vi "VIP_Phase_4.vi"() -> ()   [LabVIEW 2024]
uses:
  <vilib>/DAQmx/read.llb/DAQmx Read (Digital 1D Bool 1Chan 1Samp).vi
  <vilib>/Utility/file.llb/Write To Spreadsheet File (DBL).vi
  <vilib>/DAQmx/create/channels.llb/DAQmx Create Channel (DI-Digital Input).vi
  <vilib>/DAQmx/miscellaneous.llb/DAQmx Fill In Error Info.vi
  <vilib>/ptbypt/NI_PtbyPt.lvlib
panel:
  out "fault # 4":dbl
  out "fault # 3":dbl
  out "fault # 2":dbl
  out "fault # 1":dbl
  in  "LED 4":tag="Dev1/port0/line23"
  in  "LED 3":tag="Dev1/port0/line22"
  in  "LED 2":tag="Dev1/port0/line21"
  out "LED 4 (i)":dbl
  out "LED 3 (i)":dbl
  out "LED 2 (i)":dbl
  in  "LED 1":tag="Dev1/port0/line20"
  out "LED 1(i)":dbl
  out "4.2":bool
  out "mouse 4.2":cluster{"Y":dbl[], "Y":dbl[]}[](graph)
  out "mouse 4.1":cluster{"Y":dbl[], "Y":dbl[]}[](graph)
  in  "fake 4.2":bool
  in  "fake 4.1":bool
  out "ratio 4.2R":cluster{"Y":dbl[], "Y":dbl[]}[](graph)=[{"Y"=[2.5380001068115234, 12.063000202178955, 24.592000007629395, 36.145999908447266, 48.69600009918213, 58.23899984359741, 67.79099988937378, 81.40899991989136, 91.96199989318848, 99.9980001449585], "Y"=[0.0, 0.0, 0.0, 0.0, 0.0, 0.0, 0.0, 0.0, 0.0, 0.0]}]
  out "ratio 4.1L":cluster{"Y":dbl[], "Y":dbl[]}[](graph)=[{"Y"=[2.5380001068115234, 12.063000202178955, 24.592000007629395, 36.145999908447266, 48.69600009918213, 58.23899984359741, 67.79099988937378, 81.40899991989136, 91.96199989318848, 99.9980001449585], "Y"=[0.0, 0.0, 0.0, 0.0, 0.0, 0.0, 0.0, 0.0, 0.0, 0.0]}]
  out "ratio 4.2R":dbl
  out "ratio 4.1L":dbl
  in  "water dur (ms) 4.2":dbl=11.5
  in  "water port 4.2":tag="Dev1/port2/line0"
  out "Mouse path 4":path=path "C:/Users/Administrator/Documents/LabVIEW Data/a-lick-20140707-145848"
  out "Mouse file 4":string="a-lick-20140707-145848"
  in  "Mouse ID 4":string="VIP_4"
  in  "water dur (ms) 4.1":dbl=9.0
  in  "water port 4.1":tag="Dev1/port1/line7"
  in  "free water 4.2":bool
  in  "free water 4.1":bool
  out "4.1":bool
  out "state 4.2":enum16{"waiting", "sound", "ITI"}(ring)=enum."ITI"
  out "state 4.1":enum16{"waiting", "sound", "ITI"}(ring)=enum."ITI"
  out "water # 4.1L":dbl
  out "water # 4.2R":dbl
  out "lick # 4.2R":dbl
  out "lick # 4.1L":dbl
  out "last water 4.2R":dbl
  out "last water 4.1L":dbl
  out "mistake # 4.2R":dbl
  out "mistake # 4.1L":dbl
  out "ratio 3.2R":cluster{"Y":dbl[], "Y":dbl[]}[](graph)=[{"Y"=[2.5380001068115234, 12.063000202178955, 24.592000007629395, 36.145999908447266, 48.69600009918213, 58.23899984359741, 67.79099988937378, 81.40899991989136, 91.96199989318848, 99.9980001449585], "Y"=[0.0, 0.0, 0.0, 0.0, 0.0, 0.0, 0.0, 0.0, 0.0, 0.0]}]
  out "ratio 3.1L":cluster{"Y":dbl[], "Y":dbl[]}[](graph)=[{"Y"=[2.5380001068115234, 12.063000202178955, 24.592000007629395, 36.145999908447266, 48.69600009918213, 58.23899984359741, 67.79099988937378, 81.40899991989136, 91.96199989318848, 99.9980001449585], "Y"=[0.0, 0.0, 0.0, 0.0, 0.0, 0.0, 0.0, 0.0, 0.0, 0.0]}]
  in  "free water 3.2":bool
  in  "free water 3.1":bool
  in  "water dur (ms) 3. 2":dbl=29.0
  in  "water dur (ms) 3.1":dbl=29.0
  out "mouse 3.2":cluster{"Y":dbl[], "Y":dbl[]}[](graph)
  out "mouse 3.1":cluster{"Y":dbl[], "Y":dbl[]}[](graph)
  in  "fake 3.2":bool
  in  "fake 3.1":bool
  out "last water 3.2R":dbl
  out "last water 3.1L":dbl
  out "mistake # 3.2R":dbl
  out "mistake # 3.1L":dbl
  out "water # 3.2R":dbl
  out "water # 3.1L":dbl
  out "lick # 3.2R":dbl
  out "lick # 3.1L":dbl
  out "ratio 3.2R":dbl
  out "ratio 3.1L":dbl
  in  "water port 3.2":tag="Dev1/port1/line6"
  out "3.2":bool
  out "state 3.2":enum16{"waiting", "sound", "ITI"}(ring)=enum."ITI"
  out "state 3.1":enum16{"waiting", "sound", "ITI"}(ring)=enum."ITI"
  out "3.1":bool
  out "Mouse path 3":path=path "C:/Users/Administrator/Documents/LabVIEW Data/a-lick-20140707-145848"
  out "Mouse file 3":string="a-lick-20140707-145848"
  in  "water port 3.1":tag="Dev1/port1/line5"
  in  "Mouse ID 3":string="VIP_3"
  out "ratio 2.2R":cluster{"Y":dbl[], "Y":dbl[]}[](graph)=[{"Y"=[2.5380001068115234, 12.063000202178955, 24.592000007629395, 36.145999908447266, 48.69600009918213, 58.23899984359741, 67.79099988937378, 81.40899991989136, 91.96199989318848, 99.9980001449585], "Y"=[0.0, 0.0, 0.0, 0.0, 0.0, 0.0, 0.0, 0.0, 0.0, 0.0]}]
  out "ratio 2.1L":cluster{"Y":dbl[], "Y":dbl[]}[](graph)=[{"Y"=[2.5380001068115234, 12.063000202178955, 24.592000007629395, 36.145999908447266, 48.69600009918213, 58.23899984359741, 67.79099988937378, 81.40899991989136, 91.96199989318848, 99.9980001449585], "Y"=[0.0, 0.0, 0.0, 0.0, 0.0, 0.0, 0.0, 0.0, 0.0, 0.0]}]
  out "ratio 1.2R":cluster{"Y":dbl[], "Y":dbl[]}[](graph)=[{"Y"=[2.5380001068115234, 12.063000202178955, 24.592000007629395, 36.145999908447266, 48.69600009918213, 58.23899984359741, 67.79099988937378, 81.40899991989136, 91.96199989318848, 99.9980001449585], "Y"=[0.0, 0.0, 0.0, 0.0, 0.0, 0.0, 0.0, 0.0, 0.0, 0.0]}]
  out "mouse 2.2":cluster{"Y":dbl[], "Y":dbl[]}[](graph)
  out "mouse 2.1":cluster{"Y":dbl[], "Y":dbl[]}[](graph)
  in  "free water 2.2":bool
  in  "free water 2.1":bool
  out "last water 2.2R":dbl
  out "last water 2.1L":dbl
  out "mistake # 2.2R":dbl
  out "mistake # 2.1L":dbl
  out "water # 2.2R":dbl
  out "water # 2.1L":dbl
  out "lick  #  2.2R":dbl
  out "lick  #  2.1L":dbl
  out "2.1":bool
  out "ratio 2.2R":dbl
  out "ratio 2.1L":dbl
  out "2.2":bool
  in  "fake 2.2":bool
  in  "fake 2.1":bool
  out "Mouse path 2":path=path "C:/Users/Administrator/Documents/LabVIEW Data/a-lick-20140707-145848"
  out "Mouse file 2":string="a-lick-20140707-145848"
  in  "Mouse ID 2":string="VIP_2"
  in  "water dur (ms) 2.2":dbl=27.5
  in  "water dur (ms) 2.1":dbl=36.5
  in  "water port 2.2":tag="Dev1/port1/line4"
  in  "water port 2.1":tag="Dev1/port1/line3"
  out "state 2.2":enum16{"waiting", "sound", "ITI"}(ring)=enum."ITI"
  out "state 2.1":enum16{"waiting", "sound", "ITI"}(ring)=enum."ITI"
  in  "sound port 2":tag="Dev1/ao1"
  out "time (s)":dbl=103.38100004196167
  out "mistake # 1.2R":dbl
  out "mistake # 1.1L":dbl
  in  "water dur (ms) 1.1":dbl=36.0
  in  "water port 1.1":tag="Dev1/port1/line1"
  in  "water dur (ms) 1.2":dbl=28.0
  in  "water port 1.2":tag="Dev1/port1/line2"
  out "1.1":bool
  out "1.2":bool
  out "state 1.2":enum16{"waiting", "sound", "ITI"}(ring)=enum."ITI"
  out "lick # 1.2R":dbl
  out "water # 1.2R":dbl
  in  "fake 1.2":bool
  in  "free water 1.2":bool
  out "mouse 1.2":cluster{"Y":dbl[], "Y":dbl[]}[](graph)
  out "ratio 1.2R":dbl
  out "last water 1.2R":dbl
  out "ratio 1.1L":dbl
  out "ratio 1.1L":cluster{"Y":dbl[], "Y":dbl[]}[](graph)=[{"Y"=[2.5380001068115234, 12.063000202178955, 24.592000007629395, 36.145999908447266, 48.69600009918213, 58.23899984359741, 67.79099988937378, 81.40899991989136, 91.96199989318848, 99.9980001449585], "Y"=[0.0, 0.0, 0.0, 0.0, 0.0, 0.0, 0.0, 0.0, 0.0, 0.0]}]
  in  "free water 1.1":bool
  out "Right Speaker":dbl=5.0
  out "Left Speaker":dbl=5.0
  in  "sound file 2":path=path "C:/Users/cvm-gritton-lab/Documents/Lab View Programs/Lab View Programs/LabVIEW VIs/Tones/New_Phase_2_Sounds/200k_target2.wav"
  in  "ITI max (ms)":dbl=7000.0
  in  "ITI min (ms)":dbl=5000.0
  in  "reaction dur (ms)":dbl=1750.0
  in  "sound dur (ms)":dbl=3000.0
  in  "sound file 1":path=path "C:/Users/cvm-gritton-lab/Documents/Lab View Programs/Lab View Programs/LabVIEW VIs/Tones/New_Phase_2_Sounds/200k_target1.wav"
  in  "sound port 1":tag="Dev1/ao0"
  out "trial state":T1(ring)=enum."ITI"
  out "trial #":dbl=10.0
  out "current sound":dbl=1.0
  out "next sound":dbl[](array[numeric])
  out "Mouse path 1":path=path "C:/Users/Administrator/Documents/LabVIEW Data/a-lick-20140707-145848"
  in  "fake 1.1":bool
  out "mouse 1.1":cluster{"Y":dbl[], "Y":dbl[]}[](graph)
  out "ITI (s)":dbl=6.5
  out "last water 1.1L":dbl
  out "state 1.1":enum16{"waiting", "sound", "ITI"}(ring)=enum."ITI"
  out "water # 1.1L":dbl
  out "lick # 1.1L":dbl
  out "Mouse file 1":string="a-lick-20140707-145848"
  out "data folder":path=path "C:/LabVIEW VIs/LabVIEW data"
  in  "Mouse ID 1":string="VIP_1"
  in  "lick port":tag="Dev1/port0/line0:7"
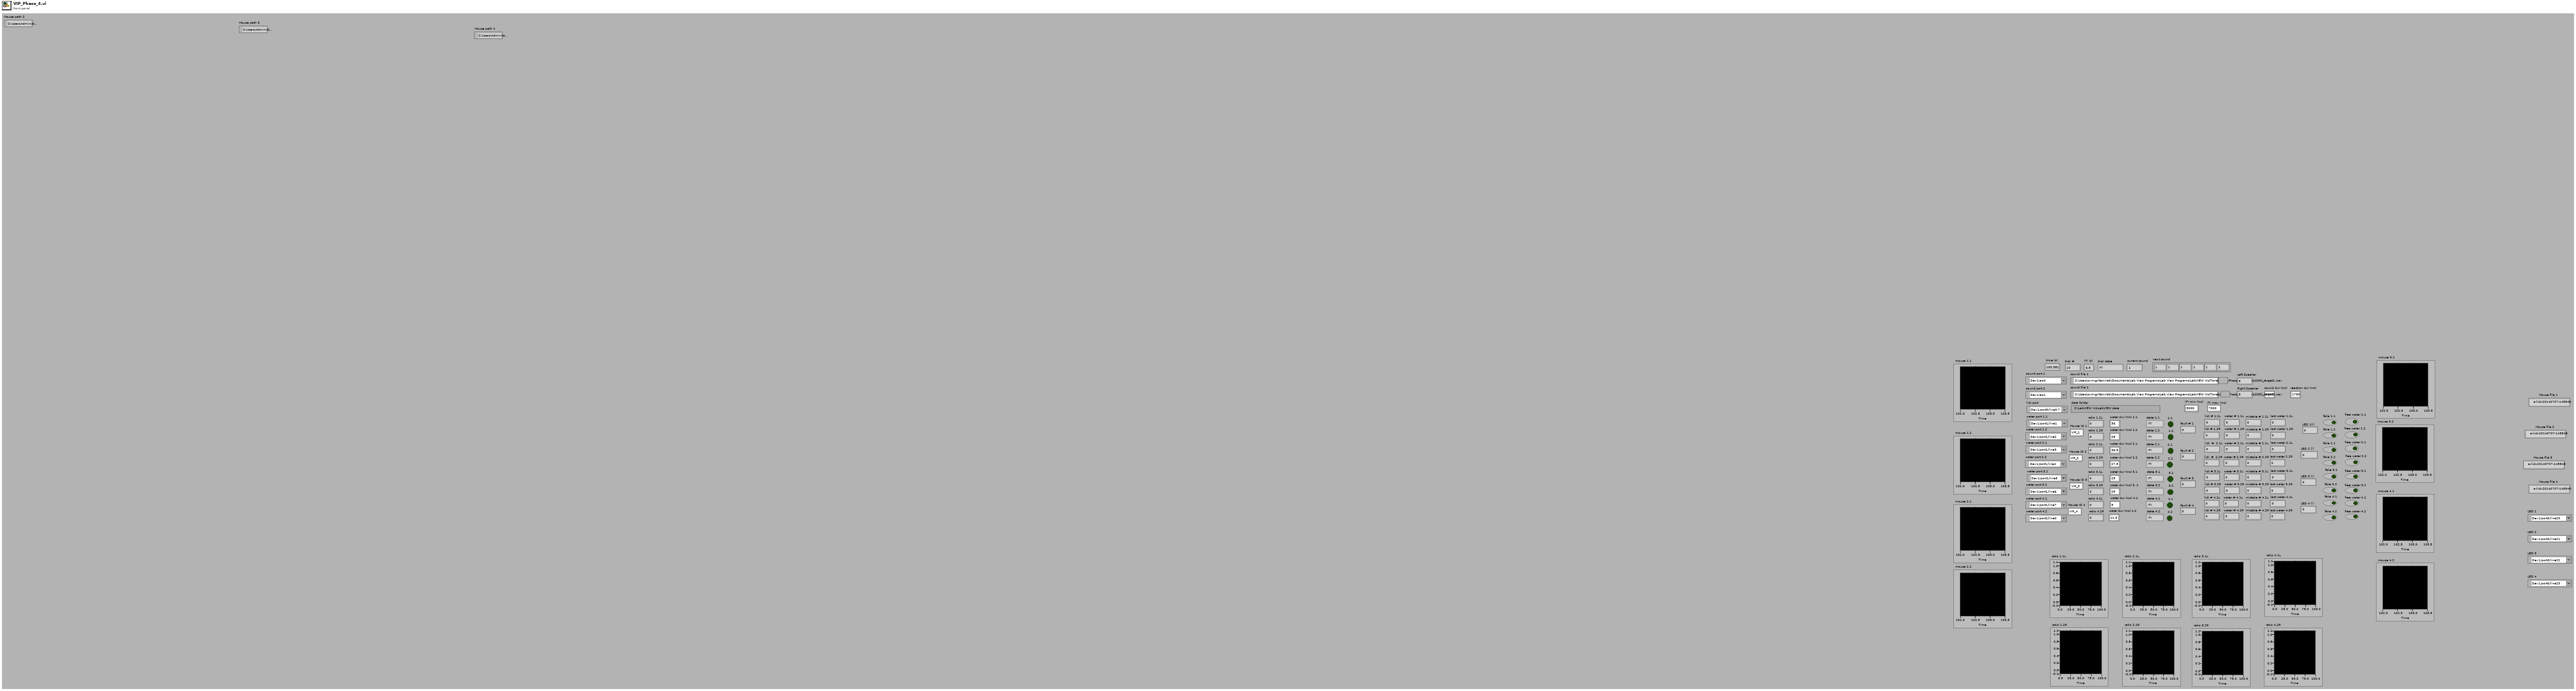
[diagram p1: front panel]
types:
  T1 = enum16{"prepare", "sound", "reaction window", "ITI", "free water", "graph", "data collection"}
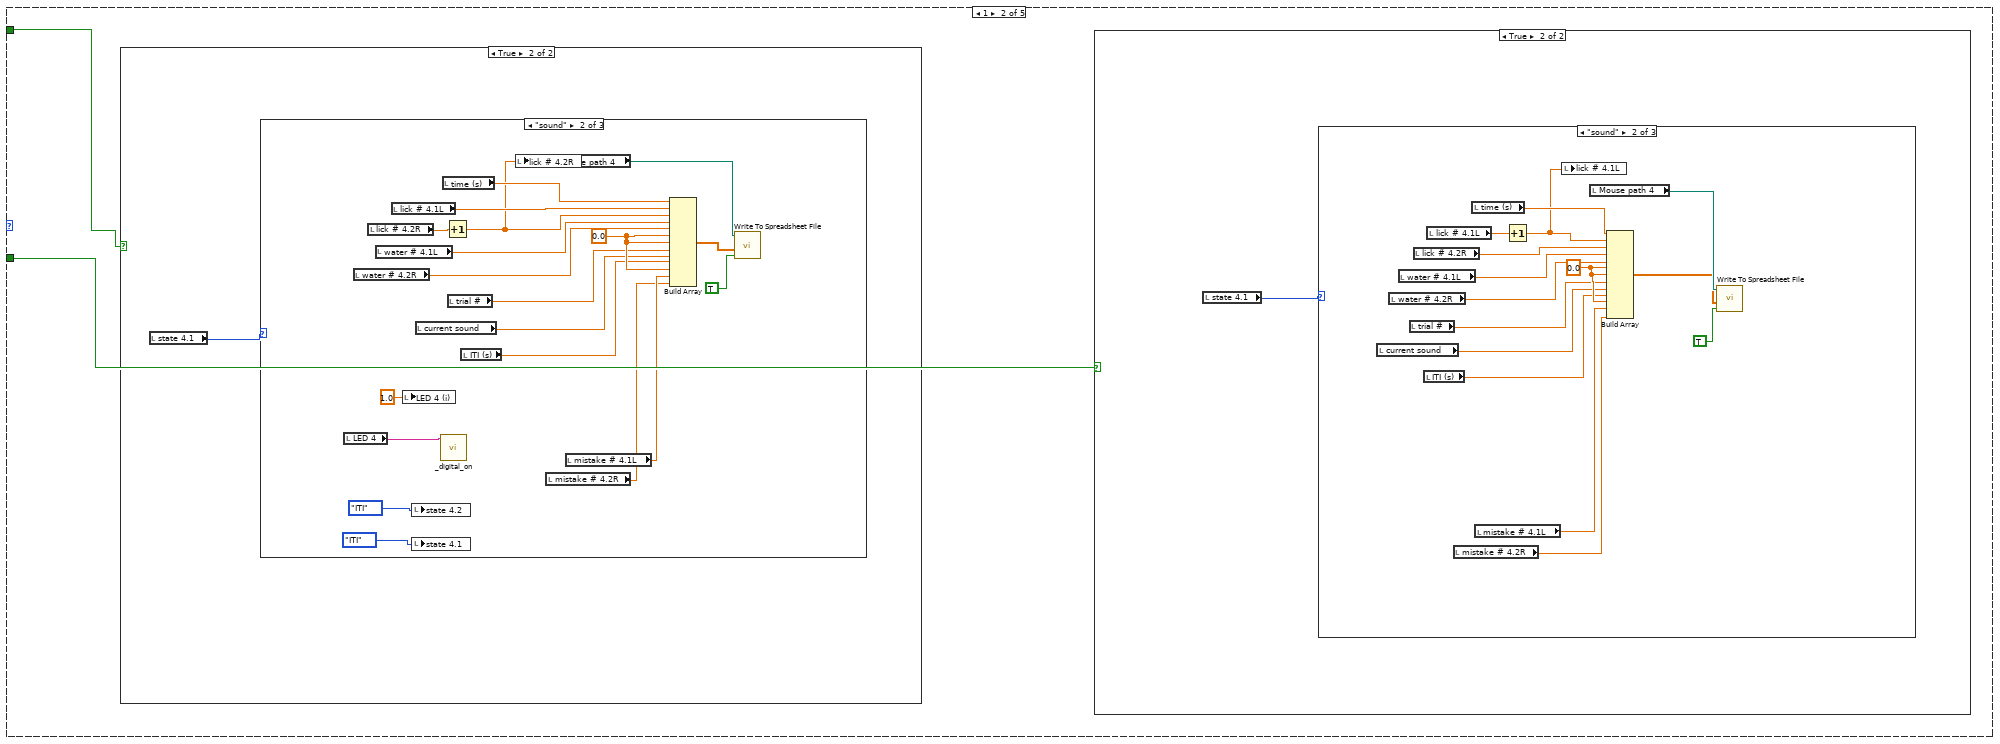
[diagram p3: hidden frame]
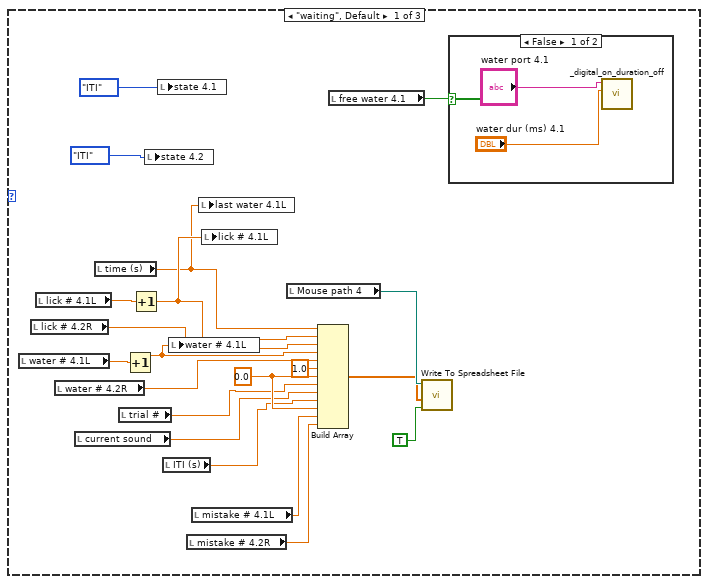
[diagram p5: hidden frame]
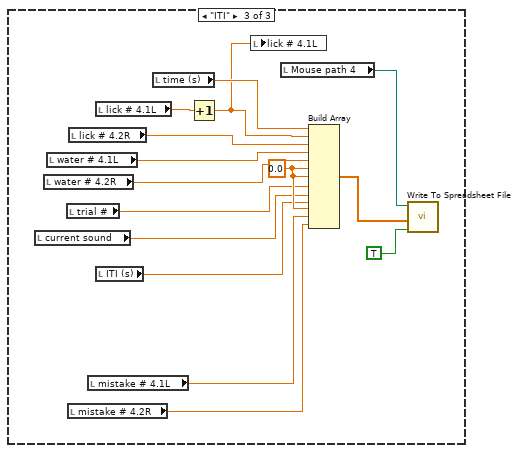
[diagram p7: hidden frame]
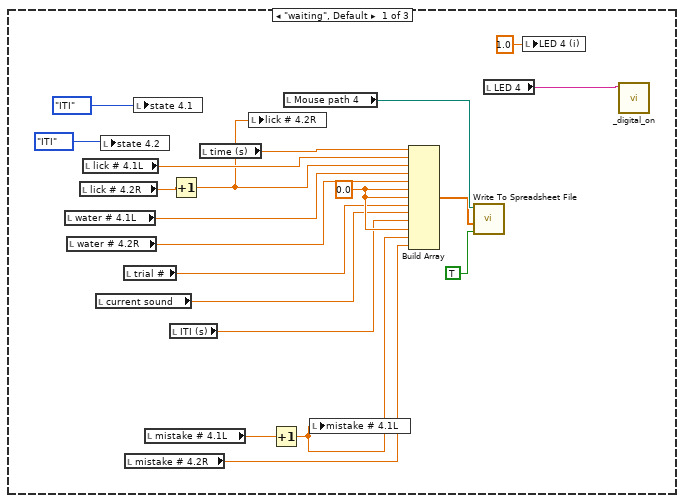
[diagram p9: hidden frame]
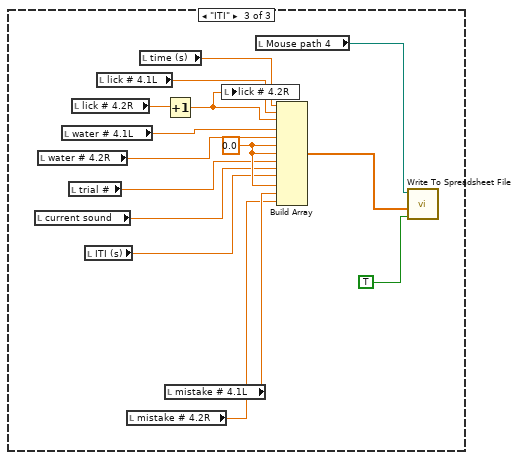
[diagram p10: hidden frame]
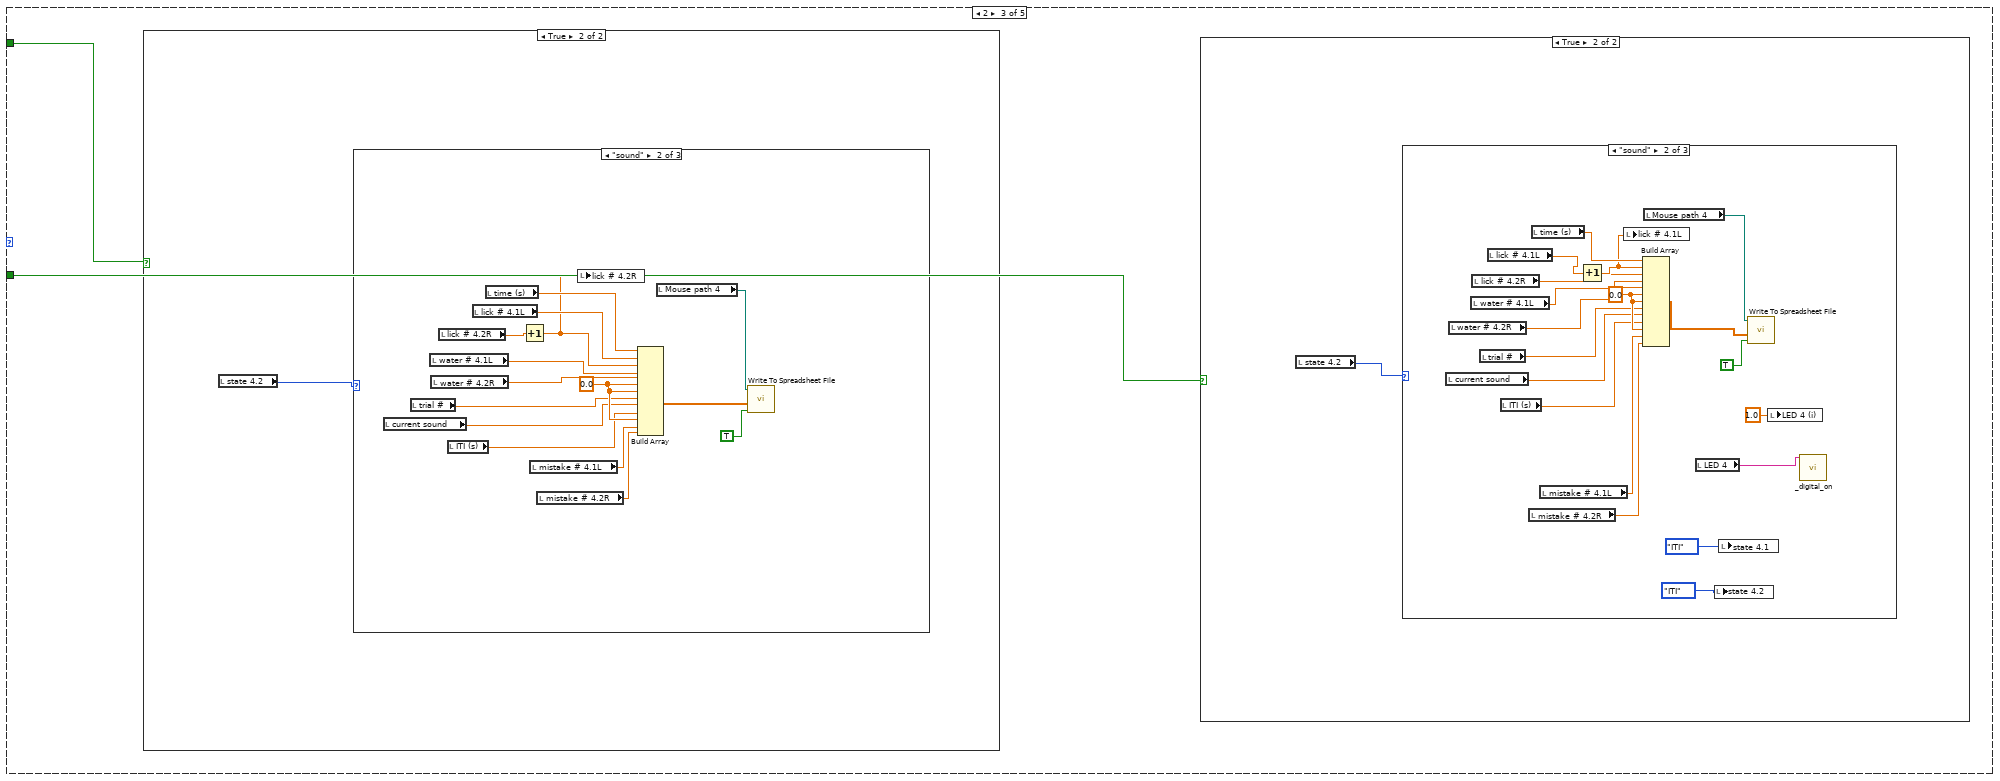
[diagram p11: hidden frame]
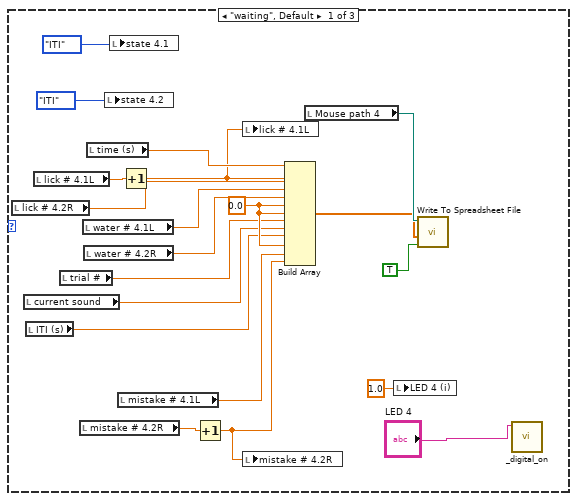
[diagram p13: hidden frame]
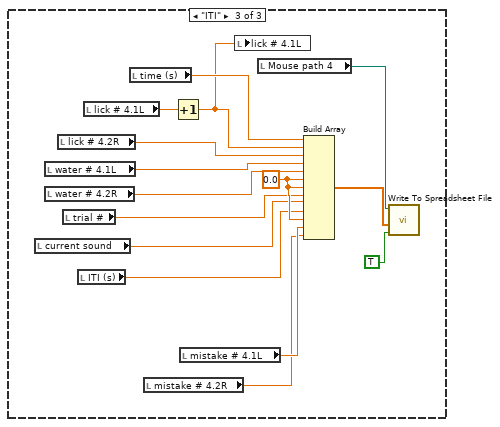
[diagram p14: hidden frame]
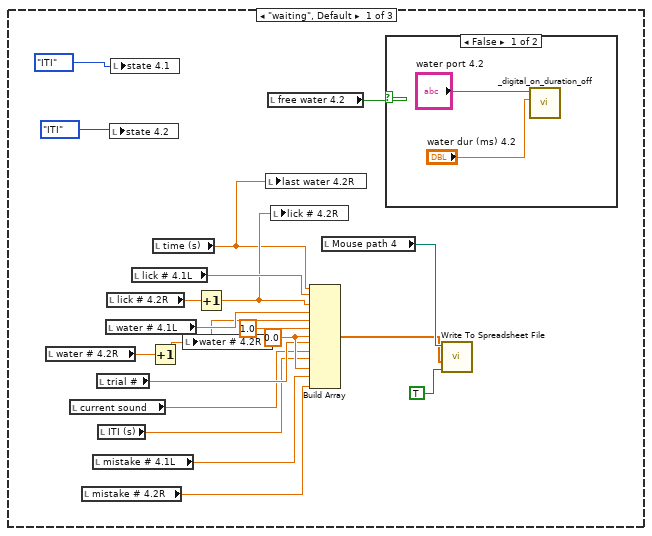
[diagram p16: hidden frame]
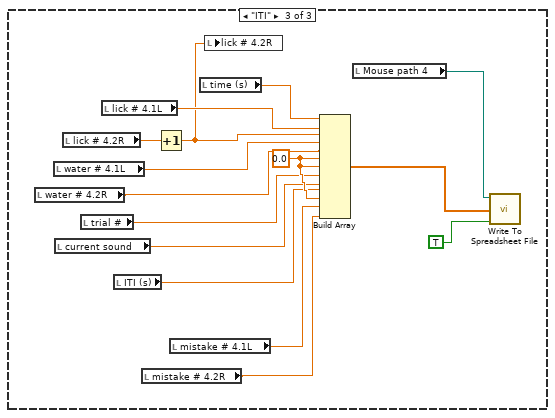
[diagram p18: hidden frame]
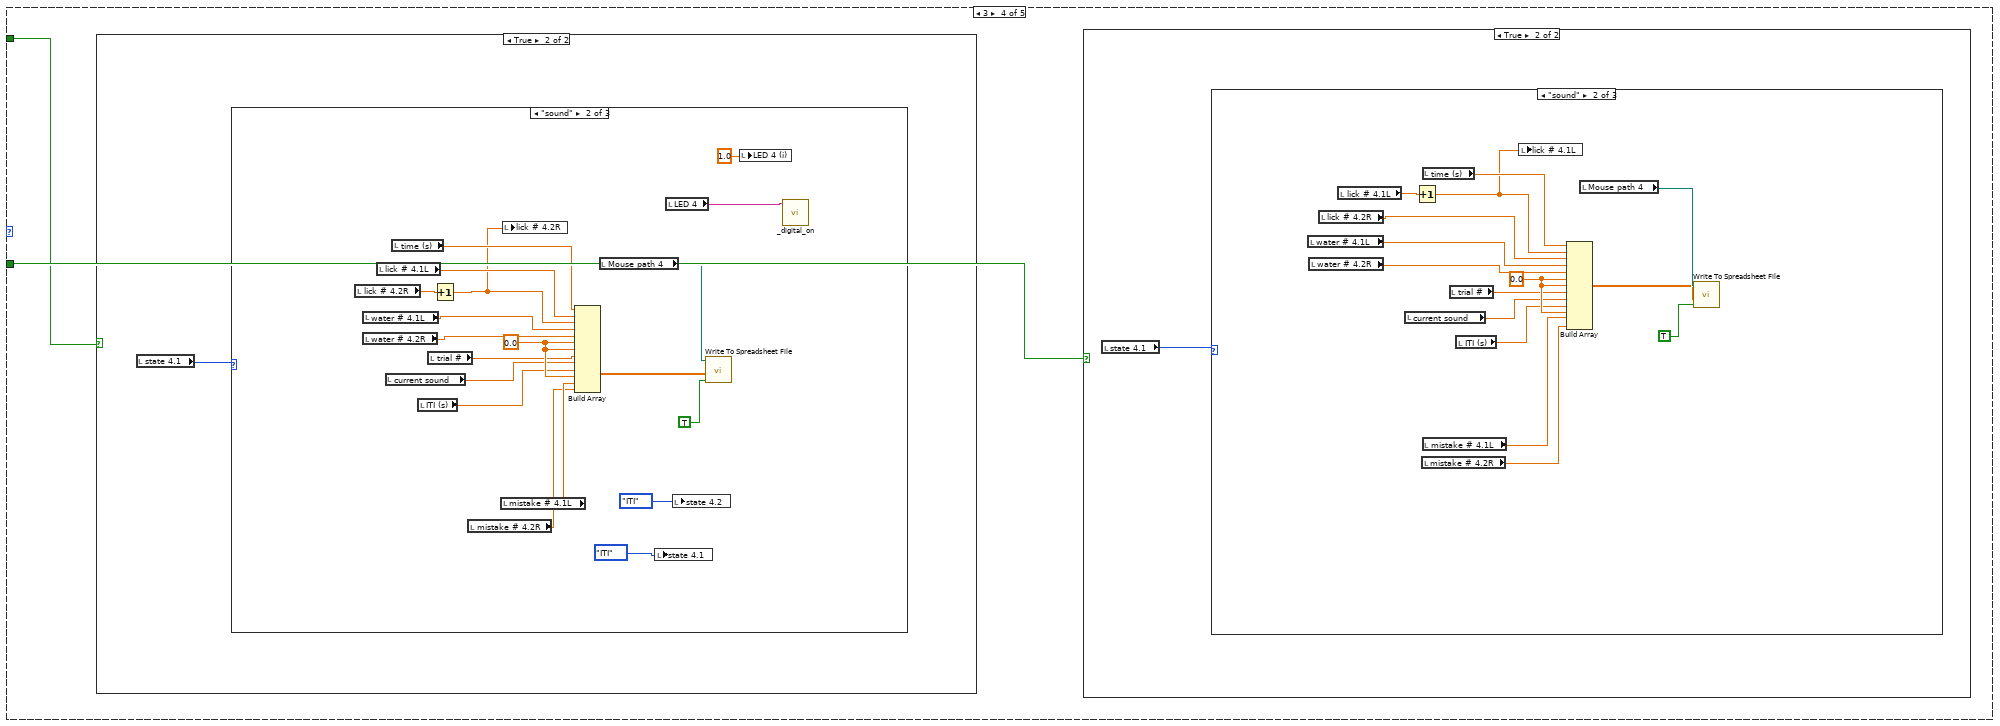
[diagram p19: hidden frame]
diagram:
  n1 = flat-sequence {
    frame #0 {
      w1 = 0.0 ("fault # 2")
      w2 = 0.0 ("LED 1 (R)")
      w12 = 0.0 ("mistake # 1.1L")
      w4 = 0
      w22 = 0
      w11 = 0
      w3 = 0
      w10 = enum16{"waiting", "sound", "ITI"}."sound"
      n2 = Get Date/Time In Seconds() -> (seconds since 1Jan1904=w24:timestamp)
      n3 = call <vilib>:"Dflt Data Dir.vi"() -> ("App:Default Data Directory"=w6:path)
      "data folder" <- w6
      n4 = Format Date/Time String(time format string (%c)="%m%d%Y-%H%M%S-", seconds (now)=w24) -> (date/time string=w9:string)  [unwired: 1 in]
      n5 = Concatenate Strings(w9, "Mouse ID 1") -> (w27:string)
      "Mouse file 1" <- w27
      n6 = Concatenate Strings(w9, "Mouse ID 4") -> (w7:string)
      "Mouse file 4" <- w7
      n7 = Concatenate Strings(w9, "Mouse ID 2") -> (w17:string)
      "Mouse file 2" <- w17
      n8 = Concatenate Strings(w9, "Mouse ID 3") -> (w14:string)
      "Mouse file 3" <- w14
      n9 = Build Path(base path=w6, name or relative path=w27) -> (appended path=→"Mouse path 1":path)
      n10 = Build Path(base path=w6, name or relative path=w17) -> (appended path=→"Mouse path 2":path)
      n11 = Build Path(base path=w6, name or relative path=w14) -> (appended path=→"Mouse path 3":path)
      n12 = Build Path(base path=w6, name or relative path=w7) -> (appended path=→"Mouse path 4":path)
      n13 = call "_array_shuffle.vi"("total number"=40, "input array"=i32[] [1, 2, 3, 4, 1, 2, 3, 4]) -> ("output array"=→"next sound":dbl[])  [unwired: 9 in]
      n14 = local write "time (s)"(w22) -> ()
      "water # 1.1L" <- w3
      "lick # 1.1L" <- w3
      "state 1.1" <- w10
      "last water 1.1L" <- w11
      "current sound" <- w22
      "trial #" <- w22
      "ITI (s)" <- w22
      "Left Speaker" <- w22
      "Right Speaker" <- w22
      "ratio 1.1L" <- w4
      "last water 1.2R" <- w11
      "ratio 1.2R" <- w4
      "water # 1.2R" <- w3
      "lick # 1.2R" <- w3
      "state 1.2" <- w10
      "mistake # 1.1L" <- w12
      "mistake # 1.2R" <- w12
      "state 2.1" <- w10
      "state 2.2" <- w10
      "ratio 2.1L" <- w4
      "ratio 2.2R" <- w4
      "lick  #  2.1L" <- w3
      "lick  #  2.2R" <- w3
      "water # 2.1L" <- w3
      "water # 2.2R" <- w3
      "mistake # 2.1L" <- w12
      "mistake # 2.2R" <- w12
      "last water 2.1L" <- w11
      "last water 2.2R" <- w11
      "state 3.1" <- w10
      "state 3.2" <- w10
      "ratio 3.1L" <- w4
      "ratio 3.2R" <- w4
      "lick # 3.1L" <- w3
      "lick # 3.2R" <- w3
      "water # 3.1L" <- w3
      "water # 3.2R" <- w3
      "mistake # 3.1L" <- w12
      "mistake # 3.2R" <- w12
      "last water 3.1L" <- w11
      "last water 3.2R" <- w11
      "mistake # 4.1L" <- w12
      "mistake # 4.2R" <- w12
      "last water 4.1L" <- w11
      "last water 4.2R" <- w11
      "lick # 4.1L" <- w3
      "lick # 4.2R" <- w3
      "water # 4.2R" <- w3
      "water # 4.1L" <- w3
      "state 4.1" <- w10
      "state 4.2" <- w10
      "ratio 4.1L" <- w4
      "ratio 4.2R" <- w4
      "LED 1(i)" <- w2
      "LED 2 (i)" <- w2
      "LED 3 (i)" <- w2
      "LED 4 (i)" <- w2
      "fault # 1" <- w1
      "fault # 2" <- w1
      "fault # 3" <- w1
      "fault # 4" <- w1
    }
    frame #1 {
      # "file format:\n1. time stamp\n2. lick #\n3. water #\n4. water triggered by lick?\n5. trial start?\n6. trial #\n7. trial sound\n8. trial ITI\n9. free water?"
      n15 = call-poly <vilib>:"DAQmx Create Virtual Channel.vi"("lines"="lick port") -> ("task out"=w29:refnum<k21>)  [unwired: 13 in, 1 out]
      n16 = call <vilib>:"DAQmx Start Task.vi"("task/channels in"=w29) -> ("task out"=w30:refnum<k21>)  [unwired: 13 in, 1 out]
      n17 = while {
        tunnel: w30 -> [w89]
        tunnel: [w88] -> w31
        shift-right: [w79] -> _
        shift-left: _ -> [w87]
        shift-right: [w84] -> _
        shift-left: _ -> [w85]
        stop <- FALSE stop-if-true
        n18 = call-poly <vilib>:"DAQmx Read.vi"("task/channels in"=w89) -> ("task out"=w88:refnum<k21>, "data"=w80:bool[])  [unwired: 12 in, 1 out]
        n19 = Build Array("fake 1.1", "fake 1.2", "fake 2.1", "fake 2.2", "fake 3.1", "fake 3.2", "fake 4.1", "fake 4.2") -> (w76:bool[])
        n20 = Or(x=w80, y=w76) -> (x .or. y?=w79:bool[])
        n21 = Index Array(array=w79) -> (element #1=w82:bool, element #2=w68:bool, element #3=w59:bool, element #4=w56:bool, element #5=w48:bool, element #6=w45:bool, element #7=w40:bool, element #8=w36:bool)  [unwired: 8 in]
        n22 = call "Collector1."("Signals"=w59) -> ("Collected Signals"=w60:dynamicdata)  [unwired: 9 in, 1 out]
        n23 = call "Collector1.2"("Signals"=w68) -> ("Collected Signals"=w67:dynamicdata)  [unwired: 9 in, 1 out]
        n24 = call "Collector1.7"("Signals"=w36) -> ("Collected Signals"=w38:dynamicdata)  [unwired: 9 in, 1 out]
        n25 = call "Collector1.3"("Signals"=w56) -> ("Collected Signals"=w57:dynamicdata)  [unwired: 9 in, 1 out]
        n26 = call "Collector1.6"("Signals"=w40) -> ("Collected Signals"=w41:dynamicdata)  [unwired: 9 in, 1 out]
        n27 = call "Collector1.1"("Signals"=w82) -> ("Collected Signals"=w69:dynamicdata)  [unwired: 9 in, 1 out]
        n28 = call "Collector1.5"("Signals"=w45) -> ("Collected Signals"=w46:dynamicdata)  [unwired: 9 in, 1 out]
        n29 = call "Collector1.4"("Signals"=w48) -> ("Collected Signals"=w49:dynamicdata)  [unwired: 9 in, 1 out]
        n30 = local read "time (s)"() -> (w83:dbl)
        n31 = call "Collector"("Signals"=w83) -> ("Collected Signals"=w35:dynamicdata)  [unwired: 9 in, 1 out]
        n32 = call "Build XY Graph1.1"("Y Input"=w69, "X Input"=w35) -> ("XY Graph"=→"mouse 1.1":cluster{"Y":dbl[], "Y":dbl[]}[])  [unwired: 3 in, 6 out]
        n33 = call "Build XY Graph1."("Y Input"=w60, "X Input"=w35) -> ("XY Graph"=→"mouse 2.1":cluster{"Y":dbl[], "Y":dbl[]}[])  [unwired: 3 in, 6 out]
        n34 = call "Build XY Graph1.2"("Y Input"=w67, "X Input"=w35) -> ("XY Graph"=→"mouse 1.2":cluster{"Y":dbl[], "Y":dbl[]}[])  [unwired: 3 in, 6 out]
        n35 = call "Build XY Graph1.7"("Y Input"=w38, "X Input"=w35) -> ("XY Graph"=→"mouse 4.2":cluster{"Y":dbl[], "Y":dbl[]}[])  [unwired: 3 in, 6 out]
        n36 = call "Build XY Graph1.3"("Y Input"=w57, "X Input"=w35) -> ("XY Graph"=→"mouse 2.2":cluster{"Y":dbl[], "Y":dbl[]}[])  [unwired: 3 in, 6 out]
        n37 = call "Build XY Graph1.6"("Y Input"=w41, "X Input"=w35) -> ("XY Graph"=→"mouse 4.1":cluster{"Y":dbl[], "Y":dbl[]}[])  [unwired: 3 in, 6 out]
        n38 = call "Build XY Graph1.5"("Y Input"=w46, "X Input"=w35) -> ("XY Graph"=→"mouse 3.2":cluster{"Y":dbl[], "Y":dbl[]}[])  [unwired: 3 in, 6 out]
        n39 = call "Build XY Graph1.4"("Y Input"=w49, "X Input"=w35) -> ("XY Graph"=→"mouse 3.1":cluster{"Y":dbl[], "Y":dbl[]}[])  [unwired: 3 in, 6 out]
        n40 = Greater?(x=w79, y=w87) -> (0:w86:bool[])
        n41 = Index Array(array=w86) -> (element #1=w74:bool, element #2=w73:bool, element #3=w62:bool, element #4=w63:bool, element #5=w54:bool, element #6=w53:bool, element #7=w33:bool, element #8=w34:bool)  [unwired: 8 in]
        "1.2" <- w73
        "1.1" <- w74
        "2.2" <- w63
        "2.1" <- w62
        "3.1" <- w54
        "3.2" <- w53
        "4.1" <- w33
        "4.2" <- w34
        n42 = local read "current sound"() -> (w72:dbl)
        n43 = local read "current sound"() -> (w66:dbl)
        n44 = local read "current sound"() -> (w44:dbl)
        n45 = local read "current sound"() -> (w55:dbl)
        n46 = case shown="4" w55 {
          tunnel: w54 -> [_ w531 w642 w752 w862]
          tunnel: w53 -> [_ w530 w641 w751 w861]
          frame 0, Default {
          }
          frame 1 {
            n47 = case shown="True" w531 {
              frame False {
              }
              frame True {
                n48 = local read "state 3.1"() -> (w588:enum16{"waiting", "sound", "ITI"})
                n49 = case shown="\"waiting\", Default" w588 {
                  frame "waiting", Default {
                    w597 = 0.0 ("element")
                    n50 = local write "state 3.2"(enum16{"waiting", "sound", "ITI"}."ITI") -> ()
                    n51 = local read "free water 3.1"() -> (w608:bool)
                    n52 = local write "state 3.1"(enum16{"waiting", "sound", "ITI"}."ITI") -> ()
                    n53 = local read "water # 3.1L"() -> (w600:dbl)
                    n54 = local read "lick # 3.2R"() -> (w601:dbl)
                    n55 = local read "lick # 3.1L"() -> (w603:dbl)
                    n56 = local read "water # 3.2R"() -> (w598:dbl)
                    n57 = local read "current sound"() -> (w590:dbl)
                    n58 = case shown="False" w608 {
                      frame False {
                        n59 = call "_digital_on_duration_off.vi"("duration (ms)"="water dur (ms) 3.1", "digital port"="water port 3.1") -> ()  [unwired: 10 in]
                      }
                      frame True {
                      }
                    }
                    n60 = local read "mistake # 3.2R"() -> (w595:dbl)
                    n61 = local read "mistake # 3.1L"() -> (w596:dbl)
                    n62 = local read "ITI (s)"() -> (w589:dbl)
                    n63 = local read "trial #"() -> (w591:dbl)
                    n64 = Increment(x=w600) -> (x+1=w599:dbl)
                    n65 = Increment(x=w603) -> (x+1=w602:dbl)
                    n66 = local read "time (s)"() -> (w604:dbl)
                    n67 = local write "water # 3.1L"(w599) -> ()
                    n68 = local write "lick # 3.1L"(w602) -> ()
                    n69 = local write "last water 3.1L"(w604) -> ()
                    n70 = local read "Mouse path 3"() -> (w607:path)
                    n71 = Build Array(w604, w602, w601, w599, w598, 1.0 ("element"), w597, w591, w590, w589, w597, w596, w595) -> (w605:dbl[])
                    n72 = call-poly <vilib>:"Write To Spreadsheet File.vi"("append to file? (new file:F)"=TRUE, "1D data"=w605, "file path (dialog if empty)"=w607) -> ()  [unwired: 5 in, 1 out]
                  }
                  frame "sound" {
                    w616 = 0.0 ("element")
                    n73 = local read "current sound"() -> (w612:dbl)
                    n74 = local read "trial #"() -> (w613:dbl)
                    n75 = local read "water # 3.2R"() -> (w617:dbl)
                    n76 = local read "water # 3.1L"() -> (w618:dbl)
                    n77 = local read "mistake # 3.2R"() -> (w614:dbl)
                    n78 = local read "lick # 3.2R"() -> (w619:dbl)
                    n79 = local read "lick # 3.1L"() -> (w621:dbl)
                    n80 = local read "ITI (s)"() -> (w611:dbl)
                    n81 = local read "mistake # 3.1L"() -> (w615:dbl)
                    n82 = local read "time (s)"() -> (w622:dbl)
                    n83 = Increment(x=w621) -> (x+1=w620:dbl)
                    n84 = local write "lick # 3.1L"(w620) -> ()
                    n85 = local read "Mouse path 3"() -> (w625:path)
                    n86 = Build Array(w622, w620, w619, w618, w617, w616, w616, w613, w612, w611, w616, w615, w614) -> (w623:dbl[])
                    n87 = call-poly <vilib>:"Write To Spreadsheet File.vi"("append to file? (new file:F)"=TRUE, "1D data"=w623, "file path (dialog if empty)"=w625) -> ()  [unwired: 5 in, 1 out]
                  }
                  frame "ITI" {
                    w631 = 0.0 ("element")
                    n88 = local read "water # 3.2R"() -> (w632:dbl)
                    n89 = local read "current sound"() -> (w627:dbl)
                    n90 = local read "lick # 3.2R"() -> (w634:dbl)
                    n91 = local read "lick # 3.1L"() -> (w636:dbl)
                    n92 = local read "water # 3.1L"() -> (w633:dbl)
                    n93 = local read "trial #"() -> (w628:dbl)
                    n94 = local read "ITI (s)"() -> (w626:dbl)
                    n95 = local read "time (s)"() -> (w637:dbl)
                    n96 = Increment(x=w636) -> (x+1=w635:dbl)
                    n97 = local read "mistake # 3.1L"() -> (w630:dbl)
                    n98 = local read "mistake # 3.2R"() -> (w629:dbl)
                    n99 = local write "lick # 3.1L"(w635) -> ()
                    n100 = local read "Mouse path 3"() -> (w640:path)
                    n101 = Build Array(w637, w635, w634, w633, w632, w631, w631, w628, w627, w626, w631, w630, w629) -> (w638:dbl[])
                    n102 = call-poly <vilib>:"Write To Spreadsheet File.vi"("append to file? (new file:F)"=TRUE, "1D data"=w638, "file path (dialog if empty)"=w640) -> ()  [unwired: 5 in, 1 out]
                  }
                }
              }
            }
            n103 = case shown="True" w530 {
              frame False {
              }
              frame True {
                n104 = local read "state 3.1"() -> (w532:enum16{"waiting", "sound", "ITI"})
                n105 = case shown="\"sound\"" w532 {
                  frame "waiting", Default {
                    w542 = 0.0 ("element")
                    n106 = local read "mistake # 3.1L"() -> (w541:dbl)
                    n107 = local write "state 3.2"(enum16{"waiting", "sound", "ITI"}."ITI") -> ()
                    n108 = local write "state 3.1"(enum16{"waiting", "sound", "ITI"}."ITI") -> ()
                    n109 = Increment(x=w541) -> (x+1=w540:dbl)
                    n110 = local read "water # 3.2R"() -> (w543:dbl)
                    n111 = local read "water # 3.1L"() -> (w544:dbl)
                    n112 = local read "lick # 3.2R"() -> (w546:dbl)
                    n113 = local read "current sound"() -> (w535:dbl)
                    n114 = local read "mistake # 3.2R"() -> (w539:dbl)
                    n115 = local write "mistake # 3.1L"(w540) -> ()
                    n116 = local read "lick # 3.1L"() -> (w547:dbl)
                    n117 = local read "ITI (s)"() -> (w534:dbl)
                    n118 = local read "trial #"() -> (w536:dbl)
                    n119 = local read "time (s)"() -> (w548:dbl)
                    n120 = Increment(x=w546) -> (x+1=w545:dbl)
                    n121 = local write "lick # 3.2R"(w545) -> ()
                    n122 = Build Array(w548, w547, w545, w544, w543, w542, w542, w536, w535, w534, w542, w540, w539) -> (w549:dbl[])
                    n123 = local read "Mouse path 3"() -> (w551:path)
                    n124 = call "_digital_on.vi"("digital port"="LED 3") -> ()  [unwired: 11 in]
                    n125 = call-poly <vilib>:"Write To Spreadsheet File.vi"("append to file? (new file:F)"=TRUE, "1D data"=w549, "file path (dialog if empty)"=w551) -> ()  [unwired: 5 in, 1 out]
                    n126 = local write "LED 3 (i)"(1.0 ("LED 3 (i)")) -> ()
                    n127 = local write "state 3.2"(enum16{"waiting", "sound", "ITI"}."ITI") -> ()
                  }
                  frame "sound" {
                    w563 = 0.0 ("element")
                    n128 = local read "LED 3"() -> (w556:tag)
                    n129 = local write "LED 3 (i)"(1.0 ("LED 3 (i)")) -> ()
                    n130 = local read "water # 3.1L"() -> (w565:dbl)
                    n131 = local read "lick # 3.2R"() -> (w567:dbl)
                    n132 = local read "water # 3.2R"() -> (w564:dbl)
                    n133 = local read "lick # 3.1L"() -> (w568:dbl)
                    n134 = local read "current sound"() -> (w559:dbl)
                    n135 = local read "trial #"() -> (w560:dbl)
                    n136 = local read "time (s)"() -> (w569:dbl)
                    n137 = Increment(x=w567) -> (x+1=w566:dbl)
                    n138 = local read "ITI (s)"() -> (w558:dbl)
                    n139 = call "_digital_on.vi"("digital port"=w556) -> ()  [unwired: 11 in]
                    n140 = local read "mistake # 3.2R"() -> (w561:dbl)
                    n141 = local read "mistake # 3.1L"() -> (w562:dbl)
                    n142 = local write "lick # 3.2R"(w566) -> ()
                    n143 = local write "state 3.1"(enum16{"waiting", "sound", "ITI"}."ITI") -> ()
                    n144 = local write "state 3.2"(enum16{"waiting", "sound", "ITI"}."ITI") -> ()
                    n145 = local read "Mouse path 3"() -> (w571:path)
                    n146 = Build Array(w569, w568, w566, w565, w564, w563, w563, w560, w559, w558, w563, w562, w561) -> (w570:dbl[])
                    n147 = call-poly <vilib>:"Write To Spreadsheet File.vi"("append to file? (new file:F)"=TRUE, "1D data"=w570, "file path (dialog if empty)"=w571) -> ()  [unwired: 5 in, 1 out]
                  }
                  frame "ITI" {
                    w578 = 0.0 ("element")
                    n148 = local read "water # 3.2R"() -> (w579:dbl)
                    n149 = local read "water # 3.1L"() -> (w580:dbl)
                    n150 = local read "lick # 3.2R"() -> (w582:dbl)
                    n151 = local read "current sound"() -> (w574:dbl)
                    n152 = local read "lick # 3.1L"() -> (w583:dbl)
                    n153 = local read "trial #"() -> (w575:dbl)
                    n154 = Increment(x=w582) -> (x+1=w581:dbl)
                    n155 = local read "time (s)"() -> (w584:dbl)
                    n156 = local read "mistake # 3.2R"() -> (w576:dbl)
                    n157 = local read "ITI (s)"() -> (w573:dbl)
                    n158 = local read "mistake # 3.1L"() -> (w577:dbl)
                    n159 = local write "lick # 3.2R"(w581) -> ()
                    n160 = local read "Mouse path 3"() -> (w586:path)
                    n161 = Build Array(w584, w583, w581, w580, w579, w578, w578, w575, w574, w573, w578, w577, w576) -> (w585:dbl[])
                    n162 = call-poly <vilib>:"Write To Spreadsheet File.vi"("append to file? (new file:F)"=TRUE, "1D data"=w585, "file path (dialog if empty)"=w586) -> ()  [unwired: 5 in, 1 out]
                  }
                }
              }
            }
          }
          frame 2 {
            n163 = case shown="True" w642 {
              frame False {
              }
              frame True {
                n164 = local read "state 3.2"() -> (w696:enum16{"waiting", "sound", "ITI"})
                n165 = case shown="\"sound\"" w696 {
                  frame "waiting", Default {
                    w705 = 0.0 ("element")
                    n166 = local read "water # 3.2R"() -> (w706:dbl)
                    n167 = local read "water # 3.1L"() -> (w707:dbl)
                    n168 = local read "lick # 3.2R"() -> (w708:dbl)
                    n169 = local read "lick # 3.1L"() -> (w710:dbl)
                    n170 = local read "current sound"() -> (w698:dbl)
                    n171 = local write "state 3.2"(enum16{"waiting", "sound", "ITI"}."ITI") -> ()
                    n172 = local read "trial #"() -> (w699:dbl)
                    n173 = local read "ITI (s)"() -> (w697:dbl)
                    n174 = local read "mistake # 3.1L"() -> (w704:dbl)
                    n175 = local read "time (s)"() -> (w711:dbl)
                    n176 = local read "mistake # 3.2R"() -> (w703:dbl)
                    n177 = local write "state 3.1"(enum16{"waiting", "sound", "ITI"}."ITI") -> ()
                    n178 = Increment(x=w710) -> (x+1=w709:dbl)
                    n179 = local write "lick # 3.1L"(w709) -> ()
                    n180 = local read "Mouse path 3"() -> (w713:path)
                    n181 = Increment(x=w703) -> (x+1=w702:dbl)
                    n182 = local write "mistake # 3.2R"(w702) -> ()
                    n183 = Build Array(w711, w709, w708, w707, w706, w705, w705, w699, w698, w697, w705, w704, w702) -> (w712:dbl[])
                    n184 = local read "LED 3"() -> (w701:tag)
                    n185 = call-poly <vilib>:"Write To Spreadsheet File.vi"("append to file? (new file:F)"=TRUE, "1D data"=w712, "file path (dialog if empty)"=w713) -> ()  [unwired: 5 in, 1 out]
                    n186 = local write "LED 3 (i)"(1.0 ("LED 3 (i)")) -> ()
                    n187 = call "_digital_on.vi"("digital port"=w701) -> ()  [unwired: 11 in]
                  }
                  frame "sound" {
                    w726 = 0.0 ("element")
                    n188 = local read "current sound"() -> (w722:dbl)
                    n189 = local read "water # 3.2R"() -> (w727:dbl)
                    n190 = local read "water # 3.1L"() -> (w728:dbl)
                    n191 = local read "trial #"() -> (w723:dbl)
                    n192 = local read "lick # 3.2R"() -> (w729:dbl)
                    n193 = local read "lick # 3.1L"() -> (w731:dbl)
                    n194 = local read "ITI (s)"() -> (w721:dbl)
                    n195 = local read "mistake # 3.2R"() -> (w724:dbl)
                    n196 = local read "time (s)"() -> (w732:dbl)
                    n197 = local read "mistake # 3.1L"() -> (w725:dbl)
                    n198 = Increment(x=w731) -> (x+1=w730:dbl)
                    n199 = local write "lick # 3.1L"(w730) -> ()
                    n200 = local read "Mouse path 3"() -> (w734:path)
                    n201 = Build Array(w732, w730, w729, w728, w727, w726, w726, w723, w722, w721, w726, w725, w724) -> (w733:dbl[])
                    n202 = local read "LED 3"() -> (w719:tag)
                    n203 = call-poly <vilib>:"Write To Spreadsheet File.vi"("append to file? (new file:F)"=TRUE, "1D data"=w733, "file path (dialog if empty)"=w734) -> ()  [unwired: 5 in, 1 out]
                    n204 = local write "LED 3 (i)"(1.0 ("LED 3 (i)")) -> ()
                    n205 = local write "state 3.1"(enum16{"waiting", "sound", "ITI"}."ITI") -> ()
                    n206 = local write "state 3.2"(enum16{"waiting", "sound", "ITI"}."ITI") -> ()
                    n207 = call "_digital_on.vi"("digital port"=w719) -> ()  [unwired: 11 in]
                  }
                  frame "ITI" {
                    w741 = 0.0 ("element")
                    n208 = local read "current sound"() -> (w737:dbl)
                    n209 = local read "water # 3.2R"() -> (w742:dbl)
                    n210 = local read "water # 3.1L"() -> (w743:dbl)
                    n211 = local read "lick # 3.2R"() -> (w744:dbl)
                    n212 = local read "trial #"() -> (w738:dbl)
                    n213 = local read "lick # 3.1L"() -> (w746:dbl)
                    n214 = local read "ITI (s)"() -> (w736:dbl)
                    n215 = local read "mistake # 3.2R"() -> (w739:dbl)
                    n216 = local read "time (s)"() -> (w747:dbl)
                    n217 = local read "mistake # 3.1L"() -> (w740:dbl)
                    n218 = Increment(x=w746) -> (x+1=w745:dbl)
                    n219 = local write "lick # 3.1L"(w745) -> ()
                    n220 = local read "Mouse path 3"() -> (w749:path)
                    n221 = Build Array(w747, w745, w744, w743, w742, w741, w741, w738, w737, w736, w741, w740, w739) -> (w748:dbl[])
                    n222 = call-poly <vilib>:"Write To Spreadsheet File.vi"("append to file? (new file:F)"=TRUE, "1D data"=w748, "file path (dialog if empty)"=w749) -> ()  [unwired: 5 in, 1 out]
                  }
                }
              }
            }
            n223 = case shown="True" w641 {
              frame False {
              }
              frame True {
                n224 = local read "state 3.2"() -> (w643:enum16{"waiting", "sound", "ITI"})
                n225 = case shown="\"waiting\", Default" w643 {
                  frame "waiting", Default {
                    w651 = 0.0 ("element")
                    n226 = local read "water # 3.2R"() -> (w653:dbl)
                    n227 = local read "current sound"() -> (w645:dbl)
                    n228 = local read "lick # 3.2R"() -> (w656:dbl)
                    n229 = local read "water # 3.1L"() -> (w654:dbl)
                    n230 = local read "trial #"() -> (w646:dbl)
                    n231 = local read "mistake # 3.2R"() -> (w649:dbl)
                    n232 = local write "state 3.1"(enum16{"waiting", "sound", "ITI"}."ITI") -> ()
                    n233 = local write "state 3.2"(enum16{"waiting", "sound", "ITI"}."ITI") -> ()
                    n234 = local read "ITI (s)"() -> (w644:dbl)
                    n235 = local read "lick # 3.1L"() -> (w657:dbl)
                    n236 = local read "mistake # 3.1L"() -> (w650:dbl)
                    n237 = local read "time (s)"() -> (w648:dbl)
                    n238 = Increment(x=w653) -> (x+1=w652:dbl)
                    n239 = Increment(x=w656) -> (x+1=w655:dbl)
                    n240 = local read "free water 3.2"() -> (w663:bool)
                    n241 = local write "water # 3.2R"(w652) -> ()
                    n242 = local write "last water 3.2R"(w648) -> ()
                    n243 = local write "lick # 3.2R"(w655) -> ()
                    n244 = local read "Mouse path 3"() -> (w659:path)
                    n245 = Build Array(w648, w657, w655, w654, w652, 1.0 ("element"), w651, w646, w645, w644, w651, w650, w649) -> (w658:dbl[])
                    n246 = case shown="False" w663 {
                      frame False {
                        n247 = call "_digital_on_duration_off.vi"("duration (ms)"="water dur (ms) 3. 2", "digital port"="water port 3.2") -> ()  [unwired: 10 in]
                      }
                      frame True {
                      }
                    }
                    n248 = call-poly <vilib>:"Write To Spreadsheet File.vi"("append to file? (new file:F)"=TRUE, "1D data"=w658, "file path (dialog if empty)"=w659) -> ()  [unwired: 5 in, 1 out]
                  }
                  frame "sound" {
                    w671 = 0.0 ("element")
                    n249 = local read "lick # 3.2R"() -> (w675:dbl)
                    n250 = local read "water # 3.1L"() -> (w673:dbl)
                    n251 = local read "current sound"() -> (w667:dbl)
                    n252 = local read "trial #"() -> (w668:dbl)
                    n253 = local read "water # 3.2R"() -> (w672:dbl)
                    n254 = local read "lick # 3.1L"() -> (w676:dbl)
                    n255 = local read "ITI (s)"() -> (w666:dbl)
                    n256 = local read "mistake # 3.2R"() -> (w669:dbl)
                    n257 = Increment(x=w675) -> (x+1=w674:dbl)
                    n258 = local read "mistake # 3.1L"() -> (w670:dbl)
                    n259 = local read "time (s)"() -> (w677:dbl)
                    n260 = local write "lick # 3.2R"(w674) -> ()
                    n261 = local read "Mouse path 3"() -> (w680:path)
                    n262 = Build Array(w677, w676, w674, w673, w672, w671, w671, w668, w667, w666, w671, w670, w669) -> (w678:dbl[])
                    n263 = call-poly <vilib>:"Write To Spreadsheet File.vi"("append to file? (new file:F)"=TRUE, "1D data"=w678, "file path (dialog if empty)"=w680) -> ()  [unwired: 5 in, 1 out]
                  }
                  frame "ITI" {
                    w686 = 0.0 ("element")
                    n264 = local read "water # 3.2R"() -> (w687:dbl)
                    n265 = local read "lick # 3.2R"() -> (w690:dbl)
                    n266 = local read "current sound"() -> (w682:dbl)
                    n267 = local read "water # 3.1L"() -> (w688:dbl)
                    n268 = local read "lick # 3.1L"() -> (w691:dbl)
                    n269 = local read "trial #"() -> (w683:dbl)
                    n270 = local read "ITI (s)"() -> (w681:dbl)
                    n271 = local read "time (s)"() -> (w692:dbl)
                    n272 = Increment(x=w690) -> (x+1=w689:dbl)
                    n273 = local read "mistake # 3.2R"() -> (w684:dbl)
                    n274 = local read "mistake # 3.1L"() -> (w685:dbl)
                    n275 = local write "lick # 3.2R"(w689) -> ()
                    n276 = local read "Mouse path 3"() -> (w694:path)
                    n277 = Build Array(w692, w691, w689, w688, w687, w686, w686, w683, w682, w681, w686, w685, w684) -> (w693:dbl[])
                    n278 = call-poly <vilib>:"Write To Spreadsheet File.vi"("append to file? (new file:F)"=TRUE, "1D data"=w693, "file path (dialog if empty)"=w694) -> ()  [unwired: 5 in, 1 out]
                  }
                }
              }
            }
          }
          frame 3 {
            n279 = case shown="True" w752 {
              frame False {
              }
              frame True {
                n280 = local read "state 3.1"() -> (w808:enum16{"waiting", "sound", "ITI"})
                n281 = case shown="\"sound\"" w808 {
                  frame "waiting", Default {
                    w815 = 0.0 ("element")
                    n282 = local read "water # 3.2R"() -> (w817:dbl)
                    n283 = local read "water # 3.1L"() -> (w819:dbl)
                    n284 = local read "lick # 3.1L"() -> (w822:dbl)
                    n285 = local write "state 3.2"(enum16{"waiting", "sound", "ITI"}."ITI") -> ()
                    n286 = local read "lick # 3.2R"() -> (w820:dbl)
                    n287 = local write "state 3.1"(enum16{"waiting", "sound", "ITI"}."ITI") -> ()
                    n288 = local read "time (s)"() -> (w816:dbl)
                    n289 = local read "current sound"() -> (w811:dbl)
                    n290 = Increment(x=w822) -> (x+1=w821:dbl)
                    n291 = Increment(x=w819) -> (x+1=w818:dbl)
                    n292 = local read "trial #"() -> (w812:dbl)
                    n293 = local read "mistake # 3.2R"() -> (w813:dbl)
                    n294 = local read "free water 3.1"() -> (w826:bool)
                    n295 = local write "water # 3.1L"(w818) -> ()
                    n296 = local write "lick # 3.1L"(w821) -> ()
                    n297 = local write "last water 3.1L"(w816) -> ()
                    n298 = local read "mistake # 3.1L"() -> (w814:dbl)
                    n299 = local read "ITI (s)"() -> (w810:dbl)
                    n300 = local read "Mouse path 3"() -> (w825:path)
                    n301 = case shown="False" w826 {
                      frame False {
                        n302 = local read "water dur (ms) 3.1"() -> (w829:dbl)
                        n303 = local read "water port 3.1"() -> (w830:tag)
                        n304 = call "_digital_on_duration_off.vi"("duration (ms)"=w829, "digital port"=w830) -> ()  [unwired: 10 in]
                      }
                      frame True {
                      }
                    }
                    n305 = Build Array(w816, w821, w820, w818, w817, 1.0 ("element"), w815, w812, w811, w810, w815, w814, w813) -> (w823:dbl[])
                    n306 = call-poly <vilib>:"Write To Spreadsheet File.vi"("append to file? (new file:F)"=TRUE, "1D data"=w823, "file path (dialog if empty)"=w825) -> ()  [unwired: 5 in, 1 out]
                  }
                  frame "sound" {
                    w836 = 0.0 ("element")
                    n307 = local read "lick # 3.2R"() -> (w839:dbl)
                    n308 = local read "water # 3.2R"() -> (w837:dbl)
                    n309 = local read "water # 3.1L"() -> (w838:dbl)
                    n310 = local read "current sound"() -> (w832:dbl)
                    n311 = local read "lick # 3.1L"() -> (w841:dbl)
                    n312 = local read "trial #"() -> (w833:dbl)
                    n313 = local read "ITI (s)"() -> (w831:dbl)
                    n314 = Increment(x=w841) -> (x+1=w840:dbl)
                    n315 = local read "mistake # 3.2R"() -> (w834:dbl)
                    n316 = local read "time (s)"() -> (w842:dbl)
                    n317 = local read "mistake # 3.1L"() -> (w835:dbl)
                    n318 = local write "lick # 3.1L"(w840) -> ()
                    n319 = local read "Mouse path 3"() -> (w844:path)
                    n320 = Build Array(w842, w840, w839, w838, w837, w836, w836, w833, w832, w831, w836, w835, w834) -> (w843:dbl[])
                    n321 = call-poly <vilib>:"Write To Spreadsheet File.vi"("append to file? (new file:F)"=TRUE, "1D data"=w843, "file path (dialog if empty)"=w844) -> ()  [unwired: 5 in, 1 out]
                  }
                  frame "ITI" {
                    w851 = 0.0 ("element")
                    n322 = local read "water # 3.2R"() -> (w852:dbl)
                    n323 = local read "water # 3.1L"() -> (w853:dbl)
                    n324 = local read "lick # 3.2R"() -> (w854:dbl)
                    n325 = local read "lick # 3.1L"() -> (w856:dbl)
                    n326 = local read "current sound"() -> (w847:dbl)
                    n327 = local read "trial #"() -> (w848:dbl)
                    n328 = local read "ITI (s)"() -> (w846:dbl)
                    n329 = local read "time (s)"() -> (w857:dbl)
                    n330 = local read "mistake # 3.2R"() -> (w849:dbl)
                    n331 = local read "mistake # 3.1L"() -> (w850:dbl)
                    n332 = Increment(x=w856) -> (x+1=w855:dbl)
                    n333 = local write "lick # 3.1L"(w855) -> ()
                    n334 = local read "Mouse path 3"() -> (w859:path)
                    n335 = Build Array(w857, w855, w854, w853, w852, w851, w851, w848, w847, w846, w851, w850, w849) -> (w858:dbl[])
                    n336 = call-poly <vilib>:"Write To Spreadsheet File.vi"("append to file? (new file:F)"=TRUE, "1D data"=w858, "file path (dialog if empty)"=w859) -> ()  [unwired: 5 in, 1 out]
                  }
                }
              }
            }
            n337 = case shown="True" w751 {
              frame False {
              }
              frame True {
                n338 = local read "state 3.1"() -> (w753:enum16{"waiting", "sound", "ITI"})
                n339 = case shown="\"sound\"" w753 {
                  frame "waiting", Default {
                    w762 = 0.0 ("element")
                    n340 = local write "state 3.2"(enum16{"waiting", "sound", "ITI"}."ITI") -> ()
                    n341 = local write "state 3.1"(enum16{"waiting", "sound", "ITI"}."ITI") -> ()
                    n342 = local read "current sound"() -> (w755:dbl)
                    n343 = local read "trial #"() -> (w756:dbl)
                    n344 = local read "ITI (s)"() -> (w754:dbl)
                    n345 = local read "lick # 3.2R"() -> (w766:dbl)
                    n346 = local read "water # 3.2R"() -> (w763:dbl)
                    n347 = local read "water # 3.1L"() -> (w764:dbl)
                    n348 = local read "mistake # 3.1L"() -> (w761:dbl)
                    n349 = local read "mistake # 3.2R"() -> (w759:dbl)
                    n350 = local read "lick # 3.1L"() -> (w767:dbl)
                    n351 = local read "time (s)"() -> (w768:dbl)
                    n352 = Increment(x=w766) -> (x+1=w765:dbl)
                    n353 = Increment(x=w761) -> (x+1=w760:dbl)
                    n354 = local write "lick # 3.2R"(w765) -> ()
                    n355 = local write "mistake # 3.1L"(w760) -> ()
                    n356 = local read "Mouse path 3"() -> (w769:path)
                    n357 = Build Array(w768, w767, w765, w764, w763, w762, w762, w756, w755, w754, w762, w760, w759) -> (w770:dbl[])
                    n358 = call-poly <vilib>:"Write To Spreadsheet File.vi"("append to file? (new file:F)"=TRUE, "1D data"=w770, "file path (dialog if empty)"=w769) -> ()  [unwired: 5 in, 1 out]
                    n359 = local read "LED 3"() -> (w758:tag)
                    n360 = local write "LED 3 (i)"(1.0 ("LED 3 (i)")) -> ()
                    n361 = call "_digital_on.vi"("digital port"=w758) -> ()  [unwired: 11 in]
                  }
                  frame "sound" {
                    w783 = 0.0 ("element")
                    n362 = local read "current sound"() -> (w779:dbl)
                    n363 = local read "water # 3.2R"() -> (w784:dbl)
                    n364 = local read "trial #"() -> (w780:dbl)
                    n365 = local read "ITI (s)"() -> (w778:dbl)
                    n366 = local read "water # 3.1L"() -> (w785:dbl)
                    n367 = local read "lick # 3.2R"() -> (w787:dbl)
                    n368 = local read "mistake # 3.2R"() -> (w781:dbl)
                    n369 = local read "lick # 3.1L"() -> (w788:dbl)
                    n370 = local read "mistake # 3.1L"() -> (w782:dbl)
                    n371 = local read "time (s)"() -> (w789:dbl)
                    n372 = Increment(x=w787) -> (x+1=w786:dbl)
                    n373 = local read "Mouse path 3"() -> (w791:path)
                    n374 = local write "lick # 3.2R"(w786) -> ()
                    n375 = Build Array(w789, w788, w786, w785, w784, w783, w783, w780, w779, w778, w783, w782, w781) -> (w790:dbl[])
                    n376 = local read "LED 3"() -> (w776:tag)
                    n377 = call-poly <vilib>:"Write To Spreadsheet File.vi"("append to file? (new file:F)"=TRUE, "1D data"=w790, "file path (dialog if empty)"=w791) -> ()  [unwired: 5 in, 1 out]
                    n378 = call "_digital_on.vi"("digital port"=w776) -> ()  [unwired: 11 in]
                    n379 = local write "state 3.1"(enum16{"waiting", "sound", "ITI"}."ITI") -> ()
                    n380 = local write "state 3.2"(enum16{"waiting", "sound", "ITI"}."ITI") -> ()
                    n381 = local write "LED 3 (i)"(1.0 ("LED 3 (i)")) -> ()
                  }
                  frame "ITI" {
                    w798 = 0.0 ("element")
                    n382 = local read "current sound"() -> (w794:dbl)
                    n383 = local read "lick # 3.2R"() -> (w802:dbl)
                    n384 = local read "water # 3.2R"() -> (w799:dbl)
                    n385 = local read "water # 3.1L"() -> (w800:dbl)
                    n386 = local read "lick # 3.1L"() -> (w803:dbl)
                    n387 = local read "trial #"() -> (w795:dbl)
                    n388 = local read "ITI (s)"() -> (w793:dbl)
                    n389 = local read "mistake # 3.1L"() -> (w797:dbl)
                    n390 = local read "mistake # 3.2R"() -> (w796:dbl)
                    n391 = Increment(x=w802) -> (x+1=w801:dbl)
                    n392 = local read "time (s)"() -> (w804:dbl)
                    n393 = local write "lick # 3.2R"(w801) -> ()
                    n394 = local read "Mouse path 3"() -> (w806:path)
                    n395 = Build Array(w804, w803, w801, w800, w799, w798, w798, w795, w794, w793, w798, w797, w796) -> (w805:dbl[])
                    n396 = call-poly <vilib>:"Write To Spreadsheet File.vi"("append to file? (new file:F)"=TRUE, "1D data"=w805, "file path (dialog if empty)"=w806) -> ()  [unwired: 5 in, 1 out]
                  }
                }
              }
            }
          }
          frame 4 {
            n397 = case shown="True" w862 {
              frame False {
              }
              frame True {
                n398 = local read "state 3.2"() -> (w916:enum16{"waiting", "sound", "ITI"})
                n399 = case shown="\"sound\"" w916 {
                  frame "waiting", Default {
                    w925 = 0.0 ("element")
                    n400 = local read "current sound"() -> (w918:dbl)
                    n401 = local read "mistake # 3.2R"() -> (w923:dbl)
                    n402 = local read "trial #"() -> (w919:dbl)
                    n403 = local read "mistake # 3.1L"() -> (w924:dbl)
                    n404 = local read "water # 3.2R"() -> (w926:dbl)
                    n405 = local read "water # 3.1L"() -> (w927:dbl)
                    n406 = local read "lick # 3.2R"() -> (w928:dbl)
                    n407 = local read "ITI (s)"() -> (w917:dbl)
                    n408 = local read "lick # 3.1L"() -> (w930:dbl)
                    n409 = local write "state 3.2"(enum16{"waiting", "sound", "ITI"}."ITI") -> ()
                    n410 = local read "LED 3"() -> (w920:tag)
                    n411 = local write "state 3.1"(enum16{"waiting", "sound", "ITI"}."ITI") -> ()
                    n412 = local write "LED 3 (i)"(1.0 ("LED 3 (i)")) -> ()
                    n413 = local read "time (s)"() -> (w931:dbl)
                    n414 = Increment(x=w923) -> (x+1=w922:dbl)
                    n415 = Increment(x=w930) -> (x+1=w929:dbl)
                    n416 = local write "mistake # 3.2R"(w922) -> ()
                    n417 = local write "lick # 3.1L"(w929) -> ()
                    n418 = local read "Mouse path 3"() -> (w933:path)
                    n419 = Build Array(w931, w929, w928, w927, w926, w925, w925, w919, w918, w917, w925, w924, w922) -> (w932:dbl[])
                    n420 = call "_digital_on.vi"("digital port"=w920) -> ()  [unwired: 11 in]
                    n421 = call-poly <vilib>:"Write To Spreadsheet File.vi"("append to file? (new file:F)"=TRUE, "1D data"=w932, "file path (dialog if empty)"=w933) -> ()  [unwired: 5 in, 1 out]
                  }
                  frame "sound" {
                    w946 = 0.0 ("element")
                    n422 = local read "current sound"() -> (w942:dbl)
                    n423 = local read "mistake # 3.2R"() -> (w944:dbl)
                    n424 = local read "water # 3.2R"() -> (w947:dbl)
                    n425 = local read "trial #"() -> (w943:dbl)
                    n426 = local read "mistake # 3.1L"() -> (w945:dbl)
                    n427 = local read "water # 3.1L"() -> (w948:dbl)
                    n428 = local read "ITI (s)"() -> (w941:dbl)
                    n429 = local read "lick # 3.2R"() -> (w949:dbl)
                    n430 = local read "lick # 3.1L"() -> (w951:dbl)
                    n431 = local read "time (s)"() -> (w952:dbl)
                    n432 = Increment(x=w951) -> (x+1=w950:dbl)
                    n433 = local read "Mouse path 3"() -> (w954:path)
                    n434 = local write "lick # 3.1L"(w950) -> ()
                    n435 = Build Array(w952, w950, w949, w948, w947, w946, w946, w943, w942, w941, w946, w945, w944) -> (w953:dbl[])
                    n436 = local read "LED 3"() -> (w939:tag)
                    n437 = local write "state 3.2"(enum16{"waiting", "sound", "ITI"}."ITI") -> ()
                    n438 = call-poly <vilib>:"Write To Spreadsheet File.vi"("append to file? (new file:F)"=TRUE, "1D data"=w953, "file path (dialog if empty)"=w954) -> ()  [unwired: 5 in, 1 out]
                    n439 = local write "state 3.1"(enum16{"waiting", "sound", "ITI"}."ITI") -> ()
                    n440 = call "_digital_on.vi"("digital port"=w939) -> ()  [unwired: 11 in]
                    n441 = local write "LED 3 (i)"(1.0 ("LED 4 (i)")) -> ()
                  }
                  frame "ITI" {
                    w961 = 0.0 ("element")
                    n442 = local read "water # 3.1L"() -> (w963:dbl)
                    n443 = local read "water # 3.2R"() -> (w962:dbl)
                    n444 = local read "current sound"() -> (w957:dbl)
                    n445 = local read "lick # 3.2R"() -> (w964:dbl)
                    n446 = local read "lick # 3.1L"() -> (w966:dbl)
                    n447 = local read "trial #"() -> (w958:dbl)
                    n448 = local read "ITI (s)"() -> (w956:dbl)
                    n449 = local read "mistake # 3.1L"() -> (w960:dbl)
                    n450 = local read "mistake # 3.2R"() -> (w959:dbl)
                    n451 = local read "time (s)"() -> (w967:dbl)
                    n452 = Increment(x=w966) -> (x+1=w965:dbl)
                    n453 = local write "lick # 3.1L"(w965) -> ()
                    n454 = Build Array(w967, w965, w964, w963, w962, w961, w961, w958, w957, w956, w961, w960, w959) -> (w968:dbl[])
                    n455 = local read "Mouse path 3"() -> (w969:path)
                    n456 = call-poly <vilib>:"Write To Spreadsheet File.vi"("append to file? (new file:F)"=TRUE, "1D data"=w968, "file path (dialog if empty)"=w969) -> ()  [unwired: 5 in, 1 out]
                  }
                }
              }
            }
            n457 = case shown="True" w861 {
              frame False {
              }
              frame True {
                n458 = local read "state 3.2"() -> (w863:enum16{"waiting", "sound", "ITI"})
                n459 = case shown="\"sound\"" w863 {
                  frame "waiting", Default {
                    w872 = 0.0 ("element")
                    n460 = local read "lick # 3.2R"() -> (w877:dbl)
                    n461 = local read "water # 3.2R"() -> (w874:dbl)
                    n462 = local read "water # 3.1L"() -> (w875:dbl)
                    n463 = local read "current sound"() -> (w865:dbl)
                    n464 = local read "lick # 3.1L"() -> (w878:dbl)
                    n465 = local read "trial #"() -> (w866:dbl)
                    n466 = local read "mistake # 3.1L"() -> (w871:dbl)
                    n467 = local read "mistake # 3.2R"() -> (w870:dbl)
                    n468 = local read "time (s)"() -> (w868:dbl)
                    n469 = local read "ITI (s)"() -> (w864:dbl)
                    n470 = Increment(x=w877) -> (x+1=w876:dbl)
                    n471 = Increment(x=w874) -> (x+1=w873:dbl)
                    n472 = local write "water # 3.2R"(w873) -> ()
                    n473 = local write "state 3.2"(enum16{"waiting", "sound", "ITI"}."ITI") -> ()
                    n474 = local write "state 3.1"(enum16{"waiting", "sound", "ITI"}."ITI") -> ()
                    n475 = local write "last water 3.2R"(w868) -> ()
                    n476 = local write "lick # 3.2R"(w876) -> ()
                    n477 = local read "Mouse path 3"() -> (w880:path)
                    n478 = local read "free water 3.2"() -> (w869:bool)
                    n479 = Build Array(w868, w878, w876, w875, w873, 1.0 ("element"), w872, w866, w865, w864, w872, w871, w870) -> (w879:dbl[])
                    n480 = call-poly <vilib>:"Write To Spreadsheet File.vi"("append to file? (new file:F)"=TRUE, "1D data"=w879, "file path (dialog if empty)"=w880) -> ()  [unwired: 5 in, 1 out]
                    n481 = case shown="False" w869 {
                      frame False {
                        n482 = local read "water dur (ms) 3. 2"() -> (w885:dbl)
                        n483 = local read "water port 3.2"() -> (w884:tag)
                        n484 = call "_digital_on_duration_off.vi"("duration (ms)"=w885, "digital port"=w884) -> ()  [unwired: 10 in]
                      }
                      frame True {
                      }
                    }
                  }
                  frame "sound" {
                    w891 = 0.0 ("element")
                    n485 = local read "water # 3.2R"() -> (w892:dbl)
                    n486 = local read "water # 3.1L"() -> (w893:dbl)
                    n487 = local read "lick # 3.2R"() -> (w895:dbl)
                    n488 = local read "current sound"() -> (w887:dbl)
                    n489 = local read "lick # 3.1L"() -> (w896:dbl)
                    n490 = local read "trial #"() -> (w888:dbl)
                    n491 = local read "ITI (s)"() -> (w886:dbl)
                    n492 = local read "mistake # 3.2R"() -> (w889:dbl)
                    n493 = local read "time (s)"() -> (w897:dbl)
                    n494 = local read "mistake # 3.1L"() -> (w890:dbl)
                    n495 = Increment(x=w895) -> (x+1=w894:dbl)
                    n496 = local write "lick # 3.2R"(w894) -> ()
                    n497 = local read "Mouse path 3"() -> (w899:path)
                    n498 = Build Array(w897, w896, w894, w893, w892, w891, w891, w888, w887, w886, w891, w890, w889) -> (w898:dbl[])
                    n499 = call-poly <vilib>:"Write To Spreadsheet File.vi"("append to file? (new file:F)"=TRUE, "1D data"=w898, "file path (dialog if empty)"=w899) -> ()  [unwired: 5 in, 1 out]
                  }
                  frame "ITI" {
                    w906 = 0.0 ("element")
                    n500 = local read "water # 3.2R"() -> (w907:dbl)
                    n501 = local read "lick # 3.2R"() -> (w910:dbl)
                    n502 = local read "water # 3.1L"() -> (w908:dbl)
                    n503 = local read "current sound"() -> (w902:dbl)
                    n504 = local read "trial #"() -> (w903:dbl)
                    n505 = local read "ITI (s)"() -> (w901:dbl)
                    n506 = local read "lick # 3.1L"() -> (w911:dbl)
                    n507 = local read "time (s)"() -> (w912:dbl)
                    n508 = local read "mistake # 3.2R"() -> (w904:dbl)
                    n509 = local read "mistake # 3.1L"() -> (w905:dbl)
                    n510 = Increment(x=w910) -> (x+1=w909:dbl)
                    n511 = local write "lick # 3.2R"(w909) -> ()
                    n512 = local read "Mouse path 3"() -> (w914:path)
                    n513 = Build Array(w912, w911, w909, w908, w907, w906, w906, w903, w902, w901, w906, w905, w904) -> (w913:dbl[])
                    n514 = call-poly <vilib>:"Write To Spreadsheet File.vi"("append to file? (new file:F)"=TRUE, "1D data"=w913, "file path (dialog if empty)"=w914) -> ()  [unwired: 5 in, 1 out]
                  }
                }
              }
            }
          }
        }
        n515 = case shown="1" w66 {
          tunnel: w62 -> [_ w972 w1082 w1192 w1302]
          tunnel: w63 -> [_ w971 w1081 w1191 w1301]
          frame 0, Default {
          }
          frame 1 {
            n516 = case shown="True" w972 {
              frame False {
              }
              frame True {
                n517 = local read "state 2.1"() -> (w1028:enum16{"waiting", "sound", "ITI"})
                n518 = case shown="\"waiting\", Default" w1028 {
                  frame "waiting", Default {
                    w1030 = 0.0 ("element")
                    n519 = local read "free water 2.1"() -> (w1034:bool)
                    n520 = case shown="False" w1034 {
                      frame False {
                        n521 = call "_digital_on_duration_off.vi"("duration (ms)"="water dur (ms) 2.1", "digital port"="water port 2.1") -> ()  [unwired: 10 in]
                      }
                      frame True {
                      }
                    }
                    n522 = local write "state 2.2"(enum16{"waiting", "sound", "ITI"}."ITI") -> ()
                    n523 = local write "state 2.1"(enum16{"waiting", "sound", "ITI"}."ITI") -> ()
                    n524 = local read "lick  #  2.1L"() -> (w1043:dbl)
                    n525 = local read "water # 2.2R"() -> (w1038:dbl)
                    n526 = local read "water # 2.1L"() -> (w1040:dbl)
                    n527 = local read "lick  #  2.2R"() -> (w1041:dbl)
                    n528 = local read "current sound"() -> (w1032:dbl)
                    n529 = Increment(x=w1043) -> (x+1=w1042:dbl)
                    n530 = local read "mistake # 2.2R"() -> (w1036:dbl)
                    n531 = local read "mistake # 2.1L"() -> (w1037:dbl)
                    n532 = Increment(x=w1040) -> (x+1=w1039:dbl)
                    n533 = local read "time (s)"() -> (w1035:dbl)
                    n534 = local read "trial #"() -> (w1033:dbl)
                    n535 = local read "ITI (s)"() -> (w1031:dbl)
                    n536 = local write "lick  #  2.1L"(w1042) -> ()
                    n537 = local write "water # 2.1L"(w1039) -> ()
                    n538 = local write "last water 2.1L"(w1035) -> ()
                    n539 = local read "Mouse path 2"() -> (w1046:path)
                    n540 = Build Array(w1035, w1042, w1041, w1039, w1038, 1.0 ("element"), w1030, w1033, w1032, w1031, w1030, w1037, w1036) -> (w1044:dbl[])
                    n541 = call-poly <vilib>:"Write To Spreadsheet File.vi"("append to file? (new file:F)"=TRUE, "1D data"=w1044, "file path (dialog if empty)"=w1046) -> ()  [unwired: 5 in, 1 out]
                  }
                  frame "sound" {
                    w1056 = 0.0 ("element")
                    n542 = local read "water # 2.2R"() -> (w1057:dbl)
                    n543 = local read "water # 2.1L"() -> (w1058:dbl)
                    n544 = local read "lick  #  2.2R"() -> (w1059:dbl)
                    n545 = local read "lick  #  2.1L"() -> (w1061:dbl)
                    n546 = local read "current sound"() -> (w1052:dbl)
                    n547 = local read "trial #"() -> (w1053:dbl)
                    n548 = local read "ITI (s)"() -> (w1051:dbl)
                    n549 = local read "mistake # 2.2R"() -> (w1054:dbl)
                    n550 = local read "mistake # 2.1L"() -> (w1055:dbl)
                    n551 = local read "time (s)"() -> (w1062:dbl)
                    n552 = Increment(x=w1061) -> (x+1=w1060:dbl)
                    n553 = local write "lick  #  2.1L"(w1060) -> ()
                    n554 = local read "Mouse path 2"() -> (w1065:path)
                    n555 = Build Array(w1062, w1060, w1059, w1058, w1057, w1056, w1056, w1053, w1052, w1051, w1056, w1055, w1054) -> (w1063:dbl[])
                    n556 = call-poly <vilib>:"Write To Spreadsheet File.vi"("append to file? (new file:F)"=TRUE, "1D data"=w1063, "file path (dialog if empty)"=w1065) -> ()  [unwired: 5 in, 1 out]
                  }
                  frame "ITI" {
                    w1071 = 0.0 ("element")
                    n557 = local read "water # 2.2R"() -> (w1072:dbl)
                    n558 = local read "water # 2.1L"() -> (w1073:dbl)
                    n559 = local read "lick  #  2.2R"() -> (w1074:dbl)
                    n560 = local read "current sound"() -> (w1067:dbl)
                    n561 = local read "lick  #  2.1L"() -> (w1076:dbl)
                    n562 = local read "trial #"() -> (w1068:dbl)
                    n563 = local read "time (s)"() -> (w1077:dbl)
                    n564 = local read "ITI (s)"() -> (w1066:dbl)
                    n565 = Increment(x=w1076) -> (x+1=w1075:dbl)
                    n566 = local read "mistake # 2.2R"() -> (w1069:dbl)
                    n567 = local read "mistake # 2.1L"() -> (w1070:dbl)
                    n568 = local write "lick  #  2.1L"(w1075) -> ()
                    n569 = local read "Mouse path 2"() -> (w1079:path)
                    n570 = Build Array(w1077, w1075, w1074, w1073, w1072, w1071, w1071, w1068, w1067, w1066, w1071, w1070, w1069) -> (w1078:dbl[])
                    n571 = call-poly <vilib>:"Write To Spreadsheet File.vi"("append to file? (new file:F)"=TRUE, "1D data"=w1078, "file path (dialog if empty)"=w1079) -> ()  [unwired: 5 in, 1 out]
                  }
                }
              }
            }
            n572 = case shown="True" w971 {
              frame False {
              }
              frame True {
                n573 = local read "state 2.1"() -> (w973:enum16{"waiting", "sound", "ITI"})
                n574 = case shown="\"sound\"" w973 {
                  frame "waiting", Default {
                    w982 = 0.0 ("element")
                    n575 = local write "LED 2 (i)"(1.0 ("LED 2 (i)")) -> ()
                    n576 = local read "water # 2.2R"() -> (w983:dbl)
                    n577 = local read "lick  #  2.2R"() -> (w987:dbl)
                    n578 = local read "water # 2.1L"() -> (w984:dbl)
                    n579 = local read "mistake # 2.1L"() -> (w981:dbl)
                    n580 = local read "lick  #  2.1L"() -> (w986:dbl)
                    n581 = local read "mistake # 2.2R"() -> (w979:dbl)
                    n582 = local read "current sound"() -> (w975:dbl)
                    n583 = local read "trial #"() -> (w976:dbl)
                    n584 = local write "state 2.2"(enum16{"waiting", "sound", "ITI"}."ITI") -> ()
                    n585 = local read "time (s)"() -> (w988:dbl)
                    n586 = Increment(x=w987) -> (x+1=w985:dbl)
                    n587 = local read "ITI (s)"() -> (w974:dbl)
                    n588 = Increment(x=w981) -> (x+1=w980:dbl)
                    n589 = local write "state 2.1"(enum16{"waiting", "sound", "ITI"}."ITI") -> ()
                    n590 = local write "lick  #  2.2R"(w985) -> ()
                    n591 = local write "mistake # 2.1L"(w980) -> ()
                    n592 = local read "Mouse path 2"() -> (w991:path)
                    n593 = Build Array(w988, w986, w985, w984, w983, w982, w982, w976, w975, w974, w982, w980, w979) -> (w990:dbl[])
                    n594 = call-poly <vilib>:"Write To Spreadsheet File.vi"("append to file? (new file:F)"=TRUE, "1D data"=w990, "file path (dialog if empty)"=w991) -> ()  [unwired: 5 in, 1 out]
                    n595 = call "_digital_on.vi"("digital port"="LED 2") -> ()  [unwired: 11 in]
                  }
                  frame "ITI" {
                    w999 = 0.0 ("element")
                    n596 = local read "water # 2.2R"() -> (w1000:dbl)
                    n597 = local read "lick  #  2.2R"() -> (w1003:dbl)
                    n598 = local read "water # 2.1L"() -> (w1001:dbl)
                    n599 = local read "current sound"() -> (w995:dbl)
                    n600 = local read "lick  #  2.1L"() -> (w1004:dbl)
                    n601 = Increment(x=w1003) -> (x+1=w1002:dbl)
                    n602 = local read "trial #"() -> (w996:dbl)
                    n603 = local read "time (s)"() -> (w1005:dbl)
                    n604 = local read "ITI (s)"() -> (w994:dbl)
                    n605 = local read "mistake # 2.2R"() -> (w997:dbl)
                    n606 = local write "lick  #  2.2R"(w1002) -> ()
                    n607 = local read "mistake # 2.1L"() -> (w998:dbl)
                    n608 = local read "Mouse path 2"() -> (w1007:path)
                    n609 = Build Array(w1005, w1004, w1002, w1001, w1000, w999, w999, w996, w995, w994, w999, w998, w997) -> (w1006:dbl[])
                    n610 = call-poly <vilib>:"Write To Spreadsheet File.vi"("append to file? (new file:F)"=TRUE, "1D data"=w1006, "file path (dialog if empty)"=w1007) -> ()  [unwired: 5 in, 1 out]
                  }
                  frame "sound" {
                    w1018 = 0.0 ("element")
                    n611 = local read "LED 2"() -> (w1011:tag)
                    n612 = local read "water # 2.2R"() -> (w1019:dbl)
                    n613 = local write "LED 2 (i)"(1.0 ("LED 2 (i)")) -> ()
                    n614 = local read "water # 2.1L"() -> (w1020:dbl)
                    n615 = local read "lick  #  2.2R"() -> (w1022:dbl)
                    n616 = local read "lick  #  2.1L"() -> (w1023:dbl)
                    n617 = local read "current sound"() -> (w1014:dbl)
                    n618 = call "_digital_on.vi"("digital port"=w1011) -> ()  [unwired: 11 in]
                    n619 = local read "trial #"() -> (w1015:dbl)
                    n620 = Increment(x=w1022) -> (x+1=w1021:dbl)
                    n621 = local read "ITI (s)"() -> (w1013:dbl)
                    n622 = local read "time (s)"() -> (w1024:dbl)
                    n623 = local write "lick  #  2.2R"(w1021) -> ()
                    n624 = local read "mistake # 2.2R"() -> (w1016:dbl)
                    n625 = local read "mistake # 2.1L"() -> (w1017:dbl)
                    n626 = local write "state 2.1"(enum16{"waiting", "sound", "ITI"}."ITI") -> ()
                    n627 = local write "state 2.2"(enum16{"waiting", "sound", "ITI"}."ITI") -> ()
                    n628 = local read "Mouse path 2"() -> (w1026:path)
                    n629 = Build Array(w1024, w1023, w1021, w1020, w1019, w1018, w1018, w1015, w1014, w1013, w1018, w1017, w1016) -> (w1025:dbl[])
                    n630 = call-poly <vilib>:"Write To Spreadsheet File.vi"("append to file? (new file:F)"=TRUE, "1D data"=w1025, "file path (dialog if empty)"=w1026) -> ()  [unwired: 5 in, 1 out]
                  }
                }
              }
            }
          }
          frame 2 {
            n631 = case shown="True" w1082 {
              frame False {
              }
              frame True {
                n632 = local read "state 2.2"() -> (w1136:enum16{"waiting", "sound", "ITI"})
                n633 = case shown="\"sound\"" w1136 {
                  frame "waiting", Default {
                    w1145 = 0.0 ("element")
                    n634 = local read "LED 2"() -> (w1140:tag)
                    n635 = local write "state 2.2"(enum16{"waiting", "sound", "ITI"}."ITI") -> ()
                    n636 = local write "state 2.1"(enum16{"waiting", "sound", "ITI"}."ITI") -> ()
                    n637 = local read "current sound"() -> (w1138:dbl)
                    n638 = local read "water # 2.2R"() -> (w1146:dbl)
                    n639 = local read "water # 2.1L"() -> (w1147:dbl)
                    n640 = local read "trial #"() -> (w1139:dbl)
                    n641 = local read "lick  #  2.2R"() -> (w1148:dbl)
                    n642 = local read "lick  #  2.1L"() -> (w1150:dbl)
                    n643 = local read "mistake # 2.2R"() -> (w1143:dbl)
                    n644 = call "_digital_on.vi"("digital port"=w1140) -> ()  [unwired: 11 in]
                    n645 = local read "ITI (s)"() -> (w1137:dbl)
                    n646 = local read "mistake # 2.1L"() -> (w1144:dbl)
                    n647 = local read "time (s)"() -> (w1151:dbl)
                    n648 = Increment(x=w1150) -> (x+1=w1149:dbl)
                    n649 = Increment(x=w1143) -> (x+1=w1142:dbl)
                    n650 = local write "lick  #  2.1L"(w1149) -> ()
                    n651 = local read "Mouse path 2"() -> (w1153:path)
                    n652 = local write "mistake # 2.2R"(w1142) -> ()
                    n653 = Build Array(w1151, w1149, w1148, w1147, w1146, w1145, w1145, w1139, w1138, w1137, w1145, w1144, w1142) -> (w1152:dbl[])
                    n654 = local write "LED 2 (i)"(1.0 ("LED 2 (i)")) -> ()
                    n655 = call-poly <vilib>:"Write To Spreadsheet File.vi"("append to file? (new file:F)"=TRUE, "1D data"=w1152, "file path (dialog if empty)"=w1153) -> ()  [unwired: 5 in, 1 out]
                  }
                  frame "sound" {
                    w1166 = 0.0 ("element")
                    n656 = local read "water # 2.2R"() -> (w1167:dbl)
                    n657 = local read "current sound"() -> (w1162:dbl)
                    n658 = local read "water # 2.1L"() -> (w1168:dbl)
                    n659 = local read "lick  #  2.2R"() -> (w1169:dbl)
                    n660 = local read "lick  #  2.1L"() -> (w1171:dbl)
                    n661 = local read "trial #"() -> (w1163:dbl)
                    n662 = local read "ITI (s)"() -> (w1161:dbl)
                    n663 = local read "mistake # 2.2R"() -> (w1164:dbl)
                    n664 = local read "mistake # 2.1L"() -> (w1165:dbl)
                    n665 = Increment(x=w1171) -> (x+1=w1170:dbl)
                    n666 = local read "time (s)"() -> (w1172:dbl)
                    n667 = local write "lick  #  2.1L"(w1170) -> ()
                    n668 = local read "Mouse path 2"() -> (w1174:path)
                    n669 = Build Array(w1172, w1170, w1169, w1168, w1167, w1166, w1166, w1163, w1162, w1161, w1166, w1165, w1164) -> (w1173:dbl[])
                    n670 = call-poly <vilib>:"Write To Spreadsheet File.vi"("append to file? (new file:F)"=TRUE, "1D data"=w1173, "file path (dialog if empty)"=w1174) -> ()  [unwired: 5 in, 1 out]
                    n671 = local write "state 2.2"(enum16{"waiting", "sound", "ITI"}."ITI") -> ()
                    n672 = local read "LED 2"() -> (w1159:tag)
                    n673 = local write "state 2.1"(enum16{"waiting", "sound", "ITI"}."ITI") -> ()
                    n674 = local write "LED 2 (i)"(1.0 ("LED 2 (i)")) -> ()
                    n675 = call "_digital_on.vi"("digital port"=w1159) -> ()  [unwired: 11 in]
                  }
                  frame "ITI" {
                    w1181 = 0.0 ("element")
                    n676 = local read "water # 2.2R"() -> (w1182:dbl)
                    n677 = local read "water # 2.1L"() -> (w1183:dbl)
                    n678 = local read "lick  #  2.1L"() -> (w1186:dbl)
                    n679 = local read "lick  #  2.2R"() -> (w1184:dbl)
                    n680 = local read "current sound"() -> (w1177:dbl)
                    n681 = local read "time (s)"() -> (w1187:dbl)
                    n682 = local read "trial #"() -> (w1178:dbl)
                    n683 = Increment(x=w1186) -> (x+1=w1185:dbl)
                    n684 = local read "ITI (s)"() -> (w1176:dbl)
                    n685 = local read "mistake # 2.2R"() -> (w1179:dbl)
                    n686 = local read "mistake # 2.1L"() -> (w1180:dbl)
                    n687 = local write "lick  #  2.1L"(w1185) -> ()
                    n688 = local read "Mouse path 2"() -> (w1189:path)
                    n689 = Build Array(w1187, w1185, w1184, w1183, w1182, w1181, w1181, w1178, w1177, w1176, w1181, w1180, w1179) -> (w1188:dbl[])
                    n690 = call-poly <vilib>:"Write To Spreadsheet File.vi"("append to file? (new file:F)"=TRUE, "1D data"=w1188, "file path (dialog if empty)"=w1189) -> ()  [unwired: 5 in, 1 out]
                  }
                }
              }
            }
            n691 = case shown="True" w1081 {
              frame False {
              }
              frame True {
                n692 = local read "state 2.2"() -> (w1083:enum16{"waiting", "sound", "ITI"})
                n693 = case shown="\"waiting\", Default" w1083 {
                  frame "waiting", Default {
                    w1094 = 0.0 ("element")
                    n694 = local read "water # 2.2R"() -> (w1089:dbl)
                    n695 = local read "water # 2.1L"() -> (w1095:dbl)
                    n696 = local read "lick  #  2.2R"() -> (w1097:dbl)
                    n697 = local read "lick  #  2.1L"() -> (w1098:dbl)
                    n698 = local read "current sound"() -> (w1086:dbl)
                    n699 = local read "time (s)"() -> (w1091:dbl)
                    n700 = Increment(x=w1089) -> (x+1=w1088:dbl)
                    n701 = Increment(x=w1097) -> (x+1=w1096:dbl)
                    n702 = local read "trial #"() -> (w1087:dbl)
                    n703 = local read "ITI (s)"() -> (w1085:dbl)
                    n704 = local read "mistake # 2.2R"() -> (w1092:dbl)
                    n705 = local write "water # 2.2R"(w1088) -> ()
                    n706 = local read "mistake # 2.1L"() -> (w1093:dbl)
                    n707 = local read "free water 2.2"() -> (w1090:bool)
                    n708 = local write "lick  #  2.2R"(w1096) -> ()
                    n709 = local write "last water 2.2R"(w1091) -> ()
                    n710 = local read "Mouse path 2"() -> (w1100:path)
                    n711 = Build Array(w1091, w1098, w1096, w1095, w1088, 1.0 ("element"), w1094, w1087, w1086, w1085, w1094, w1093, w1092) -> (w1099:dbl[])
                    n712 = case shown="False" w1090 {
                      frame False {
                        n713 = call "_digital_on_duration_off.vi"("duration (ms)"="water dur (ms) 2.2", "digital port"="water port 2.2") -> ()  [unwired: 10 in]
                      }
                      frame True {
                      }
                    }
                    n714 = local write "state 2.2"(enum16{"waiting", "sound", "ITI"}."ITI") -> ()
                    n715 = call-poly <vilib>:"Write To Spreadsheet File.vi"("append to file? (new file:F)"=TRUE, "1D data"=w1099, "file path (dialog if empty)"=w1100) -> ()  [unwired: 5 in, 1 out]
                    n716 = local write "state 2.1"(enum16{"waiting", "sound", "ITI"}."ITI") -> ()
                  }
                  frame "ITI" {
                    w1111 = 0.0 ("element")
                    n717 = local read "water # 2.2R"() -> (w1112:dbl)
                    n718 = local read "water # 2.1L"() -> (w1113:dbl)
                    n719 = local read "current sound"() -> (w1107:dbl)
                    n720 = local read "lick  #  2.2R"() -> (w1115:dbl)
                    n721 = local read "lick  #  2.1L"() -> (w1116:dbl)
                    n722 = local read "trial #"() -> (w1108:dbl)
                    n723 = local read "ITI (s)"() -> (w1106:dbl)
                    n724 = Increment(x=w1115) -> (x+1=w1114:dbl)
                    n725 = local read "mistake # 2.2R"() -> (w1109:dbl)
                    n726 = local read "mistake # 2.1L"() -> (w1110:dbl)
                    n727 = local write "lick  #  2.2R"(w1114) -> ()
                    n728 = local read "time (s)"() -> (w1117:dbl)
                    n729 = local read "Mouse path 2"() -> (w1120:path)
                    n730 = Build Array(w1117, w1116, w1114, w1113, w1112, w1111, w1111, w1108, w1107, w1106, w1111, w1110, w1109) -> (w1118:dbl[])
                    n731 = call-poly <vilib>:"Write To Spreadsheet File.vi"("append to file? (new file:F)"=TRUE, "1D data"=w1118, "file path (dialog if empty)"=w1120) -> ()  [unwired: 5 in, 1 out]
                  }
                  frame "sound" {
                    w1126 = 0.0 ("element")
                    n732 = local read "water # 2.2R"() -> (w1127:dbl)
                    n733 = local read "water # 2.1L"() -> (w1128:dbl)
                    n734 = local read "current sound"() -> (w1122:dbl)
                    n735 = local read "trial #"() -> (w1123:dbl)
                    n736 = local read "lick  #  2.2R"() -> (w1130:dbl)
                    n737 = local read "lick  #  2.1L"() -> (w1131:dbl)
                    n738 = local read "ITI (s)"() -> (w1121:dbl)
                    n739 = local read "mistake # 2.2R"() -> (w1124:dbl)
                    n740 = local read "time (s)"() -> (w1132:dbl)
                    n741 = Increment(x=w1130) -> (x+1=w1129:dbl)
                    n742 = local read "mistake # 2.1L"() -> (w1125:dbl)
                    n743 = local write "lick  #  2.2R"(w1129) -> ()
                    n744 = local read "Mouse path 2"() -> (w1135:path)
                    n745 = Build Array(w1132, w1131, w1129, w1128, w1127, w1126, w1126, w1123, w1122, w1121, w1126, w1125, w1124) -> (w1133:dbl[])
                    n746 = call-poly <vilib>:"Write To Spreadsheet File.vi"("append to file? (new file:F)"=TRUE, "1D data"=w1133, "file path (dialog if empty)"=w1135) -> ()  [unwired: 5 in, 1 out]
                  }
                }
              }
            }
          }
          frame 3 {
            n747 = case shown="True" w1192 {
              frame False {
              }
              frame True {
                n748 = local read "state 2.1"() -> (w1248:enum16{"waiting", "sound", "ITI"})
                n749 = case shown="\"sound\"" w1248 {
                  frame "waiting", Default {
                    w1257 = 0.0 ("element")
                    n750 = local read "water # 2.1L"() -> (w1260:dbl)
                    n751 = local read "lick  #  2.2R"() -> (w1261:dbl)
                    n752 = local read "lick  #  2.1L"() -> (w1263:dbl)
                    n753 = local read "water # 2.2R"() -> (w1258:dbl)
                    n754 = local write "state 2.2"(enum16{"waiting", "sound", "ITI"}."ITI") -> ()
                    n755 = local write "state 2.1"(enum16{"waiting", "sound", "ITI"}."ITI") -> ()
                    n756 = local read "mistake # 2.2R"() -> (w1255:dbl)
                    n757 = local read "mistake # 2.1L"() -> (w1256:dbl)
                    n758 = Increment(x=w1260) -> (x+1=w1259:dbl)
                    n759 = Increment(x=w1263) -> (x+1=w1262:dbl)
                    n760 = local read "time (s)"() -> (w1254:dbl)
                    n761 = local read "current sound"() -> (w1250:dbl)
                    n762 = local read "free water 2.1"() -> (w1253:bool)
                    n763 = local write "water # 2.1L"(w1259) -> ()
                    n764 = local read "ITI (s)"() -> (w1249:dbl)
                    n765 = local read "trial #"() -> (w1251:dbl)
                    n766 = local write "lick  #  2.1L"(w1262) -> ()
                    n767 = local write "last water 2.1L"(w1254) -> ()
                    n768 = case shown="False" w1253 {
                      frame False {
                        n769 = local read "water dur (ms) 2.1"() -> (w1270:dbl)
                        n770 = local read "water port 2.1"() -> (w1269:tag)
                        n771 = call "_digital_on_duration_off.vi"("duration (ms)"=w1270, "digital port"=w1269) -> ()  [unwired: 10 in]
                      }
                      frame True {
                      }
                    }
                    n772 = Build Array(w1254, w1262, w1261, w1259, w1258, 1.0 ("element"), w1257, w1251, w1250, w1249, w1257, w1256, w1255) -> (w1264:dbl[])
                    n773 = local read "Mouse path 2"() -> (w1265:path)
                    n774 = call-poly <vilib>:"Write To Spreadsheet File.vi"("append to file? (new file:F)"=TRUE, "1D data"=w1264, "file path (dialog if empty)"=w1265) -> ()  [unwired: 5 in, 1 out]
                  }
                  frame "ITI" {
                    w1276 = 0.0 ("element")
                    n775 = local read "lick  #  2.2R"() -> (w1279:dbl)
                    n776 = local read "water # 2.2R"() -> (w1277:dbl)
                    n777 = local read "water # 2.1L"() -> (w1278:dbl)
                    n778 = local read "lick  #  2.1L"() -> (w1281:dbl)
                    n779 = local read "current sound"() -> (w1272:dbl)
                    n780 = local read "mistake # 2.2R"() -> (w1274:dbl)
                    n781 = local read "trial #"() -> (w1273:dbl)
                    n782 = local read "ITI (s)"() -> (w1271:dbl)
                    n783 = local read "mistake # 2.1L"() -> (w1275:dbl)
                    n784 = local read "time (s)"() -> (w1282:dbl)
                    n785 = Increment(x=w1281) -> (x+1=w1280:dbl)
                    n786 = local write "lick  #  2.1L"(w1280) -> ()
                    n787 = local read "Mouse path 2"() -> (w1284:path)
                    n788 = Build Array(w1282, w1280, w1279, w1278, w1277, w1276, w1276, w1273, w1272, w1271, w1276, w1275, w1274) -> (w1283:dbl[])
                    n789 = call-poly <vilib>:"Write To Spreadsheet File.vi"("append to file? (new file:F)"=TRUE, "1D data"=w1283, "file path (dialog if empty)"=w1284) -> ()  [unwired: 5 in, 1 out]
                  }
                  frame "sound" {
                    w1291 = 0.0 ("element")
                    n790 = local read "current sound"() -> (w1287:dbl)
                    n791 = local read "water # 2.2R"() -> (w1292:dbl)
                    n792 = local read "water # 2.1L"() -> (w1293:dbl)
                    n793 = local read "lick  #  2.1L"() -> (w1296:dbl)
                    n794 = local read "trial #"() -> (w1288:dbl)
                    n795 = local read "ITI (s)"() -> (w1286:dbl)
                    n796 = local read "mistake # 2.2R"() -> (w1289:dbl)
                    n797 = local read "lick  #  2.2R"() -> (w1294:dbl)
                    n798 = local read "mistake # 2.1L"() -> (w1290:dbl)
                    n799 = local read "time (s)"() -> (w1297:dbl)
                    n800 = Increment(x=w1296) -> (x+1=w1295:dbl)
                    n801 = local read "Mouse path 2"() -> (w1299:path)
                    n802 = local write "lick  #  2.1L"(w1295) -> ()
                    n803 = Build Array(w1297, w1295, w1294, w1293, w1292, w1291, w1291, w1288, w1287, w1286, w1291, w1290, w1289) -> (w1298:dbl[])
                    n804 = call-poly <vilib>:"Write To Spreadsheet File.vi"("append to file? (new file:F)"=TRUE, "1D data"=w1298, "file path (dialog if empty)"=w1299) -> ()  [unwired: 5 in, 1 out]
                  }
                }
              }
            }
            n805 = case shown="True" w1191 {
              frame False {
              }
              frame True {
                n806 = local read "state 2.1"() -> (w1193:enum16{"waiting", "sound", "ITI"})
                n807 = case shown="\"sound\"" w1193 {
                  frame "waiting", Default {
                    w1202 = 0.0 ("element")
                    n808 = local read "LED 2"() -> (w1198:tag)
                    n809 = local write "LED 2 (i)"(1.0 ("LED 2 (i)")) -> ()
                    n810 = local write "state 2.2"(enum16{"waiting", "sound", "ITI"}."ITI") -> ()
                    n811 = local write "state 2.1"(enum16{"waiting", "sound", "ITI"}."ITI") -> ()
                    n812 = local read "water # 2.2R"() -> (w1203:dbl)
                    n813 = local read "mistake # 2.2R"() -> (w1199:dbl)
                    n814 = local read "current sound"() -> (w1195:dbl)
                    n815 = local read "water # 2.1L"() -> (w1204:dbl)
                    n816 = local read "lick  #  2.2R"() -> (w1206:dbl)
                    n817 = local read "mistake # 2.1L"() -> (w1201:dbl)
                    n818 = call "_digital_on.vi"("digital port"=w1198) -> ()  [unwired: 11 in]
                    n819 = local read "trial #"() -> (w1196:dbl)
                    n820 = local read "ITI (s)"() -> (w1194:dbl)
                    n821 = local read "lick  #  2.1L"() -> (w1207:dbl)
                    n822 = local read "time (s)"() -> (w1208:dbl)
                    n823 = Increment(x=w1206) -> (x+1=w1205:dbl)
                    n824 = Increment(x=w1201) -> (x+1=w1200:dbl)
                    n825 = local write "mistake # 2.1L"(w1200) -> ()
                    n826 = local write "lick  #  2.2R"(w1205) -> ()
                    n827 = local read "Mouse path 2"() -> (w1211:path)
                    n828 = Build Array(w1208, w1207, w1205, w1204, w1203, w1202, w1202, w1196, w1195, w1194, w1202, w1200, w1199) -> (w1209:dbl[])
                    n829 = call-poly <vilib>:"Write To Spreadsheet File.vi"("append to file? (new file:F)"=TRUE, "1D data"=w1209, "file path (dialog if empty)"=w1211) -> ()  [unwired: 5 in, 1 out]
                  }
                  frame "ITI" {
                    w1219 = 0.0 ("element")
                    n830 = local read "water # 2.2R"() -> (w1220:dbl)
                    n831 = local read "water # 2.1L"() -> (w1221:dbl)
                    n832 = local read "lick  #  2.2R"() -> (w1223:dbl)
                    n833 = local read "current sound"() -> (w1215:dbl)
                    n834 = local read "mistake # 2.2R"() -> (w1217:dbl)
                    n835 = local read "mistake # 2.1L"() -> (w1218:dbl)
                    n836 = local read "lick  #  2.1L"() -> (w1224:dbl)
                    n837 = local read "trial #"() -> (w1216:dbl)
                    n838 = local read "ITI (s)"() -> (w1214:dbl)
                    n839 = local read "time (s)"() -> (w1225:dbl)
                    n840 = Increment(x=w1223) -> (x+1=w1222:dbl)
                    n841 = local write "lick  #  2.2R"(w1222) -> ()
                    n842 = local read "Mouse path 2"() -> (w1227:path)
                    n843 = Build Array(w1225, w1224, w1222, w1221, w1220, w1219, w1219, w1216, w1215, w1214, w1219, w1218, w1217) -> (w1226:dbl[])
                    n844 = call-poly <vilib>:"Write To Spreadsheet File.vi"("append to file? (new file:F)"=TRUE, "1D data"=w1226, "file path (dialog if empty)"=w1227) -> ()  [unwired: 5 in, 1 out]
                  }
                  frame "sound" {
                    w1238 = 0.0 ("element")
                    n845 = local read "LED 2"() -> (w1231:tag)
                    n846 = local read "water # 2.2R"() -> (w1239:dbl)
                    n847 = local read "current sound"() -> (w1234:dbl)
                    n848 = local write "LED 2 (i)"(1.0 ("LED 2 (i)")) -> ()
                    n849 = local read "water # 2.1L"() -> (w1240:dbl)
                    n850 = local read "lick  #  2.2R"() -> (w1242:dbl)
                    n851 = local read "trial #"() -> (w1235:dbl)
                    n852 = local read "ITI (s)"() -> (w1233:dbl)
                    n853 = local read "lick  #  2.1L"() -> (w1243:dbl)
                    n854 = local read "mistake # 2.2R"() -> (w1236:dbl)
                    n855 = call "_digital_on.vi"("digital port"=w1231) -> ()  [unwired: 11 in]
                    n856 = local read "mistake # 2.1L"() -> (w1237:dbl)
                    n857 = Increment(x=w1242) -> (x+1=w1241:dbl)
                    n858 = local read "time (s)"() -> (w1244:dbl)
                    n859 = local write "lick  #  2.2R"(w1241) -> ()
                    n860 = local write "state 2.1"(enum16{"waiting", "sound", "ITI"}."ITI") -> ()
                    n861 = local write "state 2.2"(enum16{"waiting", "sound", "ITI"}."ITI") -> ()
                    n862 = local read "Mouse path 2"() -> (w1246:path)
                    n863 = Build Array(w1244, w1243, w1241, w1240, w1239, w1238, w1238, w1235, w1234, w1233, w1238, w1237, w1236) -> (w1245:dbl[])
                    n864 = call-poly <vilib>:"Write To Spreadsheet File.vi"("append to file? (new file:F)"=TRUE, "1D data"=w1245, "file path (dialog if empty)"=w1246) -> ()  [unwired: 5 in, 1 out]
                  }
                }
              }
            }
          }
          frame 4 {
            n865 = case shown="True" w1302 {
              frame False {
              }
              frame True {
                n866 = local read "state 2.2"() -> (w1356:enum16{"waiting", "sound", "ITI"})
                n867 = case shown="\"sound\"" w1356 {
                  frame "waiting", Default {
                    w1365 = 0.0 ("element")
                    n868 = local read "LED 2"() -> (w1361:tag)
                    n869 = local write "LED 2 (i)"(1.0 ("LED 2 (i)")) -> ()
                    n870 = local read "lick  #  2.2R"() -> (w1368:dbl)
                    n871 = call "_digital_on.vi"("digital port"=w1361) -> ()  [unwired: 11 in]
                    n872 = local read "lick  #  2.1L"() -> (w1370:dbl)
                    n873 = local read "current sound"() -> (w1358:dbl)
                    n874 = local read "water # 2.2R"() -> (w1366:dbl)
                    n875 = local read "water # 2.1L"() -> (w1367:dbl)
                    n876 = local read "trial #"() -> (w1359:dbl)
                    n877 = local read "mistake # 2.2R"() -> (w1363:dbl)
                    n878 = local read "mistake # 2.1L"() -> (w1364:dbl)
                    n879 = local read "ITI (s)"() -> (w1357:dbl)
                    n880 = local read "time (s)"() -> (w1371:dbl)
                    n881 = Increment(x=w1370) -> (x+1=w1369:dbl)
                    n882 = local write "lick  #  2.1L"(w1369) -> ()
                    n883 = local read "Mouse path 2"() -> (w1373:path)
                    n884 = Increment(x=w1363) -> (x+1=w1362:dbl)
                    n885 = local write "mistake # 2.2R"(w1362) -> ()
                    n886 = Build Array(w1371, w1369, w1368, w1367, w1366, w1365, w1365, w1359, w1358, w1357, w1365, w1364, w1362) -> (w1372:dbl[])
                    n887 = call-poly <vilib>:"Write To Spreadsheet File.vi"("append to file? (new file:F)"=TRUE, "1D data"=w1372, "file path (dialog if empty)"=w1373) -> ()  [unwired: 5 in, 1 out]
                    n888 = local write "state 2.2"(enum16{"waiting", "sound", "ITI"}."ITI") -> ()
                    n889 = local write "state 2.1"(enum16{"waiting", "sound", "ITI"}."ITI") -> ()
                  }
                  frame "sound" {
                    w1386 = 0.0 ("element")
                    n890 = local read "current sound"() -> (w1382:dbl)
                    n891 = local read "lick  #  2.2R"() -> (w1389:dbl)
                    n892 = local read "lick  #  2.1L"() -> (w1391:dbl)
                    n893 = local read "water # 2.2R"() -> (w1387:dbl)
                    n894 = local read "trial #"() -> (w1383:dbl)
                    n895 = local write "state 2.1"(enum16{"waiting", "sound", "ITI"}."ITI") -> ()
                    n896 = local read "ITI (s)"() -> (w1381:dbl)
                    n897 = local read "water # 2.1L"() -> (w1388:dbl)
                    n898 = local write "state 2.2"(enum16{"waiting", "sound", "ITI"}."ITI") -> ()
                    n899 = local read "mistake # 2.2R"() -> (w1384:dbl)
                    n900 = local read "time (s)"() -> (w1392:dbl)
                    n901 = local read "mistake # 2.1L"() -> (w1385:dbl)
                    n902 = Increment(x=w1391) -> (x+1=w1390:dbl)
                    n903 = local write "lick  #  2.1L"(w1390) -> ()
                    n904 = local read "Mouse path 2"() -> (w1394:path)
                    n905 = Build Array(w1392, w1390, w1389, w1388, w1387, w1386, w1386, w1383, w1382, w1381, w1386, w1385, w1384) -> (w1393:dbl[])
                    n906 = local read "LED 2"() -> (w1380:tag)
                    n907 = call-poly <vilib>:"Write To Spreadsheet File.vi"("append to file? (new file:F)"=TRUE, "1D data"=w1393, "file path (dialog if empty)"=w1394) -> ()  [unwired: 5 in, 1 out]
                    n908 = local write "LED 2 (i)"(1.0 ("LED 2 (i)")) -> ()
                    n909 = call "_digital_on.vi"("digital port"=w1380) -> ()  [unwired: 11 in]
                  }
                  frame "ITI" {
                    w1401 = 0.0 ("element")
                    n910 = local read "water # 2.1L"() -> (w1403:dbl)
                    n911 = local read "water # 2.2R"() -> (w1402:dbl)
                    n912 = local read "current sound"() -> (w1397:dbl)
                    n913 = local read "lick  #  2.2R"() -> (w1404:dbl)
                    n914 = local read "lick  #  2.1L"() -> (w1406:dbl)
                    n915 = local read "trial #"() -> (w1398:dbl)
                    n916 = local read "ITI (s)"() -> (w1396:dbl)
                    n917 = local read "mistake # 2.2R"() -> (w1399:dbl)
                    n918 = local read "mistake # 2.1L"() -> (w1400:dbl)
                    n919 = local read "time (s)"() -> (w1407:dbl)
                    n920 = Increment(x=w1406) -> (x+1=w1405:dbl)
                    n921 = local write "lick  #  2.1L"(w1405) -> ()
                    n922 = local read "Mouse path 2"() -> (w1409:path)
                    n923 = Build Array(w1407, w1405, w1404, w1403, w1402, w1401, w1401, w1398, w1397, w1396, w1401, w1400, w1399) -> (w1408:dbl[])
                    n924 = call-poly <vilib>:"Write To Spreadsheet File.vi"("append to file? (new file:F)"=TRUE, "1D data"=w1408, "file path (dialog if empty)"=w1409) -> ()  [unwired: 5 in, 1 out]
                  }
                }
              }
            }
            n925 = case shown="True" w1301 {
              frame False {
              }
              frame True {
                n926 = local read "state 2.2"() -> (w1303:enum16{"waiting", "sound", "ITI"})
                n927 = case shown="\"ITI\"" w1303 {
                  frame "waiting", Default {
                    w1311 = 0.0 ("element")
                    n928 = local read "water # 2.2R"() -> (w1313:dbl)
                    n929 = local read "lick  #  2.2R"() -> (w1316:dbl)
                    n930 = local read "water # 2.1L"() -> (w1314:dbl)
                    n931 = local read "lick  #  2.1L"() -> (w1317:dbl)
                    n932 = local read "current sound"() -> (w1305:dbl)
                    n933 = local read "trial #"() -> (w1306:dbl)
                    n934 = local read "time (s)"() -> (w1318:dbl)
                    n935 = local read "ITI (s)"() -> (w1304:dbl)
                    n936 = local read "mistake # 2.2R"() -> (w1309:dbl)
                    n937 = local read "mistake # 2.1L"() -> (w1310:dbl)
                    n938 = Increment(x=w1316) -> (x+1=w1315:dbl)
                    n939 = Increment(x=w1313) -> (x+1=w1312:dbl)
                    n940 = local write "state 2.1"(enum16{"waiting", "sound", "ITI"}."ITI") -> ()
                    n941 = local write "state 2.2"(enum16{"waiting", "sound", "ITI"}."ITI") -> ()
                    n942 = local write "water # 2.2R"(w1312) -> ()
                    n943 = local write "lick  #  2.2R"(w1315) -> ()
                    n944 = local read "Mouse path 2"() -> (w1320:path)
                    n945 = Build Array(w1318, w1317, w1315, w1314, w1312, 1.0 ("element"), w1311, w1306, w1305, w1304, w1311, w1310, w1309) -> (w1319:dbl[])
                    n946 = call-poly <vilib>:"Write To Spreadsheet File.vi"("append to file? (new file:F)"=TRUE, "1D data"=w1319, "file path (dialog if empty)"=w1320) -> ()  [unwired: 5 in, 1 out]
                    n947 = local read "free water 2.2"() -> (w1308:bool)
                    n948 = case shown="False" w1308 {
                      frame False {
                        n949 = local read "water dur (ms) 2.2"() -> (w1325:dbl)
                        n950 = local read "water port 2.2"() -> (w1324:tag)
                        n951 = call "_digital_on_duration_off.vi"("duration (ms)"=w1325, "digital port"=w1324) -> ()  [unwired: 10 in]
                      }
                      frame True {
                      }
                    }
                  }
                  frame "sound" {
                    w1331 = 0.0 ("element")
                    n952 = local read "current sound"() -> (w1327:dbl)
                    n953 = local read "water # 2.1L"() -> (w1333:dbl)
                    n954 = local read "water # 2.2R"() -> (w1332:dbl)
                    n955 = local read "lick  #  2.2R"() -> (w1335:dbl)
                    n956 = local read "lick  #  2.1L"() -> (w1336:dbl)
                    n957 = local read "trial #"() -> (w1328:dbl)
                    n958 = local read "ITI (s)"() -> (w1326:dbl)
                    n959 = local read "mistake # 2.2R"() -> (w1329:dbl)
                    n960 = local read "time (s)"() -> (w1337:dbl)
                    n961 = local read "mistake # 2.1L"() -> (w1330:dbl)
                    n962 = Increment(x=w1335) -> (x+1=w1334:dbl)
                    n963 = local write "lick  #  2.2R"(w1334) -> ()
                    n964 = local read "Mouse path 2"() -> (w1340:path)
                    n965 = Build Array(w1337, w1336, w1334, w1333, w1332, w1331, w1331, w1328, w1327, w1326, w1331, w1330, w1329) -> (w1338:dbl[])
                    n966 = call-poly <vilib>:"Write To Spreadsheet File.vi"("append to file? (new file:F)"=TRUE, "1D data"=w1338, "file path (dialog if empty)"=w1340) -> ()  [unwired: 5 in, 1 out]
                  }
                  frame "ITI" {
                    w1346 = 0.0 ("element")
                    n967 = local read "water # 2.2R"() -> (w1347:dbl)
                    n968 = local read "water # 2.1L"() -> (w1348:dbl)
                    n969 = local read "current sound"() -> (w1342:dbl)
                    n970 = local read "lick  #  2.2R"() -> (w1350:dbl)
                    n971 = local read "trial #"() -> (w1343:dbl)
                    n972 = local read "lick  #  2.1L"() -> (w1351:dbl)
                    n973 = local read "ITI (s)"() -> (w1341:dbl)
                    n974 = local read "time (s)"() -> (w1352:dbl)
                    n975 = Increment(x=w1350) -> (x+1=w1349:dbl)
                    n976 = local write "lick  #  2.2R"(w1349) -> ()
                    n977 = local read "mistake # 2.2R"() -> (w1344:dbl)
                    n978 = local read "mistake # 2.1L"() -> (w1345:dbl)
                    n979 = local read "Mouse path 2"() -> (w1353:path)
                    n980 = Build Array(w1352, w1351, w1349, w1348, w1347, w1346, w1346, w1343, w1342, w1341, w1346, w1345, w1344) -> (w1354:dbl[])
                    n981 = call-poly <vilib>:"Write To Spreadsheet File.vi"("append to file? (new file:F)"=TRUE, "1D data"=w1354, "file path (dialog if empty)"=w1353) -> ()  [unwired: 5 in, 1 out]
                  }
                }
              }
            }
          }
        }
        n982 = case shown="4" w44 {
          tunnel: w33 -> [_ w90 w201 w311 w421]
          tunnel: w34 -> [_ w91 w200 w310 w420]
          frame 0, Default {
          }
          frame 1 {
            n983 = case shown="True" w91 {
              frame False {
              }
              frame True {
                n984 = local read "state 4.1"() -> (w145:enum16{"waiting", "sound", "ITI"})
                n985 = case shown="\"sound\"" w145 {
                  frame "waiting", Default {
                    w154 = 0.0 ("element")
                    n986 = local read "water # 4.1L"() -> (w156:dbl)
                    n987 = local read "water # 4.2R"() -> (w155:dbl)
                    n988 = local read "lick # 4.2R"() -> (w158:dbl)
                    n989 = local read "lick # 4.1L"() -> (w159:dbl)
                    n990 = local read "current sound"() -> (w147:dbl)
                    n991 = local write "state 4.2"(enum16{"waiting", "sound", "ITI"}."ITI") -> ()
                    n992 = local read "trial #"() -> (w148:dbl)
                    n993 = local read "mistake # 4.2R"() -> (w151:dbl)
                    n994 = local write "state 4.1"(enum16{"waiting", "sound", "ITI"}."ITI") -> ()
                    n995 = local read "mistake # 4.1L"() -> (w153:dbl)
                    n996 = local read "ITI (s)"() -> (w146:dbl)
                    n997 = Increment(x=w158) -> (x+1=w157:dbl)
                    n998 = local read "time (s)"() -> (w160:dbl)
                    n999 = local write "lick # 4.2R"(w157) -> ()
                    n1000 = Increment(x=w153) -> (x+1=w152:dbl)
                    n1001 = local read "Mouse path 4"() -> (w162:path)
                    n1002 = local write "mistake # 4.1L"(w152) -> ()
                    n1003 = Build Array(w160, w159, w157, w156, w155, w154, w154, w148, w147, w146, w154, w152, w151) -> (w161:dbl[])
                    n1004 = call-poly <vilib>:"Write To Spreadsheet File.vi"("append to file? (new file:F)"=TRUE, "1D data"=w161, "file path (dialog if empty)"=w162) -> ()  [unwired: 5 in, 1 out]
                    n1005 = local read "LED 4"() -> (w149:tag)
                    n1006 = local write "LED 4 (i)"(1.0 ("LED 4 (i)")) -> ()
                    n1007 = call "_digital_on.vi"("digital port"=w149) -> ()  [unwired: 11 in]
                  }
                  frame "sound" {
                    w175 = 0.0 ("element")
                    n1008 = local read "LED 4"() -> (w168:tag)
                    n1009 = local read "water # 4.2R"() -> (w176:dbl)
                    n1010 = local read "lick # 4.2R"() -> (w179:dbl)
                    n1011 = local read "water # 4.1L"() -> (w177:dbl)
                    n1012 = local read "lick # 4.1L"() -> (w180:dbl)
                    n1013 = local write "LED 4 (i)"(1.0 ("LED 4 (i)")) -> ()
                    n1014 = local write "state 4.2"(enum16{"waiting", "sound", "ITI"}."ITI") -> ()
                    n1015 = local write "state 4.1"(enum16{"waiting", "sound", "ITI"}."ITI") -> ()
                    n1016 = local read "current sound"() -> (w171:dbl)
                    n1017 = call "_digital_on.vi"("digital port"=w168) -> ()  [unwired: 11 in]
                    n1018 = local read "time (s)"() -> (w181:dbl)
                    n1019 = Increment(x=w179) -> (x+1=w178:dbl)
                    n1020 = local read "trial #"() -> (w172:dbl)
                    n1021 = local read "ITI (s)"() -> (w170:dbl)
                    n1022 = local write "lick # 4.2R"(w178) -> ()
                    n1023 = local read "mistake # 4.2R"() -> (w173:dbl)
                    n1024 = local read "Mouse path 4"() -> (w183:path)
                    n1025 = local read "mistake # 4.1L"() -> (w174:dbl)
                    n1026 = Build Array(w181, w180, w178, w177, w176, w175, w175, w172, w171, w170, w175, w174, w173) -> (w182:dbl[])
                    n1027 = call-poly <vilib>:"Write To Spreadsheet File.vi"("append to file? (new file:F)"=TRUE, "1D data"=w182, "file path (dialog if empty)"=w183) -> ()  [unwired: 5 in, 1 out]
                  }
                  frame "ITI" {
                    w190 = 0.0 ("element")
                    n1028 = local read "current sound"() -> (w186:dbl)
                    n1029 = local read "water # 4.2R"() -> (w191:dbl)
                    n1030 = local read "water # 4.1L"() -> (w192:dbl)
                    n1031 = local read "trial #"() -> (w187:dbl)
                    n1032 = local read "lick # 4.2R"() -> (w194:dbl)
                    n1033 = local read "ITI (s)"() -> (w185:dbl)
                    n1034 = local read "lick # 4.1L"() -> (w195:dbl)
                    n1035 = local read "mistake # 4.2R"() -> (w188:dbl)
                    n1036 = local read "time (s)"() -> (w196:dbl)
                    n1037 = Increment(x=w194) -> (x+1=w193:dbl)
                    n1038 = local read "mistake # 4.1L"() -> (w189:dbl)
                    n1039 = local write "lick # 4.2R"(w193) -> ()
                    n1040 = local read "Mouse path 4"() -> (w198:path)
                    n1041 = Build Array(w196, w195, w193, w192, w191, w190, w190, w187, w186, w185, w190, w189, w188) -> (w197:dbl[])
                    n1042 = call-poly <vilib>:"Write To Spreadsheet File.vi"("append to file? (new file:F)"=TRUE, "1D data"=w197, "file path (dialog if empty)"=w198) -> ()  [unwired: 5 in, 1 out]
                  }
                }
              }
            }
            n1043 = case shown="True" w90 {
              frame False {
              }
              frame True {
                n1044 = local read "state 4.1"() -> (w92:enum16{"waiting", "sound", "ITI"})
                n1045 = case shown="\"sound\"" w92 {
                  frame "waiting", Default {
                    w100 = 0.0 ("element")
                    n1046 = local read "water # 4.1L"() -> (w103:dbl)
                    n1047 = local read "lick # 4.2R"() -> (w104:dbl)
                    n1048 = local read "lick # 4.1L"() -> (w106:dbl)
                    n1049 = local read "water # 4.2R"() -> (w101:dbl)
                    n1050 = local read "current sound"() -> (w94:dbl)
                    n1051 = local read "time (s)"() -> (w97:dbl)
                    n1052 = local read "trial #"() -> (w95:dbl)
                    n1053 = Increment(x=w103) -> (x+1=w102:dbl)
                    n1054 = Increment(x=w106) -> (x+1=w105:dbl)
                    n1055 = local write "state 4.2"(enum16{"waiting", "sound", "ITI"}."ITI") -> ()
                    n1056 = local write "state 4.1"(enum16{"waiting", "sound", "ITI"}."ITI") -> ()
                    n1057 = local read "ITI (s)"() -> (w93:dbl)
                    n1058 = local write "water # 4.1L"(w102) -> ()
                    n1059 = local read "mistake # 4.2R"() -> (w98:dbl)
                    n1060 = local read "mistake # 4.1L"() -> (w99:dbl)
                    n1061 = local write "last water 4.1L"(w97) -> ()
                    n1062 = local write "lick # 4.1L"(w105) -> ()
                    n1063 = local read "Mouse path 4"() -> (w108:path)
                    n1064 = Build Array(w97, w105, w104, w102, w101, 1.0 ("element"), w100, w95, w94, w93, w100, w99, w98) -> (w107:dbl[])
                    n1065 = local read "free water 4.1"() -> (w110:bool)
                    n1066 = call-poly <vilib>:"Write To Spreadsheet File.vi"("append to file? (new file:F)"=TRUE, "1D data"=w107, "file path (dialog if empty)"=w108) -> ()  [unwired: 5 in, 1 out]
                    n1067 = case shown="False" w110 {
                      frame False {
                        n1068 = call "_digital_on_duration_off.vi"("duration (ms)"="water dur (ms) 4.1", "digital port"="water port 4.1") -> ()  [unwired: 10 in]
                      }
                      frame True {
                      }
                    }
                  }
                  frame "sound" {
                    w120 = 0.0 ("element")
                    n1069 = local read "current sound"() -> (w116:dbl)
                    n1070 = local read "water # 4.2R"() -> (w121:dbl)
                    n1071 = local read "water # 4.1L"() -> (w122:dbl)
                    n1072 = local read "trial #"() -> (w117:dbl)
                    n1073 = local read "lick # 4.2R"() -> (w123:dbl)
                    n1074 = local read "ITI (s)"() -> (w115:dbl)
                    n1075 = local read "lick # 4.1L"() -> (w125:dbl)
                    n1076 = local read "mistake # 4.2R"() -> (w118:dbl)
                    n1077 = local read "time (s)"() -> (w126:dbl)
                    n1078 = local read "mistake # 4.1L"() -> (w119:dbl)
                    n1079 = Increment(x=w125) -> (x+1=w124:dbl)
                    n1080 = local write "lick # 4.1L"(w124) -> ()
                    n1081 = local read "Mouse path 4"() -> (w128:path)
                    n1082 = Build Array(w126, w124, w123, w122, w121, w120, w120, w117, w116, w115, w120, w119, w118) -> (w127:dbl[])
                    n1083 = call-poly <vilib>:"Write To Spreadsheet File.vi"("append to file? (new file:F)"=TRUE, "1D data"=w127, "file path (dialog if empty)"=w128) -> ()  [unwired: 5 in, 1 out]
                  }
                  frame "ITI" {
                    w135 = 0.0 ("element")
                    n1084 = local read "current sound"() -> (w131:dbl)
                    n1085 = local read "water # 4.2R"() -> (w136:dbl)
                    n1086 = local read "water # 4.1L"() -> (w137:dbl)
                    n1087 = local read "trial #"() -> (w132:dbl)
                    n1088 = local read "mistake # 4.2R"() -> (w133:dbl)
                    n1089 = local read "lick # 4.2R"() -> (w138:dbl)
                    n1090 = local read "mistake # 4.1L"() -> (w134:dbl)
                    n1091 = local read "lick # 4.1L"() -> (w140:dbl)
                    n1092 = local read "ITI (s)"() -> (w130:dbl)
                    n1093 = local read "time (s)"() -> (w141:dbl)
                    n1094 = Increment(x=w140) -> (x+1=w139:dbl)
                    n1095 = local write "lick # 4.1L"(w139) -> ()
                    n1096 = local read "Mouse path 4"() -> (w143:path)
                    n1097 = Build Array(w141, w139, w138, w137, w136, w135, w135, w132, w131, w130, w135, w134, w133) -> (w142:dbl[])
                    n1098 = call-poly <vilib>:"Write To Spreadsheet File.vi"("append to file? (new file:F)"=TRUE, "1D data"=w142, "file path (dialog if empty)"=w143) -> ()  [unwired: 5 in, 1 out]
                  }
                }
              }
            }
          }
          frame 2 {
            n1099 = case shown="True" w200 {
              frame False {
              }
              frame True {
                n1100 = local read "state 4.2"() -> (w257:enum16{"waiting", "sound", "ITI"})
                n1101 = case shown="\"sound\"" w257 {
                  frame "waiting", Default {
                    w265 = 0.0 ("element")
                    n1102 = local read "water # 4.2R"() -> (w267:dbl)
                    n1103 = local read "current sound"() -> (w259:dbl)
                    n1104 = local read "mistake # 4.2R"() -> (w263:dbl)
                    n1105 = local read "mistake # 4.1L"() -> (w264:dbl)
                    n1106 = local read "trial #"() -> (w260:dbl)
                    n1107 = local read "ITI (s)"() -> (w258:dbl)
                    n1108 = local read "water # 4.1L"() -> (w268:dbl)
                    n1109 = local read "lick # 4.2R"() -> (w270:dbl)
                    n1110 = local write "state 4.2"(enum16{"waiting", "sound", "ITI"}."ITI") -> ()
                    n1111 = local write "state 4.1"(enum16{"waiting", "sound", "ITI"}."ITI") -> ()
                    n1112 = local read "lick # 4.1L"() -> (w271:dbl)
                    n1113 = Increment(x=w267) -> (x+1=w266:dbl)
                    n1114 = local read "time (s)"() -> (w262:dbl)
                    n1115 = local write "water # 4.2R"(w266) -> ()
                    n1116 = Increment(x=w270) -> (x+1=w269:dbl)
                    n1117 = local write "last water 4.2R"(w262) -> ()
                    n1118 = local read "free water 4.2"() -> (w275:bool)
                    n1119 = local write "lick # 4.2R"(w269) -> ()
                    n1120 = Build Array(w262, w271, w269, w268, w266, 1.0 ("element"), w265, w260, w259, w258, w265, w264, w263) -> (w272:dbl[])
                    n1121 = local read "Mouse path 4"() -> (w273:path)
                    n1122 = case shown="False" w275 {
                      frame False {
                        n1123 = call "_digital_on_duration_off.vi"("duration (ms)"="water dur (ms) 4.2", "digital port"="water port 4.2") -> ()  [unwired: 10 in]
                      }
                      frame True {
                      }
                    }
                    n1124 = call-poly <vilib>:"Write To Spreadsheet File.vi"("append to file? (new file:F)"=TRUE, "1D data"=w272, "file path (dialog if empty)"=w273) -> ()  [unwired: 5 in, 1 out]
                  }
                  frame "sound" {
                    w285 = 0.0 ("element")
                    n1125 = local read "current sound"() -> (w281:dbl)
                    n1126 = local read "trial #"() -> (w282:dbl)
                    n1127 = local read "water # 4.1L"() -> (w287:dbl)
                    n1128 = local read "water # 4.2R"() -> (w286:dbl)
                    n1129 = local read "lick # 4.2R"() -> (w289:dbl)
                    n1130 = local read "ITI (s)"() -> (w280:dbl)
                    n1131 = local read "lick # 4.1L"() -> (w290:dbl)
                    n1132 = local read "time (s)"() -> (w291:dbl)
                    n1133 = Increment(x=w289) -> (x+1=w288:dbl)
                    n1134 = local read "mistake # 4.1L"() -> (w284:dbl)
                    n1135 = local read "mistake # 4.2R"() -> (w283:dbl)
                    n1136 = local write "lick # 4.2R"(w288) -> ()
                    n1137 = Build Array(w291, w290, w288, w287, w286, w285, w285, w282, w281, w280, w285, w284, w283) -> (w292:dbl[])
                    n1138 = local read "Mouse path 4"() -> (w293:path)
                    n1139 = call-poly <vilib>:"Write To Spreadsheet File.vi"("append to file? (new file:F)"=TRUE, "1D data"=w292, "file path (dialog if empty)"=w293) -> ()  [unwired: 5 in, 1 out]
                  }
                  frame "ITI" {
                    w300 = 0.0 ("element")
                    n1140 = local read "water # 4.2R"() -> (w301:dbl)
                    n1141 = local read "water # 4.1L"() -> (w302:dbl)
                    n1142 = local read "current sound"() -> (w296:dbl)
                    n1143 = local read "lick # 4.2R"() -> (w304:dbl)
                    n1144 = local read "trial #"() -> (w297:dbl)
                    n1145 = local read "lick # 4.1L"() -> (w305:dbl)
                    n1146 = local read "ITI (s)"() -> (w295:dbl)
                    n1147 = local read "mistake # 4.2R"() -> (w298:dbl)
                    n1148 = Increment(x=w304) -> (x+1=w303:dbl)
                    n1149 = local read "mistake # 4.1L"() -> (w299:dbl)
                    n1150 = local read "time (s)"() -> (w306:dbl)
                    n1151 = local write "lick # 4.2R"(w303) -> ()
                    n1152 = Build Array(w306, w305, w303, w302, w301, w300, w300, w297, w296, w295, w300, w299, w298) -> (w307:dbl[])
                    n1153 = local read "Mouse path 4"() -> (w308:path)
                    n1154 = call-poly <vilib>:"Write To Spreadsheet File.vi"("append to file? (new file:F)"=TRUE, "1D data"=w307, "file path (dialog if empty)"=w308) -> ()  [unwired: 5 in, 1 out]
                  }
                }
              }
            }
            n1155 = case shown="True" w201 {
              frame False {
              }
              frame True {
                n1156 = local read "state 4.2"() -> (w202:enum16{"waiting", "sound", "ITI"})
                n1157 = case shown="\"sound\"" w202 {
                  frame "waiting", Default {
                    w211 = 0.0 ("element")
                    n1158 = local read "lick # 4.2R"() -> (w214:dbl)
                    n1159 = local read "current sound"() -> (w204:dbl)
                    n1160 = local read "ITI (s)"() -> (w203:dbl)
                    n1161 = local read "lick # 4.1L"() -> (w216:dbl)
                    n1162 = local read "trial #"() -> (w205:dbl)
                    n1163 = local read "mistake # 4.2R"() -> (w209:dbl)
                    n1164 = local read "water # 4.1L"() -> (w213:dbl)
                    n1165 = local read "water # 4.2R"() -> (w212:dbl)
                    n1166 = local read "time (s)"() -> (w217:dbl)
                    n1167 = local write "state 4.2"(enum16{"waiting", "sound", "ITI"}."ITI") -> ()
                    n1168 = local write "state 4.1"(enum16{"waiting", "sound", "ITI"}."ITI") -> ()
                    n1169 = local read "mistake # 4.1L"() -> (w210:dbl)
                    n1170 = Increment(x=w216) -> (x+1=w215:dbl)
                    n1171 = Increment(x=w209) -> (x+1=w208:dbl)
                    n1172 = local write "lick # 4.1L"(w215) -> ()
                    n1173 = local write "mistake # 4.2R"(w208) -> ()
                    n1174 = Build Array(w217, w215, w214, w213, w212, w211, w211, w205, w204, w203, w211, w210, w208) -> (w218:dbl[])
                    n1175 = local read "Mouse path 4"() -> (w219:path)
                    n1176 = local write "LED 4 (i)"(1.0 ("LED 4 (i)")) -> ()
                    n1177 = call-poly <vilib>:"Write To Spreadsheet File.vi"("append to file? (new file:F)"=TRUE, "1D data"=w218, "file path (dialog if empty)"=w219) -> ()  [unwired: 5 in, 1 out]
                    n1178 = call "_digital_on.vi"("digital port"="LED 4") -> ()  [unwired: 11 in]
                  }
                  frame "sound" {
                    w232 = 0.0 ("element")
                    n1179 = local read "current sound"() -> (w228:dbl)
                    n1180 = local read "water # 4.2R"() -> (w233:dbl)
                    n1181 = local read "water # 4.1L"() -> (w234:dbl)
                    n1182 = local read "lick # 4.2R"() -> (w235:dbl)
                    n1183 = local read "trial #"() -> (w229:dbl)
                    n1184 = local read "lick # 4.1L"() -> (w237:dbl)
                    n1185 = local read "ITI (s)"() -> (w227:dbl)
                    n1186 = local read "mistake # 4.2R"() -> (w230:dbl)
                    n1187 = local read "time (s)"() -> (w238:dbl)
                    n1188 = local read "mistake # 4.1L"() -> (w231:dbl)
                    n1189 = Increment(x=w237) -> (x+1=w236:dbl)
                    n1190 = local write "lick # 4.1L"(w236) -> ()
                    n1191 = Build Array(w238, w236, w235, w234, w233, w232, w232, w229, w228, w227, w232, w231, w230) -> (w239:dbl[])
                    n1192 = local read "Mouse path 4"() -> (w240:path)
                    n1193 = local read "LED 4"() -> (w225:tag)
                    n1194 = local write "state 4.2"(enum16{"waiting", "sound", "ITI"}."ITI") -> ()
                    n1195 = local write "state 4.1"(enum16{"waiting", "sound", "ITI"}."ITI") -> ()
                    n1196 = call-poly <vilib>:"Write To Spreadsheet File.vi"("append to file? (new file:F)"=TRUE, "1D data"=w239, "file path (dialog if empty)"=w240) -> ()  [unwired: 5 in, 1 out]
                    n1197 = local write "LED 4 (i)"(1.0 ("LED 4 (i)")) -> ()
                    n1198 = call "_digital_on.vi"("digital port"=w225) -> ()  [unwired: 11 in]
                  }
                  frame "ITI" {
                    w247 = 0.0 ("element")
                    n1199 = local read "current sound"() -> (w243:dbl)
                    n1200 = local read "water # 4.1L"() -> (w249:dbl)
                    n1201 = local read "water # 4.2R"() -> (w248:dbl)
                    n1202 = local read "lick # 4.2R"() -> (w250:dbl)
                    n1203 = local read "trial #"() -> (w244:dbl)
                    n1204 = local read "ITI (s)"() -> (w242:dbl)
                    n1205 = local read "lick # 4.1L"() -> (w252:dbl)
                    n1206 = local read "time (s)"() -> (w253:dbl)
                    n1207 = local read "mistake # 4.2R"() -> (w245:dbl)
                    n1208 = Increment(x=w252) -> (x+1=w251:dbl)
                    n1209 = local read "mistake # 4.1L"() -> (w246:dbl)
                    n1210 = local write "lick # 4.1L"(w251) -> ()
                    n1211 = local read "Mouse path 4"() -> (w255:path)
                    n1212 = Build Array(w253, w251, w250, w249, w248, w247, w247, w244, w243, w242, w247, w246, w245) -> (w254:dbl[])
                    n1213 = call-poly <vilib>:"Write To Spreadsheet File.vi"("append to file? (new file:F)"=TRUE, "1D data"=w254, "file path (dialog if empty)"=w255) -> ()  [unwired: 5 in, 1 out]
                  }
                }
              }
            }
          }
          frame 3 {
            n1214 = case shown="True" w310 {
              frame False {
              }
              frame True {
                n1215 = local read "state 4.1"() -> (w365:enum16{"waiting", "sound", "ITI"})
                n1216 = case shown="\"sound\"" w365 {
                  frame "waiting", Default {
                    w374 = 0.0 ("element")
                    n1217 = local write "state 4.2"(enum16{"waiting", "sound", "ITI"}."ITI") -> ()
                    n1218 = local write "state 4.1"(enum16{"waiting", "sound", "ITI"}."ITI") -> ()
                    n1219 = local read "mistake # 4.1L"() -> (w373:dbl)
                    n1220 = local read "water # 4.2R"() -> (w375:dbl)
                    n1221 = local read "current sound"() -> (w367:dbl)
                    n1222 = local read "water # 4.1L"() -> (w376:dbl)
                    n1223 = local read "mistake # 4.2R"() -> (w371:dbl)
                    n1224 = local read "lick # 4.2R"() -> (w378:dbl)
                    n1225 = local read "trial #"() -> (w368:dbl)
                    n1226 = local read "ITI (s)"() -> (w366:dbl)
                    n1227 = local read "lick # 4.1L"() -> (w379:dbl)
                    n1228 = local read "time (s)"() -> (w380:dbl)
                    n1229 = Increment(x=w373) -> (x+1=w372:dbl)
                    n1230 = Increment(x=w378) -> (x+1=w377:dbl)
                    n1231 = local write "mistake # 4.1L"(w372) -> ()
                    n1232 = local write "lick # 4.2R"(w377) -> ()
                    n1233 = local read "Mouse path 4"() -> (w382:path)
                    n1234 = local read "LED 4"() -> (w369:tag)
                    n1235 = local write "LED 4 (i)"(1.0 ("LED 4 (i)")) -> ()
                    n1236 = Build Array(w380, w379, w377, w376, w375, w374, w374, w368, w367, w366, w374, w372, w371) -> (w381:dbl[])
                    n1237 = call "_digital_on.vi"("digital port"=w369) -> ()  [unwired: 11 in]
                    n1238 = call-poly <vilib>:"Write To Spreadsheet File.vi"("append to file? (new file:F)"=TRUE, "1D data"=w381, "file path (dialog if empty)"=w382) -> ()  [unwired: 5 in, 1 out]
                  }
                  frame "sound" {
                    w395 = 0.0 ("element")
                    n1239 = local read "lick # 4.2R"() -> (w399:dbl)
                    n1240 = local read "water # 4.1L"() -> (w397:dbl)
                    n1241 = local read "water # 4.2R"() -> (w396:dbl)
                    n1242 = local read "lick # 4.1L"() -> (w400:dbl)
                    n1243 = local read "current sound"() -> (w391:dbl)
                    n1244 = local read "time (s)"() -> (w401:dbl)
                    n1245 = local read "ITI (s)"() -> (w390:dbl)
                    n1246 = local read "trial #"() -> (w392:dbl)
                    n1247 = Increment(x=w399) -> (x+1=w398:dbl)
                    n1248 = local read "mistake # 4.2R"() -> (w393:dbl)
                    n1249 = local read "mistake # 4.1L"() -> (w394:dbl)
                    n1250 = local write "lick # 4.2R"(w398) -> ()
                    n1251 = Build Array(w401, w400, w398, w397, w396, w395, w395, w392, w391, w390, w395, w394, w393) -> (w402:dbl[])
                    n1252 = local read "Mouse path 4"() -> (w403:path)
                    n1253 = local write "state 4.1"(enum16{"waiting", "sound", "ITI"}."ITI") -> ()
                    n1254 = local read "LED 4"() -> (w388:tag)
                    n1255 = local write "state 4.2"(enum16{"waiting", "sound", "ITI"}."ITI") -> ()
                    n1256 = call-poly <vilib>:"Write To Spreadsheet File.vi"("append to file? (new file:F)"=TRUE, "1D data"=w402, "file path (dialog if empty)"=w403) -> ()  [unwired: 5 in, 1 out]
                    n1257 = local write "LED 4 (i)"(1.0 ("LED 4 (i)")) -> ()
                    n1258 = call "_digital_on.vi"("digital port"=w388) -> ()  [unwired: 11 in]
                  }
                  frame "ITI" {
                    w410 = 0.0 ("element")
                    n1259 = local read "water # 4.2R"() -> (w411:dbl)
                    n1260 = local read "water # 4.1L"() -> (w412:dbl)
                    n1261 = local read "current sound"() -> (w406:dbl)
                    n1262 = local read "lick # 4.2R"() -> (w414:dbl)
                    n1263 = local read "lick # 4.1L"() -> (w415:dbl)
                    n1264 = local read "trial #"() -> (w407:dbl)
                    n1265 = local read "time (s)"() -> (w416:dbl)
                    n1266 = local read "ITI (s)"() -> (w405:dbl)
                    n1267 = Increment(x=w414) -> (x+1=w413:dbl)
                    n1268 = local read "mistake # 4.1L"() -> (w409:dbl)
                    n1269 = local read "mistake # 4.2R"() -> (w408:dbl)
                    n1270 = local write "lick # 4.2R"(w413) -> ()
                    n1271 = local read "Mouse path 4"() -> (w418:path)
                    n1272 = Build Array(w416, w415, w413, w412, w411, w410, w410, w407, w406, w405, w410, w409, w408) -> (w417:dbl[])
                    n1273 = call-poly <vilib>:"Write To Spreadsheet File.vi"("append to file? (new file:F)"=TRUE, "1D data"=w417, "file path (dialog if empty)"=w418) -> ()  [unwired: 5 in, 1 out]
                  }
                }
              }
            }
            n1274 = case shown="True" w311 {
              frame False {
              }
              frame True {
                n1275 = local read "state 4.1"() -> (w312:enum16{"waiting", "sound", "ITI"})
                n1276 = case shown="\"sound\"" w312 {
                  frame "waiting", Default {
                    w320 = 0.0 ("element")
                    n1277 = local read "water # 4.1L"() -> (w323:dbl)
                    n1278 = local write "state 4.2"(enum16{"waiting", "sound", "ITI"}."ITI") -> ()
                    n1279 = local read "water # 4.2R"() -> (w321:dbl)
                    n1280 = local write "state 4.1"(enum16{"waiting", "sound", "ITI"}."ITI") -> ()
                    n1281 = local read "lick # 4.2R"() -> (w324:dbl)
                    n1282 = local read "lick # 4.1L"() -> (w326:dbl)
                    n1283 = local read "time (s)"() -> (w317:dbl)
                    n1284 = local read "mistake # 4.2R"() -> (w318:dbl)
                    n1285 = local read "current sound"() -> (w314:dbl)
                    n1286 = Increment(x=w323) -> (x+1=w322:dbl)
                    n1287 = local read "mistake # 4.1L"() -> (w319:dbl)
                    n1288 = local read "trial #"() -> (w315:dbl)
                    n1289 = Increment(x=w326) -> (x+1=w325:dbl)
                    n1290 = local read "ITI (s)"() -> (w313:dbl)
                    n1291 = local write "water # 4.1L"(w322) -> ()
                    n1292 = local write "last water 4.1L"(w317) -> ()
                    n1293 = local read "free water 4.1"() -> (w332:bool)
                    n1294 = local write "lick # 4.1L"(w325) -> ()
                    n1295 = local read "Mouse path 4"() -> (w328:path)
                    n1296 = Build Array(w317, w325, w324, w322, w321, 1.0 ("element"), w320, w315, w314, w313, w320, w319, w318) -> (w327:dbl[])
                    n1297 = case shown="False" w332 {
                      frame False {
                        n1298 = local read "water dur (ms) 4.1"() -> (w333:dbl)
                        n1299 = local read "water port 4.1"() -> (w334:tag)
                        n1300 = call "_digital_on_duration_off.vi"("duration (ms)"=w333, "digital port"=w334) -> ()  [unwired: 10 in]
                      }
                      frame True {
                      }
                    }
                    n1301 = call-poly <vilib>:"Write To Spreadsheet File.vi"("append to file? (new file:F)"=TRUE, "1D data"=w327, "file path (dialog if empty)"=w328) -> ()  [unwired: 5 in, 1 out]
                  }
                  frame "sound" {
                    w340 = 0.0 ("element")
                    n1302 = local read "water # 4.1L"() -> (w342:dbl)
                    n1303 = local read "water # 4.2R"() -> (w341:dbl)
                    n1304 = local read "lick # 4.2R"() -> (w343:dbl)
                    n1305 = local read "lick # 4.1L"() -> (w345:dbl)
                    n1306 = local read "current sound"() -> (w336:dbl)
                    n1307 = Increment(x=w345) -> (x+1=w344:dbl)
                    n1308 = local read "mistake # 4.2R"() -> (w338:dbl)
                    n1309 = local read "time (s)"() -> (w346:dbl)
                    n1310 = local read "mistake # 4.1L"() -> (w339:dbl)
                    n1311 = local read "trial #"() -> (w337:dbl)
                    n1312 = local read "ITI (s)"() -> (w335:dbl)
                    n1313 = local write "lick # 4.1L"(w344) -> ()
                    n1314 = Build Array(w346, w344, w343, w342, w341, w340, w340, w337, w336, w335, w340, w339, w338) -> (w347:dbl[])
                    n1315 = local read "Mouse path 4"() -> (w348:path)
                    n1316 = call-poly <vilib>:"Write To Spreadsheet File.vi"("append to file? (new file:F)"=TRUE, "1D data"=w347, "file path (dialog if empty)"=w348) -> ()  [unwired: 5 in, 1 out]
                  }
                  frame "ITI" {
                    w355 = 0.0 ("element")
                    n1317 = local read "water # 4.2R"() -> (w356:dbl)
                    n1318 = local read "lick # 4.2R"() -> (w358:dbl)
                    n1319 = local read "water # 4.1L"() -> (w357:dbl)
                    n1320 = local read "lick # 4.1L"() -> (w360:dbl)
                    n1321 = local read "current sound"() -> (w351:dbl)
                    n1322 = local read "trial #"() -> (w352:dbl)
                    n1323 = local read "ITI (s)"() -> (w350:dbl)
                    n1324 = Increment(x=w360) -> (x+1=w359:dbl)
                    n1325 = local read "time (s)"() -> (w361:dbl)
                    n1326 = local read "mistake # 4.1L"() -> (w354:dbl)
                    n1327 = local read "mistake # 4.2R"() -> (w353:dbl)
                    n1328 = local write "lick # 4.1L"(w359) -> ()
                    n1329 = local read "Mouse path 4"() -> (w363:path)
                    n1330 = Build Array(w361, w359, w358, w357, w356, w355, w355, w352, w351, w350, w355, w354, w353) -> (w362:dbl[])
                    n1331 = call-poly <vilib>:"Write To Spreadsheet File.vi"("append to file? (new file:F)"=TRUE, "1D data"=w362, "file path (dialog if empty)"=w363) -> ()  [unwired: 5 in, 1 out]
                  }
                }
              }
            }
          }
          frame 4 {
            n1332 = case shown="True" w420 {
              frame False {
              }
              frame True {
                n1333 = local read "state 4.2"() -> (w477:enum16{"waiting", "sound", "ITI"})
                n1334 = case shown="\"sound\"" w477 {
                  frame "waiting", Default {
                    w485 = 0.0 ("element")
                    n1335 = local read "water # 4.2R"() -> (w487:dbl)
                    n1336 = local read "lick # 4.2R"() -> (w490:dbl)
                    n1337 = local read "water # 4.1L"() -> (w488:dbl)
                    n1338 = local read "lick # 4.1L"() -> (w491:dbl)
                    n1339 = local read "current sound"() -> (w479:dbl)
                    n1340 = local read "trial #"() -> (w480:dbl)
                    n1341 = local read "mistake # 4.2R"() -> (w483:dbl)
                    n1342 = local read "time (s)"() -> (w482:dbl)
                    n1343 = local read "ITI (s)"() -> (w478:dbl)
                    n1344 = Increment(x=w490) -> (x+1=w489:dbl)
                    n1345 = local read "mistake # 4.1L"() -> (w484:dbl)
                    n1346 = Increment(x=w487) -> (x+1=w486:dbl)
                    n1347 = local write "water # 4.2R"(w486) -> ()
                    n1348 = local write "state 4.2"(enum16{"waiting", "sound", "ITI"}."ITI") -> ()
                    n1349 = local write "lick # 4.2R"(w489) -> ()
                    n1350 = local write "last water 4.2R"(w482) -> ()
                    n1351 = local read "Mouse path 4"() -> (w493:path)
                    n1352 = local write "state 4.1"(enum16{"waiting", "sound", "ITI"}."ITI") -> ()
                    n1353 = local read "free water 4.2"() -> (w495:bool)
                    n1354 = Build Array(w482, w491, w489, w488, w486, 1.0 ("element"), w485, w480, w479, w478, w485, w484, w483) -> (w492:dbl[])
                    n1355 = call-poly <vilib>:"Write To Spreadsheet File.vi"("append to file? (new file:F)"=TRUE, "1D data"=w492, "file path (dialog if empty)"=w493) -> ()  [unwired: 5 in, 1 out]
                    n1356 = case shown="False" w495 {
                      frame False {
                        n1357 = local read "water dur (ms) 4.2"() -> (w498:dbl)
                        n1358 = local read "water port 4.2"() -> (w499:tag)
                        n1359 = call "_digital_on_duration_off.vi"("duration (ms)"=w498, "digital port"=w499) -> ()  [unwired: 10 in]
                      }
                      frame True {
                      }
                    }
                  }
                  frame "sound" {
                    w503 = 0.0 ("element")
                    n1360 = local read "water # 4.2R"() -> (w506:dbl)
                    n1361 = local read "water # 4.1L"() -> (w507:dbl)
                    n1362 = local read "current sound"() -> (w501:dbl)
                    n1363 = local read "lick # 4.2R"() -> (w509:dbl)
                    n1364 = local read "trial #"() -> (w502:dbl)
                    n1365 = local read "lick # 4.1L"() -> (w510:dbl)
                    n1366 = local read "ITI (s)"() -> (w500:dbl)
                    n1367 = local read "mistake # 4.2R"() -> (w504:dbl)
                    n1368 = Increment(x=w509) -> (x+1=w508:dbl)
                    n1369 = local read "mistake # 4.1L"() -> (w505:dbl)
                    n1370 = local write "lick # 4.2R"(w508) -> ()
                    n1371 = local read "time (s)"() -> (w511:dbl)
                    n1372 = Build Array(w511, w510, w508, w507, w506, w503, w503, w502, w501, w500, w503, w505, w504) -> (w512:dbl[])
                    n1373 = local read "Mouse path 4"() -> (w513:path)
                    n1374 = call-poly <vilib>:"Write To Spreadsheet File.vi"("append to file? (new file:F)"=TRUE, "1D data"=w512, "file path (dialog if empty)"=w513) -> ()  [unwired: 5 in, 1 out]
                  }
                  frame "ITI" {
                    w520 = 0.0 ("element")
                    n1375 = local read "water # 4.2R"() -> (w521:dbl)
                    n1376 = local read "lick # 4.2R"() -> (w524:dbl)
                    n1377 = local read "water # 4.1L"() -> (w522:dbl)
                    n1378 = local read "lick # 4.1L"() -> (w525:dbl)
                    n1379 = local read "current sound"() -> (w516:dbl)
                    n1380 = local read "ITI (s)"() -> (w515:dbl)
                    n1381 = local read "trial #"() -> (w517:dbl)
                    n1382 = Increment(x=w524) -> (x+1=w523:dbl)
                    n1383 = local read "mistake # 4.2R"() -> (w518:dbl)
                    n1384 = local read "mistake # 4.1L"() -> (w519:dbl)
                    n1385 = local read "time (s)"() -> (w526:dbl)
                    n1386 = local write "lick # 4.2R"(w523) -> ()
                    n1387 = Build Array(w526, w525, w523, w522, w521, w520, w520, w517, w516, w515, w520, w519, w518) -> (w527:dbl[])
                    n1388 = local read "Mouse path 4"() -> (w528:path)
                    n1389 = call-poly <vilib>:"Write To Spreadsheet File.vi"("append to file? (new file:F)"=TRUE, "1D data"=w527, "file path (dialog if empty)"=w528) -> ()  [unwired: 5 in, 1 out]
                  }
                }
              }
            }
            n1390 = case shown="True" w421 {
              frame False {
              }
              frame True {
                n1391 = local read "state 4.2"() -> (w422:enum16{"waiting", "sound", "ITI"})
                n1392 = case shown="\"sound\"" w422 {
                  frame "waiting", Default {
                    w424 = 0.0 ("element")
                    n1393 = local read "current sound"() -> (w427:dbl)
                    n1394 = local read "trial #"() -> (w428:dbl)
                    n1395 = local read "LED 4"() -> (w430:tag)
                    n1396 = local read "water # 4.2R"() -> (w432:dbl)
                    n1397 = local read "water # 4.1L"() -> (w433:dbl)
                    n1398 = local read "lick # 4.2R"() -> (w434:dbl)
                    n1399 = local read "lick # 4.1L"() -> (w436:dbl)
                    n1400 = local read "ITI (s)"() -> (w423:dbl)
                    n1401 = local write "LED 4 (i)"(1.0 ("LED 4 (i)")) -> ()
                    n1402 = local read "mistake # 4.2R"() -> (w431:dbl)
                    n1403 = local read "mistake # 4.1L"() -> (w425:dbl)
                    n1404 = local read "time (s)"() -> (w437:dbl)
                    n1405 = Increment(x=w436) -> (x+1=w435:dbl)
                    n1406 = call "_digital_on.vi"("digital port"=w430) -> ()  [unwired: 11 in]
                    n1407 = Increment(x=w431) -> (x+1=w426:dbl)
                    n1408 = local write "lick # 4.1L"(w435) -> ()
                    n1409 = local write "mistake # 4.2R"(w426) -> ()
                    n1410 = local read "Mouse path 4"() -> (w439:path)
                    n1411 = Build Array(w437, w435, w434, w433, w432, w424, w424, w428, w427, w423, w424, w425, w426) -> (w438:dbl[])
                    n1412 = local write "state 4.1"(enum16{"waiting", "sound", "ITI"}."ITI") -> ()
                    n1413 = local write "state 4.2"(enum16{"waiting", "sound", "ITI"}."ITI") -> ()
                    n1414 = call-poly <vilib>:"Write To Spreadsheet File.vi"("append to file? (new file:F)"=TRUE, "1D data"=w438, "file path (dialog if empty)"=w439) -> ()  [unwired: 5 in, 1 out]
                  }
                  frame "sound" {
                    w452 = 0.0 ("element")
                    n1415 = local read "lick # 4.2R"() -> (w455:dbl)
                    n1416 = local read "water # 4.2R"() -> (w453:dbl)
                    n1417 = local read "current sound"() -> (w448:dbl)
                    n1418 = local read "water # 4.1L"() -> (w454:dbl)
                    n1419 = local read "lick # 4.1L"() -> (w457:dbl)
                    n1420 = local read "trial #"() -> (w449:dbl)
                    n1421 = local read "ITI (s)"() -> (w447:dbl)
                    n1422 = local read "time (s)"() -> (w458:dbl)
                    n1423 = local read "mistake # 4.2R"() -> (w450:dbl)
                    n1424 = local read "mistake # 4.1L"() -> (w451:dbl)
                    n1425 = Increment(x=w457) -> (x+1=w456:dbl)
                    n1426 = local write "lick # 4.1L"(w456) -> ()
                    n1427 = local read "Mouse path 4"() -> (w460:path)
                    n1428 = Build Array(w458, w456, w455, w454, w453, w452, w452, w449, w448, w447, w452, w451, w450) -> (w459:dbl[])
                    n1429 = local read "LED 4"() -> (w445:tag)
                    n1430 = local write "state 4.1"(enum16{"waiting", "sound", "ITI"}."ITI") -> ()
                    n1431 = local write "state 4.2"(enum16{"waiting", "sound", "ITI"}."ITI") -> ()
                    n1432 = local write "LED 4 (i)"(1.0 ("LED 4 (i)")) -> ()
                    n1433 = call-poly <vilib>:"Write To Spreadsheet File.vi"("append to file? (new file:F)"=TRUE, "1D data"=w459, "file path (dialog if empty)"=w460) -> ()  [unwired: 5 in, 1 out]
                    n1434 = call "_digital_on.vi"("digital port"=w445) -> ()  [unwired: 11 in]
                  }
                  frame "ITI" {
                    w467 = 0.0 ("element")
                    n1435 = local read "current sound"() -> (w463:dbl)
                    n1436 = local read "water # 4.2R"() -> (w468:dbl)
                    n1437 = local read "water # 4.1L"() -> (w469:dbl)
                    n1438 = local read "lick # 4.2R"() -> (w470:dbl)
                    n1439 = local read "trial #"() -> (w464:dbl)
                    n1440 = local read "lick # 4.1L"() -> (w472:dbl)
                    n1441 = local read "ITI (s)"() -> (w462:dbl)
                    n1442 = local read "time (s)"() -> (w473:dbl)
                    n1443 = local read "mistake # 4.1L"() -> (w466:dbl)
                    n1444 = local read "mistake # 4.2R"() -> (w465:dbl)
                    n1445 = Increment(x=w472) -> (x+1=w471:dbl)
                    n1446 = local write "lick # 4.1L"(w471) -> ()
                    n1447 = local read "Mouse path 4"() -> (w475:path)
                    n1448 = Build Array(w473, w471, w470, w469, w468, w467, w467, w464, w463, w462, w467, w466, w465) -> (w474:dbl[])
                    n1449 = call-poly <vilib>:"Write To Spreadsheet File.vi"("append to file? (new file:F)"=TRUE, "1D data"=w474, "file path (dialog if empty)"=w475) -> ()  [unwired: 5 in, 1 out]
                  }
                }
              }
            }
          }
        }
        n1450 = case shown="4" w72 {
          tunnel: w74 -> [_ w1412 w1523 w1636 w1746]
          tunnel: w73 -> [_ w1411 w1524 w1635 w1745]
          frame 0, Default {
          }
          frame 1 {
            n1451 = case shown="True" w1411 {
              frame False {
              }
              frame True {
                n1452 = local read "state 1.2"() -> (w1413:enum16{"waiting", "sound", "ITI"})
                n1453 = case shown="\"sound\"" w1413 {
                  frame "waiting", Default {
                    w1424 = 0
                    n1454 = local read "LED 1"() -> (w1414:tag)
                    n1455 = local read "water # 1.2R"() -> (w1418:dbl)
                    n1456 = local read "water # 1.1L"() -> (w1430:dbl)
                    n1457 = call "_digital_on.vi"("digital port"=w1414) -> ()  [unwired: 11 in]
                    n1458 = local read "lick # 1.2R"() -> (w1428:dbl)
                    n1459 = local read "lick # 1.1L"() -> (w1427:dbl)
                    n1460 = local read "current sound"() -> (w1432:dbl)
                    n1461 = local read "time (s)"() -> (w1426:dbl)
                    n1462 = local read "trial #"() -> (w1431:dbl)
                    n1463 = local write "LED 1(i)"(1.0 ("LED 1(i)")) -> ()
                    n1464 = local read "mistake # 1.1L"() -> (w1420:dbl)
                    n1465 = Increment(x=w1428) -> (x+1=w1429:dbl)
                    n1466 = local read "mistake # 1.2R"() -> (w1422:dbl)
                    n1467 = local write "lick # 1.2R"(w1429) -> ()
                    n1468 = local write "state 1.2"(enum16{"waiting", "sound", "ITI"}."ITI") -> ()
                    n1469 = local write "state 1.1"(enum16{"waiting", "sound", "ITI"}."ITI") -> ()
                    n1470 = local read "ITI (s)"() -> (w1433:dbl)
                    n1471 = Increment(x=w1420) -> (x+1=w1419:dbl)
                    n1472 = local read "Mouse path 1"() -> (w1423:path)
                    n1473 = local write "mistake # 1.1L"(w1419) -> ()
                    n1474 = Build Array(w1426, w1427, w1429, w1430, w1418, 0.0 ("element"), w1424, w1431, w1432, w1433, w1424, w1419, w1422) -> (w1434:dbl[])
                    n1475 = call-poly <vilib>:"Write To Spreadsheet File.vi"("append to file? (new file:F)"=TRUE, "1D data"=w1434, "file path (dialog if empty)"=w1423) -> ()  [unwired: 5 in, 1 out]
                  }
                  frame "ITI" {
                    w1437 = 0 ("element")
                    n1476 = local read "lick # 1.2R"() -> (w1444:dbl)
                    n1477 = local read "water # 1.1L"() -> (w1442:dbl)
                    n1478 = local read "water # 1.2R"() -> (w1441:dbl)
                    n1479 = local read "lick # 1.1L"() -> (w1445:dbl)
                    n1480 = local read "mistake # 1.2R"() -> (w1435:dbl)
                    n1481 = local read "current sound"() -> (w1439:dbl)
                    n1482 = local read "mistake # 1.1L"() -> (w1436:dbl)
                    n1483 = local read "time (s)"() -> (w1446:dbl)
                    n1484 = local read "trial #"() -> (w1440:dbl)
                    n1485 = local read "ITI (s)"() -> (w1438:dbl)
                    n1486 = Increment(x=w1444) -> (x+1=w1443:dbl)
                    n1487 = local write "lick # 1.2R"(w1443) -> ()
                    n1488 = local read "Mouse path 1"() -> (w1449:path)
                    n1489 = Build Array(w1446, w1445, w1443, w1442, w1441, w1437, w1437, w1440, w1439, w1438, w1437, w1436, w1435) -> (w1447:dbl[])
                    n1490 = call-poly <vilib>:"Write To Spreadsheet File.vi"("append to file? (new file:F)"=TRUE, "1D data"=w1447, "file path (dialog if empty)"=w1449) -> ()  [unwired: 5 in, 1 out]
                  }
                  frame "sound" {
                    w1456 = 0 ("element")
                    n1491 = local read "water # 1.2R"() -> (w1460:dbl)
                    n1492 = local read "water # 1.1L"() -> (w1461:dbl)
                    n1493 = local read "lick # 1.2R"() -> (w1463:dbl)
                    n1494 = local read "lick # 1.1L"() -> (w1464:dbl)
                    n1495 = Increment(x=w1463) -> (x+1=w1462:dbl)
                    n1496 = local read "mistake # 1.2R"() -> (w1454:dbl)
                    n1497 = local read "mistake # 1.1L"() -> (w1455:dbl)
                    n1498 = local read "current sound"() -> (w1458:dbl)
                    n1499 = local read "time (s)"() -> (w1465:dbl)
                    n1500 = local write "lick # 1.2R"(w1462) -> ()
                    n1501 = local read "ITI (s)"() -> (w1457:dbl)
                    n1502 = local read "trial #"() -> (w1459:dbl)
                    n1503 = local read "Mouse path 1"() -> (w1468:path)
                    n1504 = Build Array(w1465, w1464, w1462, w1461, w1460, w1456, w1456, w1459, w1458, w1457, w1456, w1455, w1454) -> (w1466:dbl[])
                    n1505 = local write "state 1.2"(enum16{"waiting", "sound", "ITI"}."ITI") -> ()
                    n1506 = local write "state 1.1"(enum16{"waiting", "sound", "ITI"}."ITI") -> ()
                    n1507 = call-poly <vilib>:"Write To Spreadsheet File.vi"("append to file? (new file:F)"=TRUE, "1D data"=w1466, "file path (dialog if empty)"=w1468) -> ()  [unwired: 5 in, 1 out]
                    n1508 = local read "LED 1"() -> (w1453:tag)
                    n1509 = local write "LED 1(i)"(1.0 ("LED 1(i)")) -> ()
                    n1510 = call "_digital_on.vi"("digital port"=w1453) -> ()  [unwired: 11 in]
                  }
                }
              }
            }
            n1511 = case shown="True" w1412 {
              frame False {
              }
              frame True {
                n1512 = local read "Mouse path 1"() -> (w1469:path)
                n1513 = local read "state 1.1"() -> (w1470:enum16{"waiting", "sound", "ITI"})
                n1514 = case shown="\"ITI\"" w1470 {
                  tunnel: w1469 -> [w1477 _ w1510]
                  frame "waiting", Default {
                    w1482 = 0
                    n1515 = local read "time (s)"() -> (w1489:dbl)
                    n1516 = local read "lick # 1.1L"() -> (w1488:dbl)
                    n1517 = local read "water # 1.1L"() -> (w1487:dbl)
                    n1518 = local write "state 1.2"(enum16{"waiting", "sound", "ITI"}."ITI") -> ()
                    n1519 = local write "state 1.1"(enum16{"waiting", "sound", "ITI"}."ITI") -> ()
                    n1520 = local write "last water 1.1L"(w1489) -> ()
                    n1521 = Increment(x=w1487) -> (x+1=w1485:dbl)
                    n1522 = Increment(x=w1488) -> (x+1=w1486:dbl)
                    n1523 = local write "lick # 1.1L"(w1486) -> ()
                    n1524 = local write "water # 1.1L"(w1485) -> ()
                    n1525 = local read "lick # 1.2R"() -> (w1476:dbl)
                    n1526 = local read "free water 1.1"() -> (w1473:bool)
                    n1527 = local read "current sound"() -> (w1480:dbl)
                    n1528 = local read "trial #"() -> (w1481:dbl)
                    n1529 = local read "water # 1.2R"() -> (w1484:dbl)
                    n1530 = case shown="False" w1473 {
                      frame False {
                        n1531 = call "_digital_on_duration_off.vi"("duration (ms)"="water dur (ms) 1.1", "digital port"="water port 1.1") -> ()  [unwired: 10 in]
                      }
                      frame True {
                      }
                    }
                    n1532 = local read "ITI (s)"() -> (w1479:dbl)
                    n1533 = local read "mistake # 1.1L"() -> (w1475:dbl)
                    n1534 = local read "mistake # 1.2R"() -> (w1474:dbl)
                    n1535 = Build Array(w1489, w1486, w1476, w1485, w1484, 1, w1482, w1481, w1480, w1479, w1482, w1475, w1474) -> (w1478:dbl[])
                    n1536 = call-poly <vilib>:"Write To Spreadsheet File.vi"("append to file? (new file:F)"=TRUE, "1D data"=w1478, "file path (dialog if empty)"=w1477) -> ()  [unwired: 5 in, 1 out]
                  }
                  frame "sound" {
                    w1495 = 0 ("element")
                    n1537 = local read "mistake # 1.2R"() -> (w1493:dbl)
                    n1538 = local read "water # 1.2R"() -> (w1499:dbl)
                    n1539 = local read "water # 1.1L"() -> (w1500:dbl)
                    n1540 = local read "mistake # 1.1L"() -> (w1494:dbl)
                    n1541 = local read "current sound"() -> (w1497:dbl)
                    n1542 = local read "trial #"() -> (w1498:dbl)
                    n1543 = local read "lick # 1.2R"() -> (w1501:dbl)
                    n1544 = local read "lick # 1.1L"() -> (w1503:dbl)
                    n1545 = local read "ITI (s)"() -> (w1496:dbl)
                    n1546 = Increment(x=w1503) -> (x+1=w1502:dbl)
                    n1547 = local read "time (s)"() -> (w1504:dbl)
                    n1548 = local write "lick # 1.1L"(w1502) -> ()
                    n1549 = local read "Mouse path 1"() -> (w1506:path)
                    n1550 = Build Array(w1504, w1502, w1501, w1500, w1499, w1495, w1495, w1498, w1497, w1496, w1495, w1494, w1493) -> (w1505:dbl[])
                    n1551 = call-poly <vilib>:"Write To Spreadsheet File.vi"("append to file? (new file:F)"=TRUE, "1D data"=w1505, "file path (dialog if empty)"=w1506) -> ()  [unwired: 5 in, 1 out]
                  }
                  frame "ITI" {
                    w1516 = 0
                    n1552 = local read "time (s)"() -> (w1521:dbl)
                    n1553 = local read "lick # 1.1L"() -> (w1520:dbl)
                    n1554 = local read "lick # 1.2R"() -> (w1511:dbl)
                    n1555 = Increment(x=w1520) -> (x+1=w1519:dbl)
                    n1556 = local read "water # 1.1L"() -> (w1518:dbl)
                    n1557 = local read "water # 1.2R"() -> (w1517:dbl)
                    n1558 = local write "lick # 1.1L"(w1519) -> ()
                    n1559 = local read "current sound"() -> (w1514:dbl)
                    n1560 = local read "ITI (s)"() -> (w1513:dbl)
                    n1561 = local read "trial #"() -> (w1515:dbl)
                    n1562 = local read "mistake # 1.2R"() -> (w1508:dbl)
                    n1563 = local read "mistake # 1.1L"() -> (w1509:dbl)
                    n1564 = Build Array(w1521, w1519, w1511, w1518, w1517, w1516, w1516, w1515, w1514, w1513, w1516, w1509, w1508) -> (w1512:dbl[])
                    n1565 = call-poly <vilib>:"Write To Spreadsheet File.vi"("append to file? (new file:F)"=TRUE, "1D data"=w1512, "file path (dialog if empty)"=w1510) -> ()  [unwired: 5 in, 1 out]
                  }
                }
              }
            }
          }
          frame 2 {
            n1566 = case shown="True" w1523 {
              frame False {
              }
              frame True {
                n1567 = local read "state 1.1"() -> (w1525:enum16{"waiting", "sound", "ITI"})
                n1568 = case shown="\"sound\"" w1525 {
                  frame "waiting", Default {
                    w1534 = 0
                    n1569 = local read "LED 1"() -> (w1526:tag)
                    n1570 = local read "water # 1.1L"() -> (w1528:dbl)
                    n1571 = local read "lick # 1.2R"() -> (w1540:dbl)
                    n1572 = call "_digital_on.vi"("digital port"=w1526) -> ()  [unwired: 11 in]
                    n1573 = local read "water # 1.2R"() -> (w1541:dbl)
                    n1574 = local read "time (s)"() -> (w1537:dbl)
                    n1575 = local read "current sound"() -> (w1543:dbl)
                    n1576 = local read "lick # 1.1L"() -> (w1538:dbl)
                    n1577 = local write "state 1.2"(enum16{"waiting", "sound", "ITI"}."ITI") -> ()
                    n1578 = local write "state 1.1"(enum16{"waiting", "sound", "ITI"}."ITI") -> ()
                    n1579 = local read "mistake # 1.2R"() -> (w1531:dbl)
                    n1580 = local read "ITI (s)"() -> (w1544:dbl)
                    n1581 = Increment(x=w1538) -> (x+1=w1539:dbl)
                    n1582 = local write "lick # 1.1L"(w1539) -> ()
                    n1583 = local read "mistake # 1.1L"() -> (w1533:dbl)
                    n1584 = local read "trial #"() -> (w1542:dbl)
                    n1585 = Increment(x=w1531) -> (x+1=w1530:dbl)
                    n1586 = local read "Mouse path 1"() -> (w1546:path)
                    n1587 = local write "mistake # 1.2R"(w1530) -> ()
                    n1588 = Build Array(w1537, w1539, w1540, w1528, w1541, 0.0 ("element"), w1534, w1542, w1543, w1544, w1534, w1533, w1530) -> (w1545:dbl[])
                    n1589 = call-poly <vilib>:"Write To Spreadsheet File.vi"("append to file? (new file:F)"=TRUE, "1D data"=w1545, "file path (dialog if empty)"=w1546) -> ()  [unwired: 5 in, 1 out]
                    n1590 = local write "LED 1(i)"(1.0 ("LED 1(i)")) -> ()
                  }
                  frame "ITI" {
                    w1549 = 0 ("element")
                    n1591 = local read "lick # 1.1L"() -> (w1557:dbl)
                    n1592 = local read "water # 1.2R"() -> (w1553:dbl)
                    n1593 = local read "water # 1.1L"() -> (w1554:dbl)
                    n1594 = local read "lick # 1.2R"() -> (w1555:dbl)
                    n1595 = local read "mistake # 1.2R"() -> (w1547:dbl)
                    n1596 = local read "current sound"() -> (w1551:dbl)
                    n1597 = local read "mistake # 1.1L"() -> (w1548:dbl)
                    n1598 = local read "trial #"() -> (w1552:dbl)
                    n1599 = Increment(x=w1557) -> (x+1=w1556:dbl)
                    n1600 = local read "time (s)"() -> (w1558:dbl)
                    n1601 = local read "ITI (s)"() -> (w1550:dbl)
                    n1602 = local write "lick # 1.1L"(w1556) -> ()
                    n1603 = Build Array(w1558, w1556, w1555, w1554, w1553, w1549, w1549, w1552, w1551, w1550, w1549, w1548, w1547) -> (w1559:dbl[])
                    n1604 = local read "Mouse path 1"() -> (w1561:path)
                    n1605 = call-poly <vilib>:"Write To Spreadsheet File.vi"("append to file? (new file:F)"=TRUE, "1D data"=w1559, "file path (dialog if empty)"=w1561) -> ()  [unwired: 5 in, 1 out]
                  }
                  frame "sound" {
                    w1568 = 0 ("element")
                    n1606 = local read "water # 1.2R"() -> (w1572:dbl)
                    n1607 = local read "water # 1.1L"() -> (w1573:dbl)
                    n1608 = local read "lick # 1.2R"() -> (w1574:dbl)
                    n1609 = local read "mistake # 1.2R"() -> (w1566:dbl)
                    n1610 = local read "mistake # 1.1L"() -> (w1567:dbl)
                    n1611 = local read "current sound"() -> (w1570:dbl)
                    n1612 = local read "lick # 1.1L"() -> (w1576:dbl)
                    n1613 = local read "trial #"() -> (w1571:dbl)
                    n1614 = local read "ITI (s)"() -> (w1569:dbl)
                    n1615 = local read "time (s)"() -> (w1577:dbl)
                    n1616 = Increment(x=w1576) -> (x+1=w1575:dbl)
                    n1617 = local write "lick # 1.1L"(w1575) -> ()
                    n1618 = local read "Mouse path 1"() -> (w1580:path)
                    n1619 = Build Array(w1577, w1575, w1574, w1573, w1572, w1568, w1568, w1571, w1570, w1569, w1568, w1567, w1566) -> (w1578:dbl[])
                    n1620 = local read "LED 1"() -> (w1564:tag)
                    n1621 = call-poly <vilib>:"Write To Spreadsheet File.vi"("append to file? (new file:F)"=TRUE, "1D data"=w1578, "file path (dialog if empty)"=w1580) -> ()  [unwired: 5 in, 1 out]
                    n1622 = local write "state 1.2"(enum16{"waiting", "sound", "ITI"}."ITI") -> ()
                    n1623 = local write "state 1.1"(enum16{"waiting", "sound", "ITI"}."ITI") -> ()
                    n1624 = call "_digital_on.vi"("digital port"=w1564) -> ()  [unwired: 11 in]
                    n1625 = local write "LED 1(i)"(1.0 ("LED 1(i)")) -> ()
                  }
                }
              }
            }
            n1626 = case shown="True" w1524 {
              frame False {
              }
              frame True {
                n1627 = local read "Mouse path 1"() -> (w1581:path)
                n1628 = local read "state 1.2"() -> (w1582:enum16{"waiting", "sound", "ITI"})
                n1629 = case shown="\"sound\"" w1582 {
                  tunnel: w1581 -> [w1590 _ w1622]
                  frame "waiting", Default {
                    w1596 = 0
                    n1630 = local read "lick # 1.1L"() -> (w1589:dbl)
                    n1631 = local read "lick # 1.2R"() -> (w1588:dbl)
                    n1632 = local read "time (s)"() -> (w1601:dbl)
                    n1633 = local read "water # 1.2R"() -> (w1599:dbl)
                    n1634 = Increment(x=w1588) -> (x+1=w1587:dbl)
                    n1635 = local write "last water 1.2R"(w1601) -> ()
                    n1636 = local write "lick # 1.2R"(w1587) -> ()
                    n1637 = Increment(x=w1599) -> (x+1=w1598:dbl)
                    n1638 = local read "free water 1.2"() -> (w1584:bool)
                    n1639 = local write "water # 1.2R"(w1598) -> ()
                    n1640 = case shown="False" w1584 {
                      frame False {
                        n1641 = call "_digital_on_duration_off.vi"("duration (ms)"="water dur (ms) 1.2", "digital port"="water port 1.2") -> ()  [unwired: 10 in]
                      }
                      frame True {
                      }
                    }
                    n1642 = local read "water # 1.1L"() -> (w1600:dbl)
                    n1643 = local read "current sound"() -> (w1594:dbl)
                    n1644 = local read "trial #"() -> (w1595:dbl)
                    n1645 = local read "mistake # 1.2R"() -> (w1585:dbl)
                    n1646 = local read "mistake # 1.1L"() -> (w1586:dbl)
                    n1647 = local read "ITI (s)"() -> (w1593:dbl)
                    n1648 = Build Array(w1601, w1589, w1587, w1600, w1598, 1, w1596, w1595, w1594, w1593, w1596, w1586, w1585) -> (w1592:dbl[])
                    n1649 = local write "state 1.1"(enum16{"waiting", "sound", "ITI"}."ITI") -> ()
                    n1650 = local write "state 1.2"(enum16{"waiting", "sound", "ITI"}."ITI") -> ()
                    n1651 = call-poly <vilib>:"Write To Spreadsheet File.vi"("append to file? (new file:F)"=TRUE, "1D data"=w1592, "file path (dialog if empty)"=w1590) -> ()  [unwired: 5 in, 1 out]
                  }
                  frame "sound" {
                    w1607 = 0 ("element")
                    n1652 = local read "water # 1.2R"() -> (w1611:dbl)
                    n1653 = local read "water # 1.1L"() -> (w1612:dbl)
                    n1654 = local read "lick # 1.1L"() -> (w1614:dbl)
                    n1655 = local read "lick # 1.2R"() -> (w1615:dbl)
                    n1656 = local read "current sound"() -> (w1609:dbl)
                    n1657 = local read "mistake # 1.1L"() -> (w1606:dbl)
                    n1658 = local read "ITI (s)"() -> (w1608:dbl)
                    n1659 = local read "mistake # 1.2R"() -> (w1605:dbl)
                    n1660 = local read "trial #"() -> (w1610:dbl)
                    n1661 = local read "time (s)"() -> (w1616:dbl)
                    n1662 = Increment(x=w1615) -> (x+1=w1613:dbl)
                    n1663 = local write "lick # 1.2R"(w1613) -> ()
                    n1664 = local read "Mouse path 1"() -> (w1619:path)
                    n1665 = Build Array(w1616, w1614, w1613, w1612, w1611, w1607, w1607, w1610, w1609, w1608, w1607, w1606, w1605) -> (w1617:dbl[])
                    n1666 = call-poly <vilib>:"Write To Spreadsheet File.vi"("append to file? (new file:F)"=TRUE, "1D data"=w1617, "file path (dialog if empty)"=w1619) -> ()  [unwired: 5 in, 1 out]
                  }
                  frame "ITI" {
                    w1628 = 0
                    n1667 = local read "lick # 1.1L"() -> (w1623:dbl)
                    n1668 = local read "lick # 1.2R"() -> (w1632:dbl)
                    n1669 = local read "time (s)"() -> (w1633:dbl)
                    n1670 = Increment(x=w1632) -> (x+1=w1631:dbl)
                    n1671 = local write "lick # 1.2R"(w1631) -> ()
                    n1672 = local read "water # 1.1L"() -> (w1630:dbl)
                    n1673 = local read "current sound"() -> (w1626:dbl)
                    n1674 = local read "water # 1.2R"() -> (w1629:dbl)
                    n1675 = local read "trial #"() -> (w1627:dbl)
                    n1676 = local read "mistake # 1.1L"() -> (w1621:dbl)
                    n1677 = local read "mistake # 1.2R"() -> (w1620:dbl)
                    n1678 = local read "ITI (s)"() -> (w1625:dbl)
                    n1679 = Build Array(w1633, w1623, w1631, w1630, w1629, w1628, w1628, w1627, w1626, w1625, w1628, w1621, w1620) -> (w1624:dbl[])
                    n1680 = call-poly <vilib>:"Write To Spreadsheet File.vi"("append to file? (new file:F)"=TRUE, "1D data"=w1624, "file path (dialog if empty)"=w1622) -> ()  [unwired: 5 in, 1 out]
                  }
                }
              }
            }
          }
          frame 3 {
            n1681 = case shown="True" w1636 {
              frame False {
              }
              frame True {
                n1682 = local read "state 1.1"() -> (w1692:enum16{"waiting", "sound", "ITI"})
                n1683 = case shown="\"waiting\", Default" w1692 {
                  frame "waiting", Default {
                    w1697 = 0 ("element")
                    n1684 = local read "water # 1.2R"() -> (w1702:dbl)
                    n1685 = local read "water # 1.1L"() -> (w1704:dbl)
                    n1686 = local read "lick # 1.2R"() -> (w1705:dbl)
                    n1687 = local read "lick # 1.1L"() -> (w1707:dbl)
                    n1688 = local read "time (s)"() -> (w1708:dbl)
                    n1689 = Increment(x=w1704) -> (x+1=w1703:dbl)
                    n1690 = Increment(x=w1707) -> (x+1=w1706:dbl)
                    n1691 = local write "state 1.1"(enum16{"waiting", "sound", "ITI"}."ITI") -> ()
                    n1692 = local write "water # 1.1L"(w1703) -> ()
                    n1693 = local read "Mouse path 1"() -> (w1710:path)
                    n1694 = local write "lick # 1.1L"(w1706) -> ()
                    n1695 = local write "last water 1.1L"(w1708) -> ()
                    n1696 = local read "current sound"() -> (w1699:dbl)
                    n1697 = local read "mistake # 1.2R"() -> (w1695:dbl)
                    n1698 = local read "mistake # 1.1L"() -> (w1696:dbl)
                    n1699 = local read "ITI (s)"() -> (w1698:dbl)
                    n1700 = local read "trial #"() -> (w1700:dbl)
                    n1701 = local read "free water 1.1"() -> (w1693:bool)
                    n1702 = local write "state 1.2"(enum16{"waiting", "sound", "ITI"}."ITI") -> ()
                    n1703 = case shown="False" w1693 {
                      frame False {
                        n1704 = local read "water port 1.1"() -> (w1713:tag)
                        n1705 = local read "water dur (ms) 1.1"() -> (w1714:dbl)
                        n1706 = call "_digital_on_duration_off.vi"("duration (ms)"=w1714, "digital port"=w1713) -> ()  [unwired: 10 in]
                      }
                      frame True {
                      }
                    }
                    n1707 = Build Array(w1708, w1706, w1705, w1703, w1702, 1 ("element"), w1697, w1700, w1699, w1698, w1697, w1696, w1695) -> (w1709:dbl[])
                    n1708 = call-poly <vilib>:"Write To Spreadsheet File.vi"("append to file? (new file:F)"=TRUE, "1D data"=w1709, "file path (dialog if empty)"=w1710) -> ()  [unwired: 5 in, 1 out]
                  }
                  frame "ITI" {
                    w1717 = 0 ("element")
                    n1709 = local read "water # 1.2R"() -> (w1721:dbl)
                    n1710 = local read "water # 1.1L"() -> (w1722:dbl)
                    n1711 = local read "lick # 1.1L"() -> (w1725:dbl)
                    n1712 = local read "lick # 1.2R"() -> (w1723:dbl)
                    n1713 = local read "current sound"() -> (w1719:dbl)
                    n1714 = local read "trial #"() -> (w1720:dbl)
                    n1715 = local read "ITI (s)"() -> (w1718:dbl)
                    n1716 = local read "time (s)"() -> (w1726:dbl)
                    n1717 = Increment(x=w1725) -> (x+1=w1724:dbl)
                    n1718 = local read "mistake # 1.1L"() -> (w1716:dbl)
                    n1719 = local read "mistake # 1.2R"() -> (w1715:dbl)
                    n1720 = local write "lick # 1.1L"(w1724) -> ()
                    n1721 = local read "Mouse path 1"() -> (w1729:path)
                    n1722 = Build Array(w1726, w1724, w1723, w1722, w1721, w1717, w1717, w1720, w1719, w1718, w1717, w1716, w1715) -> (w1727:dbl[])
                    n1723 = call-poly <vilib>:"Write To Spreadsheet File.vi"("append to file? (new file:F)"=TRUE, "1D data"=w1727, "file path (dialog if empty)"=w1729) -> ()  [unwired: 5 in, 1 out]
                  }
                  frame "sound" {
                    w1732 = 0 ("element")
                    n1724 = local read "water # 1.2R"() -> (w1736:dbl)
                    n1725 = local read "water # 1.1L"() -> (w1737:dbl)
                    n1726 = local read "lick # 1.2R"() -> (w1738:dbl)
                    n1727 = local read "lick # 1.1L"() -> (w1740:dbl)
                    n1728 = local read "current sound"() -> (w1734:dbl)
                    n1729 = local read "mistake # 1.2R"() -> (w1730:dbl)
                    n1730 = local read "ITI (s)"() -> (w1733:dbl)
                    n1731 = local read "trial #"() -> (w1735:dbl)
                    n1732 = local read "mistake # 1.1L"() -> (w1731:dbl)
                    n1733 = local read "time (s)"() -> (w1741:dbl)
                    n1734 = Increment(x=w1740) -> (x+1=w1739:dbl)
                    n1735 = local write "lick # 1.1L"(w1739) -> ()
                    n1736 = local read "Mouse path 1"() -> (w1744:path)
                    n1737 = Build Array(w1741, w1739, w1738, w1737, w1736, w1732, w1732, w1735, w1734, w1733, w1732, w1731, w1730) -> (w1742:dbl[])
                    n1738 = call-poly <vilib>:"Write To Spreadsheet File.vi"("append to file? (new file:F)"=TRUE, "1D data"=w1742, "file path (dialog if empty)"=w1744) -> ()  [unwired: 5 in, 1 out]
                  }
                }
              }
            }
            n1739 = case shown="True" w1635 {
              frame False {
              }
              frame True {
                n1740 = local read "state 1.2"() -> (w1637:enum16{"waiting", "sound", "ITI"})
                n1741 = case shown="\"sound\"" w1637 {
                  frame "waiting", Default {
                    w1644 = 0 ("element")
                    n1742 = local read "water # 1.2R"() -> (w1648:dbl)
                    n1743 = local read "water # 1.1L"() -> (w1649:dbl)
                    n1744 = local read "lick # 1.2R"() -> (w1651:dbl)
                    n1745 = local read "lick # 1.1L"() -> (w1652:dbl)
                    n1746 = local read "current sound"() -> (w1646:dbl)
                    n1747 = local read "mistake # 1.1L"() -> (w1642:dbl)
                    n1748 = Increment(x=w1651) -> (x+1=w1650:dbl)
                    n1749 = local read "time (s)"() -> (w1653:dbl)
                    n1750 = local read "mistake # 1.2R"() -> (w1643:dbl)
                    n1751 = local read "trial #"() -> (w1647:dbl)
                    n1752 = local read "ITI (s)"() -> (w1645:dbl)
                    n1753 = local write "lick # 1.2R"(w1650) -> ()
                    n1754 = local write "state 1.1"(enum16{"waiting", "sound", "ITI"}."ITI") -> ()
                    n1755 = Increment(x=w1642) -> (x+1=w1641:dbl)
                    n1756 = local read "Mouse path 1"() -> (w1656:path)
                    n1757 = local write "mistake # 1.1L"(w1641) -> ()
                    n1758 = local write "LED 1(i)"(1.0 ("LED 1(i)")) -> ()
                    n1759 = Build Array(w1653, w1652, w1650, w1649, w1648, w1644, w1644, w1647, w1646, w1645, w1644, w1641, w1643) -> (w1655:dbl[])
                    n1760 = call-poly <vilib>:"Write To Spreadsheet File.vi"("append to file? (new file:F)"=TRUE, "1D data"=w1655, "file path (dialog if empty)"=w1656) -> ()  [unwired: 5 in, 1 out]
                    n1761 = local read "LED 1"() -> (w1638:tag)
                    n1762 = local write "state 1.2"(enum16{"waiting", "sound", "ITI"}."ITI") -> ()
                    n1763 = call "_digital_on.vi"("digital port"=w1638) -> ()  [unwired: 11 in]
                  }
                  frame "sound" {
                    w1664 = 0 ("element")
                    n1764 = local write "state 1.1"(enum16{"waiting", "sound", "ITI"}."ITI") -> ()
                    n1765 = local write "state 1.2"(enum16{"waiting", "sound", "ITI"}."ITI") -> ()
                    n1766 = local read "water # 1.2R"() -> (w1668:dbl)
                    n1767 = local read "water # 1.1L"() -> (w1669:dbl)
                    n1768 = local read "lick # 1.2R"() -> (w1671:dbl)
                    n1769 = local read "current sound"() -> (w1666:dbl)
                    n1770 = local read "mistake # 1.2R"() -> (w1662:dbl)
                    n1771 = local read "lick # 1.1L"() -> (w1672:dbl)
                    n1772 = local read "ITI (s)"() -> (w1665:dbl)
                    n1773 = local read "mistake # 1.1L"() -> (w1663:dbl)
                    n1774 = local read "trial #"() -> (w1667:dbl)
                    n1775 = Increment(x=w1671) -> (x+1=w1670:dbl)
                    n1776 = local read "time (s)"() -> (w1673:dbl)
                    n1777 = local write "lick # 1.2R"(w1670) -> ()
                    n1778 = local read "LED 1"() -> (w1660:tag)
                    n1779 = local read "Mouse path 1"() -> (w1675:path)
                    n1780 = Build Array(w1673, w1672, w1670, w1669, w1668, w1664, w1664, w1667, w1666, w1665, w1664, w1663, w1662) -> (w1674:dbl[])
                    n1781 = call "_digital_on.vi"("digital port"=w1660) -> ()  [unwired: 11 in]
                    n1782 = local write "LED 1(i)"(1.0 ("LED 1(i)")) -> ()
                    n1783 = call-poly <vilib>:"Write To Spreadsheet File.vi"("append to file? (new file:F)"=TRUE, "1D data"=w1674, "file path (dialog if empty)"=w1675) -> ()  [unwired: 5 in, 1 out]
                  }
                  frame "ITI" {
                    w1679 = 0 ("element")
                    n1784 = local read "water # 1.2R"() -> (w1683:dbl)
                    n1785 = local read "water # 1.1L"() -> (w1684:dbl)
                    n1786 = local read "lick # 1.2R"() -> (w1686:dbl)
                    n1787 = local read "current sound"() -> (w1681:dbl)
                    n1788 = local read "lick # 1.1L"() -> (w1687:dbl)
                    n1789 = local read "mistake # 1.2R"() -> (w1677:dbl)
                    n1790 = local read "mistake # 1.1L"() -> (w1678:dbl)
                    n1791 = local read "trial #"() -> (w1682:dbl)
                    n1792 = local read "ITI (s)"() -> (w1680:dbl)
                    n1793 = local read "time (s)"() -> (w1688:dbl)
                    n1794 = Increment(x=w1686) -> (x+1=w1685:dbl)
                    n1795 = local write "lick # 1.2R"(w1685) -> ()
                    n1796 = local read "Mouse path 1"() -> (w1691:path)
                    n1797 = Build Array(w1688, w1687, w1685, w1684, w1683, w1679, w1679, w1682, w1681, w1680, w1679, w1678, w1677) -> (w1689:dbl[])
                    n1798 = call-poly <vilib>:"Write To Spreadsheet File.vi"("append to file? (new file:F)"=TRUE, "1D data"=w1689, "file path (dialog if empty)"=w1691) -> ()  [unwired: 5 in, 1 out]
                  }
                }
              }
            }
          }
          frame 4 {
            n1799 = case shown="True" w1746 {
              frame False {
              }
              frame True {
                n1800 = local read "state 1.1"() -> (w1800:enum16{"waiting", "sound", "ITI"})
                n1801 = case shown="\"waiting\", Default" w1800 {
                  frame "waiting", Default {
                    w1801 = 0 ("element")
                    n1802 = local read "water # 1.1L"() -> (w1812:dbl)
                    n1803 = local read "lick # 1.2R"() -> (w1813:dbl)
                    n1804 = local read "lick # 1.1L"() -> (w1815:dbl)
                    n1805 = local read "water # 1.2R"() -> (w1811:dbl)
                    n1806 = local read "mistake # 1.2R"() -> (w1807:dbl)
                    n1807 = local read "mistake # 1.1L"() -> (w1802:dbl)
                    n1808 = local read "current sound"() -> (w1809:dbl)
                    n1809 = local read "time (s)"() -> (w1816:dbl)
                    n1810 = Increment(x=w1815) -> (x+1=w1814:dbl)
                    n1811 = local read "trial #"() -> (w1810:dbl)
                    n1812 = local read "ITI (s)"() -> (w1808:dbl)
                    n1813 = local write "state 1.2"(enum16{"waiting", "sound", "ITI"}."ITI") -> ()
                    n1814 = local write "state 1.1"(enum16{"waiting", "sound", "ITI"}."ITI") -> ()
                    n1815 = local write "lick # 1.1L"(w1814) -> ()
                    n1816 = Increment(x=w1807) -> (x+1=w1803:dbl)
                    n1817 = local write "mistake # 1.2R"(w1803) -> ()
                    n1818 = local read "Mouse path 1"() -> (w1819:path)
                    n1819 = Build Array(w1816, w1814, w1813, w1812, w1811, w1801, w1801, w1810, w1809, w1808, w1801, w1802, w1803) -> (w1817:dbl[])
                    n1820 = local read "LED 1"() -> (w1804:tag)
                    n1821 = call-poly <vilib>:"Write To Spreadsheet File.vi"("append to file? (new file:F)"=TRUE, "1D data"=w1817, "file path (dialog if empty)"=w1819) -> ()  [unwired: 5 in, 1 out]
                    n1822 = call "_digital_on.vi"("digital port"=w1804) -> ()  [unwired: 11 in]
                    n1823 = local write "LED 1(i)"(1.0 ("LED 1(i)")) -> ()
                  }
                  frame "sound" {
                    w1827 = 0 ("element")
                    n1824 = local read "water # 1.2R"() -> (w1831:dbl)
                    n1825 = local read "water # 1.1L"() -> (w1832:dbl)
                    n1826 = local read "lick # 1.2R"() -> (w1833:dbl)
                    n1827 = local read "mistake # 1.2R"() -> (w1825:dbl)
                    n1828 = local read "current sound"() -> (w1829:dbl)
                    n1829 = local read "lick # 1.1L"() -> (w1835:dbl)
                    n1830 = local read "mistake # 1.1L"() -> (w1826:dbl)
                    n1831 = local write "state 1.2"(enum16{"waiting", "sound", "ITI"}."ITI") -> ()
                    n1832 = local write "state 1.1"(enum16{"waiting", "sound", "ITI"}."ITI") -> ()
                    n1833 = local read "trial #"() -> (w1830:dbl)
                    n1834 = local read "ITI (s)"() -> (w1828:dbl)
                    n1835 = local read "time (s)"() -> (w1836:dbl)
                    n1836 = Increment(x=w1835) -> (x+1=w1834:dbl)
                    n1837 = local read "Mouse path 1"() -> (w1839:path)
                    n1838 = local write "lick # 1.1L"(w1834) -> ()
                    n1839 = local read "LED 1"() -> (w1823:tag)
                    n1840 = Build Array(w1836, w1834, w1833, w1832, w1831, w1827, w1827, w1830, w1829, w1828, w1827, w1826, w1825) -> (w1837:dbl[])
                    n1841 = local write "LED 1(i)"(1.0 ("LED 1(i)")) -> ()
                    n1842 = call-poly <vilib>:"Write To Spreadsheet File.vi"("append to file? (new file:F)"=TRUE, "1D data"=w1837, "file path (dialog if empty)"=w1839) -> ()  [unwired: 5 in, 1 out]
                    n1843 = call "_digital_on.vi"("digital port"=w1823) -> ()  [unwired: 11 in]
                  }
                  frame "ITI" {
                    w1842 = 0 ("element")
                    n1844 = local read "water # 1.2R"() -> (w1846:dbl)
                    n1845 = local read "lick # 1.1L"() -> (w1850:dbl)
                    n1846 = local read "water # 1.1L"() -> (w1847:dbl)
                    n1847 = local read "lick # 1.2R"() -> (w1848:dbl)
                    n1848 = local read "mistake # 1.2R"() -> (w1840:dbl)
                    n1849 = local read "current sound"() -> (w1844:dbl)
                    n1850 = local read "mistake # 1.1L"() -> (w1841:dbl)
                    n1851 = Increment(x=w1850) -> (x+1=w1849:dbl)
                    n1852 = local read "trial #"() -> (w1845:dbl)
                    n1853 = local read "time (s)"() -> (w1851:dbl)
                    n1854 = local read "ITI (s)"() -> (w1843:dbl)
                    n1855 = local write "lick # 1.1L"(w1849) -> ()
                    n1856 = local read "Mouse path 1"() -> (w1854:path)
                    n1857 = Build Array(w1851, w1849, w1848, w1847, w1846, w1842, w1842, w1845, w1844, w1843, w1842, w1841, w1840) -> (w1852:dbl[])
                    n1858 = call-poly <vilib>:"Write To Spreadsheet File.vi"("append to file? (new file:F)"=TRUE, "1D data"=w1852, "file path (dialog if empty)"=w1854) -> ()  [unwired: 5 in, 1 out]
                  }
                }
              }
            }
            n1859 = case shown="True" w1745 {
              frame False {
              }
              frame True {
                n1860 = local read "state 1.2"() -> (w1747:enum16{"waiting", "sound", "ITI"})
                n1861 = case shown="\"waiting\", Default" w1747 {
                  frame "waiting", Default {
                    w1752 = 0 ("element")
                    n1862 = local read "water # 1.2R"() -> (w1758:dbl)
                    n1863 = local read "lick # 1.2R"() -> (w1761:dbl)
                    n1864 = local read "free water 1.2"() -> (w1748:bool)
                    n1865 = local read "water # 1.1L"() -> (w1759:dbl)
                    n1866 = local read "lick # 1.1L"() -> (w1762:dbl)
                    n1867 = local read "time (s)"() -> (w1763:dbl)
                    n1868 = local write "state 1.2"(enum16{"waiting", "sound", "ITI"}."ITI") -> ()
                    n1869 = local write "state 1.1"(enum16{"waiting", "sound", "ITI"}."ITI") -> ()
                    n1870 = Increment(x=w1758) -> (x+1=w1757:dbl)
                    n1871 = Increment(x=w1761) -> (x+1=w1760:dbl)
                    n1872 = case shown="False" w1748 {
                      frame False {
                        n1873 = local read "water dur (ms) 1.2"() -> (w1769:dbl)
                        n1874 = local read "water port 1.2"() -> (w1768:tag)
                        n1875 = call "_digital_on_duration_off.vi"("duration (ms)"=w1769, "digital port"=w1768) -> ()  [unwired: 10 in]
                      }
                      frame True {
                      }
                    }
                    n1876 = local write "water # 1.2R"(w1757) -> ()
                    n1877 = local write "lick # 1.2R"(w1760) -> ()
                    n1878 = local write "last water 1.2R"(w1763) -> ()
                    n1879 = local read "mistake # 1.2R"() -> (w1750:dbl)
                    n1880 = local read "mistake # 1.1L"() -> (w1751:dbl)
                    n1881 = local read "current sound"() -> (w1754:dbl)
                    n1882 = local read "ITI (s)"() -> (w1753:dbl)
                    n1883 = local read "trial #"() -> (w1755:dbl)
                    n1884 = local read "Mouse path 1"() -> (w1766:path)
                    n1885 = Build Array(w1763, w1762, w1760, w1759, w1757, 1 ("element"), w1752, w1755, w1754, w1753, w1752, w1751, w1750) -> (w1764:dbl[])
                    n1886 = call-poly <vilib>:"Write To Spreadsheet File.vi"("append to file? (new file:F)"=TRUE, "1D data"=w1764, "file path (dialog if empty)"=w1766) -> ()  [unwired: 5 in, 1 out]
                  }
                  frame "sound" {
                    w1772 = 0 ("element")
                    n1887 = local read "lick # 1.2R"() -> (w1779:dbl)
                    n1888 = local read "water # 1.2R"() -> (w1776:dbl)
                    n1889 = local read "water # 1.1L"() -> (w1777:dbl)
                    n1890 = local read "lick # 1.1L"() -> (w1780:dbl)
                    n1891 = local read "mistake # 1.2R"() -> (w1770:dbl)
                    n1892 = local read "current sound"() -> (w1774:dbl)
                    n1893 = Increment(x=w1779) -> (x+1=w1778:dbl)
                    n1894 = local read "mistake # 1.1L"() -> (w1771:dbl)
                    n1895 = local read "time (s)"() -> (w1781:dbl)
                    n1896 = local read "trial #"() -> (w1775:dbl)
                    n1897 = local read "ITI (s)"() -> (w1773:dbl)
                    n1898 = local write "lick # 1.2R"(w1778) -> ()
                    n1899 = local read "Mouse path 1"() -> (w1784:path)
                    n1900 = Build Array(w1781, w1780, w1778, w1777, w1776, w1772, w1772, w1775, w1774, w1773, w1772, w1771, w1770) -> (w1782:dbl[])
                    n1901 = call-poly <vilib>:"Write To Spreadsheet File.vi"("append to file? (new file:F)"=TRUE, "1D data"=w1782, "file path (dialog if empty)"=w1784) -> ()  [unwired: 5 in, 1 out]
                  }
                  frame "ITI" {
                    w1787 = 0 ("element")
                    n1902 = local read "water # 1.2R"() -> (w1791:dbl)
                    n1903 = local read "water # 1.1L"() -> (w1792:dbl)
                    n1904 = local read "lick # 1.2R"() -> (w1794:dbl)
                    n1905 = local read "lick # 1.1L"() -> (w1795:dbl)
                    n1906 = local read "mistake # 1.2R"() -> (w1785:dbl)
                    n1907 = local read "current sound"() -> (w1789:dbl)
                    n1908 = local read "mistake # 1.1L"() -> (w1786:dbl)
                    n1909 = Increment(x=w1794) -> (x+1=w1793:dbl)
                    n1910 = local read "ITI (s)"() -> (w1788:dbl)
                    n1911 = local read "trial #"() -> (w1790:dbl)
                    n1912 = local read "time (s)"() -> (w1796:dbl)
                    n1913 = local write "lick # 1.2R"(w1793) -> ()
                    n1914 = local read "Mouse path 1"() -> (w1799:path)
                    n1915 = Build Array(w1796, w1795, w1793, w1792, w1791, w1787, w1787, w1790, w1789, w1788, w1787, w1786, w1785) -> (w1797:dbl[])
                    n1916 = call-poly <vilib>:"Write To Spreadsheet File.vi"("append to file? (new file:F)"=TRUE, "1D data"=w1797, "file path (dialog if empty)"=w1799) -> ()  [unwired: 5 in, 1 out]
                  }
                }
              }
            }
          }
        }
        n1917 = call "_loop_time.vi"("from shift register"=w85) -> ("to shift register"=w84:dbl)  [unwired: 9 in, 1 out]
        n1918 = call "Elapsed Time"() -> ("Elapsed Time (s)"=→"time (s)":dbl)  [unwired: 12 in, 7 out]
      }
      n1919 = call <vilib>:"DAQmx Clear Task.vi"("task in"=w31) -> ()  [unwired: 14 in, 1 out]
      n1920 = while {
        shift-right: [w1858] -> _
        shift-left: T1."prepare" -> [w1857]
        stop <- FALSE stop-if-true
        n1921 = local write "trial state"(w1857) -> ()
        n1922 = case shown="\"graph\"" w1857 {
          tunnel: [w1859 w1939 w1988 w2003 w2009 T1."ITI" T1."prepare"] -> w1858
          frame "prepare", Default {
            n1923 = flat-sequence {
              tunnel: [T1."sound"] -> w1859
              frame #0 {
                w1863 = 500
                w1870 = 1000
                n1924 = Subtract(x="ITI max (ms)", y=w1863) -> (x-y=w1866:dbl)
                n1925 = Subtract(x="ITI min (ms)", y=w1863) -> (x-y=w1867:dbl)
                n1926 = local read "next sound"() -> (w1873:dbl[])
                n1927 = Divide(x=w1866, y=w1870) -> (x/y=w1861:dbl)
                n1928 = Divide(x=w1867, y=w1870) -> (x/y=w1860:dbl)
                n1929 = Delete From Array(array=w1873, index=0) -> (deleted portion=w1871:dbl, array with subset deleted=w1872:dbl[])  [unwired: 1 in]
                n1930 = local write "next sound"(w1872) -> ()
                n1931 = call "_random_integer.vi"("max"=w1861, "min"=w1860) -> ("output"=w1864:dbl)  [unwired: 9 in]
                n1932 = local write "current sound"(w1871) -> ()
                n1933 = Add(x=w1864, y=0.5) -> (x+y=w1865:dbl)
                n1934 = local write "ITI (s)"(w1865) -> ()
              }
              frame #1 {
                n1935 = local read "trial #"() -> (w1936:dbl)
                n1936 = local read "water # 3.2R"() -> (w1898:dbl)
                n1937 = local read "water # 3.1L"() -> (w1899:dbl)
                n1938 = local read "water # 2.2R"() -> (w1913:dbl)
                n1939 = local read "lick # 3.2R"() -> (w1900:dbl)
                n1940 = local read "current sound"() -> (w1879:dbl)
                n1941 = local read "water # 4.2R"() -> (w1883:dbl)
                n1942 = Increment(x=w1936) -> (x+1=w1880:dbl)
                n1943 = local read "water # 2.1L"() -> (w1914:dbl)
                n1944 = local read "water # 4.1L"() -> (w1884:dbl)
                n1945 = local read "mistake # 4.1L"() -> (w1876:dbl)
                n1946 = local read "mistake # 4.2R"() -> (w1875:dbl)
                n1947 = local read "lick # 3.1L"() -> (w1901:dbl)
                n1948 = local read "lick # 4.2R"() -> (w1885:dbl)
                n1949 = local read "lick # 4.1L"() -> (w1886:dbl)
                n1950 = local read "current sound"() -> (w1895:dbl)
                n1951 = local read "lick  #  2.1L"() -> (w1916:dbl)
                n1952 = local read "ITI (s)"() -> (w1878:dbl)
                n1953 = local read "lick  #  2.2R"() -> (w1915:dbl)
                n1954 = local read "ITI (s)"() -> (w1894:dbl)
                n1955 = local read "current sound"() -> (w1910:dbl)
                n1956 = local write "trial #"(w1880) -> ()
                n1957 = local read "time (s)"() -> (w1902:dbl)
                n1958 = local read "water # 1.2R"() -> (w1924:dbl)
                n1959 = local read "mistake # 2.2R"() -> (w1906:dbl)
                n1960 = local read "ITI (s)"() -> (w1909:dbl)
                n1961 = local read "mistake # 3.2R"() -> (w1891:dbl)
                n1962 = local read "mistake # 3.1L"() -> (w1892:dbl)
                n1963 = local read "time (s)"() -> (w1887:dbl)
                n1964 = local read "water # 1.1L"() -> (w1925:dbl)
                n1965 = local read "mistake # 1.2R"() -> (w1921:dbl)
                n1966 = local read "lick # 1.1L"() -> (w1927:dbl)
                n1967 = local read "mistake # 2.1L"() -> (w1907:dbl)
                n1968 = local read "lick # 1.2R"() -> (w1926:dbl)
                n1969 = local read "mistake # 1.1L"() -> (w1922:dbl)
                n1970 = local read "current sound"() -> (w1931:dbl)
                n1971 = local read "time (s)"() -> (w1917:dbl)
                n1972 = local read "time (s)"() -> (w1933:dbl)
                n1973 = local read "ITI (s)"() -> (w1930:dbl)
                n1974 = local read "Mouse path 1"() -> (w1935:path)
                n1975 = local read "Mouse path 2"() -> (w1918:path)
                n1976 = Build Array(w1887, w1886, w1885, w1884, w1883, 0.0 ("element"), 1.0 ("element"), w1880, w1879, w1878, 0.0 ("element"), w1876, w1875) -> (w1888:dbl[])
                n1977 = Build Array(w1902, w1901, w1900, w1899, w1898, 0.0 ("element"), 1 ("element"), w1880, w1895, w1894, 0.0 ("element"), w1892, w1891) -> (w1904:dbl[])
                n1978 = local read "Mouse path 4"() -> (w1889:path)
                n1979 = Build Array(w1917, w1916, w1915, w1914, w1913, 0.0 ("element"), 1 ("element"), w1880, w1910, w1909, 0 ("element"), w1907, w1906) -> (w1919:dbl[])
                n1980 = local read "Mouse path 3"() -> (w1903:path)
                n1981 = Build Array(w1933, w1927, w1926, w1925, w1924, 0.0 ("element"), 1, w1880, w1931, w1930, 0, w1922, w1921) -> (w1928:dbl[])
                n1982 = call-poly <vilib>:"Write To Spreadsheet File.vi"("append to file? (new file:F)"=TRUE, "1D data"=w1919, "file path (dialog if empty)"=w1918) -> ()  [unwired: 5 in, 1 out]
                n1983 = call-poly <vilib>:"Write To Spreadsheet File.vi"("append to file? (new file:F)"=TRUE, "1D data"=w1928, "file path (dialog if empty)"=w1935) -> ()  [unwired: 5 in, 1 out]
                n1984 = call-poly <vilib>:"Write To Spreadsheet File.vi"("append to file? (new file:F)"=TRUE, "1D data"=w1888, "file path (dialog if empty)"=w1889) -> ()  [unwired: 5 in, 1 out]
                n1985 = call-poly <vilib>:"Write To Spreadsheet File.vi"("append to file? (new file:F)"=TRUE, "1D data"=w1904, "file path (dialog if empty)"=w1903) -> ()  [unwired: 5 in, 1 out]
              }
              frame #2 {
                w1937 = enum16{"waiting", "sound", "ITI"}."sound"
                n1986 = local write "state 1.2"(w1937) -> ()
                n1987 = local write "state 1.1"(w1937) -> ()
                n1988 = local write "state 3.2"(w1937) -> ()
                n1989 = local write "state 3.1"(w1937) -> ()
                n1990 = local write "state 4.2"(w1937) -> ()
                n1991 = local write "state 2.1"(w1937) -> ()
                n1992 = local write "state 2.2"(w1937) -> ()
                n1993 = local write "state 4.1"(w1937) -> ()
              }
              frame #3 {
              }
            }
          }
          frame "sound" {
            n1994 = flat-sequence {
              tunnel: [T1."free water"] -> w1939
              frame #0 {
                n1995 = local read "current sound"() -> (w1945:dbl)
                n1996 = case shown="3" w1945 {
                  tunnel: "sound dur (ms)" -> [w1950 w1955 w1960 w1964]
                  tunnel: "sound port 1" -> [w1947 _ w1957 _]
                  tunnel: "sound port 2" -> [_ w1952 _ w1965]
                  tunnel: "sound file 1" -> [w1946 _ _ w1961]
                  tunnel: "sound file 2" -> [_ w1951 w1956 _]
                  frame ..1 {
                    n1997 = local read "Left Speaker"() -> (w1949:dbl)
                    n1998 = Increment(x=w1949) -> (x+1=w1948:dbl)
                    n1999 = local write "Left Speaker"(w1948) -> ()
                    n2000 = call "_play_wave_file.vi"("sound length (ms)"=w1950, "sound file"=w1946, "sound port"=w1947) -> ()  [unwired: 9 in]
                  }
                  frame 2 {
                    n2001 = local read "Right Speaker"() -> (w1954:dbl)
                    n2002 = Increment(x=w1954) -> (x+1=w1953:dbl)
                    n2003 = call "_play_wave_file.vi"("sound length (ms)"=w1955, "sound file"=w1951, "sound port"=w1952) -> ()  [unwired: 9 in]
                    n2004 = local write "Right Speaker"(w1953) -> ()
                  }
                  frame 3 {
                    n2005 = local read "Left Speaker"() -> (w1959:dbl)
                    n2006 = call "_play_wave_file.vi"("sound length (ms)"=w1960, "sound file"=w1956, "sound port"=w1957) -> ()  [unwired: 9 in]
                    n2007 = Increment(x=w1959) -> (x+1=w1958:dbl)
                    n2008 = local write "Left Speaker"(w1958) -> ()
                  }
                  frame 4.. {
                    n2009 = local read "Right Speaker"() -> (w1963:dbl)
                    n2010 = Increment(x=w1963) -> (x+1=w1962:dbl)
                    n2011 = call "_play_wave_file.vi"("sound length (ms)"=w1964, "sound file"=w1961, "sound port"=w1965) -> ()  [unwired: 9 in]
                    n2012 = local write "Right Speaker"(w1962) -> ()
                  }
                }
              }
              frame #1 {
                n2013 = local read "LED 1(i)"() -> (w1969:dbl)
                n2014 = local read "LED 2 (i)"() -> (w1968:dbl)
                n2015 = local read "LED 3 (i)"() -> (w1967:dbl)
                n2016 = local read "LED 4 (i)"() -> (w1966:dbl)
                n2017 = case shown="1" w1969 {
                  frame 0, Default {
                  }
                  frame 1 {
                    n2018 = local read "fault # 1"() -> (w1984:dbl)
                    n2019 = local read "LED 1"() -> (w1982:tag)
                    n2020 = Increment(x=w1984) -> (x+1=w1983:dbl)
                    n2021 = local write "LED 1(i)"(0.0 ("LED 1(i)")) -> ()
                    n2022 = local write "fault # 1"(w1983) -> ()
                    n2023 = call "_digital_off.vi"("digital port"=w1982) -> ()  [unwired: 11 in]
                  }
                }
                n2024 = case shown="1" w1968 {
                  frame 0, Default {
                  }
                  frame 1 {
                    n2025 = local read "fault # 2"() -> (w1980:dbl)
                    n2026 = local read "LED 2"() -> (w1978:tag)
                    n2027 = Increment(x=w1980) -> (x+1=w1979:dbl)
                    n2028 = local write "LED 2 (i)"(0.0 ("LED 2 (i)")) -> ()
                    n2029 = call "_digital_off.vi"("digital port"=w1978) -> ()  [unwired: 11 in]
                    n2030 = local write "fault # 2"(w1979) -> ()
                  }
                }
                n2031 = case shown="1" w1966 {
                  frame 0, Default {
                  }
                  frame 1 {
                    n2032 = local read "fault # 4"() -> (w1972:dbl)
                    n2033 = local read "LED 4"() -> (w1970:tag)
                    n2034 = Increment(x=w1972) -> (x+1=w1971:dbl)
                    n2035 = local write "LED 4 (i)"(0.0 ("LED 4 (i)")) -> ()
                    n2036 = call "_digital_off.vi"("digital port"=w1970) -> ()  [unwired: 11 in]
                    n2037 = local write "fault # 4"(w1971) -> ()
                  }
                }
                n2038 = case shown="1" w1967 {
                  frame 0, Default {
                  }
                  frame 1 {
                    n2039 = local read "fault # 3"() -> (w1976:dbl)
                    n2040 = local read "LED 3"() -> (w1974:tag)
                    n2041 = Increment(x=w1976) -> (x+1=w1975:dbl)
                    n2042 = local write "LED 3 (i)"(0.0 ("LED 3 (i)")) -> ()
                    n2043 = call "_digital_off.vi"("digital port"=w1974) -> ()  [unwired: 11 in]
                    n2044 = local write "fault # 3"(w1975) -> ()
                  }
                }
              }
              frame #2 {
                w1986 = enum16{"waiting", "sound", "ITI"}."waiting"
                n2045 = local write "state 1.1"(w1986) -> ()
                n2046 = local write "state 1.2"(w1986) -> ()
                n2047 = local write "state 2.1"(w1986) -> ()
                n2048 = local write "state 2.2"(w1986) -> ()
                n2049 = local write "state 3.2"(w1986) -> ()
                n2050 = local write "state 3.1"(w1986) -> ()
                n2051 = local write "state 4.1"(w1986) -> ()
                n2052 = local write "state 4.2"(w1986) -> ()
              }
              frame #3 {
              }
            }
          }
          frame "reaction window" {
            n2053 = flat-sequence {
              tunnel: [T1."graph"] -> w1988
              frame #0 {
                n2054 = Wait (ms)(milliseconds to wait="reaction dur (ms)") -> ()  [unwired: 1 out]
              }
              frame #1 {
                n2055 = local read "LED 2 (i)"() -> (w1992:dbl)
                n2056 = local read "LED 3 (i)"() -> (w1991:dbl)
                n2057 = local read "LED 1(i)"() -> (w1993:dbl)
                n2058 = local read "LED 4 (i)"() -> (w1990:dbl)
                n2059 = case shown="1" w1992 {
                  frame 0, Default {
                  }
                  frame 1 {
                    n2060 = local read "LED 2"() -> (w1999:tag)
                    n2061 = local write "LED 2 (i)"(0.0 ("LED 2 (i)")) -> ()
                    n2062 = call "_digital_on_LED.vi"("digital port"=w1999) -> ()  [unwired: 11 in]
                  }
                }
                n2063 = case shown="1" w1993 {
                  frame 0, Default {
                  }
                  frame 1 {
                    n2064 = local write "LED 1(i)"(0.0 ("LED 1(i)")) -> ()
                    n2065 = call "_digital_on_LED.vi"("digital port"="LED 1") -> ()  [unwired: 11 in]
                  }
                }
                n2066 = case shown="1" w1991 {
                  frame 0, Default {
                  }
                  frame 1 {
                    n2067 = local read "LED 3"() -> (w1997:tag)
                    n2068 = local write "LED 3 (i)"(0.0 ("LED 3 (i)")) -> ()
                    n2069 = call "_digital_on_LED.vi"("digital port"=w1997) -> ()  [unwired: 11 in]
                  }
                }
                n2070 = case shown="1" w1990 {
                  frame 0, Default {
                  }
                  frame 1 {
                    n2071 = local read "LED 4"() -> (w1995:tag)
                    n2072 = local write "LED 4 (i)"(0.0 ("LED 4 (i)")) -> ()
                    n2073 = call "_digital_on_LED.vi"("digital port"=w1995) -> ()  [unwired: 11 in]
                  }
                }
              }
              frame #2 {
              }
            }
          }
          frame "ITI" {
            n2074 = flat-sequence {
              tunnel: [T1."prepare"] -> w2003
              frame #0 {
                w2004 = enum16{"waiting", "sound", "ITI"}."ITI"
                n2075 = local write "state 1.1"(w2004) -> ()
                n2076 = local write "state 4.1"(w2004) -> ()
                n2077 = local write "state 1.2"(w2004) -> ()
                n2078 = local write "state 4.2"(w2004) -> ()
                n2079 = local write "state 2.2"(w2004) -> ()
                n2080 = local write "state 3.1"(w2004) -> ()
                n2081 = local write "state 2.1"(w2004) -> ()
                n2082 = local write "state 3.2"(w2004) -> ()
              }
              frame #1 {
                n2083 = local read "ITI (s)"() -> (w2007:dbl)
                n2084 = Multiply(x=w2007, y=1000) -> (x*y=w2005:dbl)
                n2085 = Wait (ms)(milliseconds to wait=w2005) -> ()  [unwired: 1 out]
              }
              frame #2 {
              }
            }
          }
          frame "free water" {
            n2086 = flat-sequence {
              tunnel: [T1."reaction window"] -> w2009
              frame #0 {
                n2087 = local read "state 4.2"() -> (w2013:enum16{"waiting", "sound", "ITI"})
                n2088 = local read "state 4.1"() -> (w2014:enum16{"waiting", "sound", "ITI"})
                n2089 = local read "state 1.1"() -> (w2038:enum16{"waiting", "sound", "ITI"})
                n2090 = local read "state 1.2"() -> (w2037:enum16{"waiting", "sound", "ITI"})
                n2091 = local read "state 2.1"() -> (w2025:enum16{"waiting", "sound", "ITI"})
                n2092 = local read "state 2.2"() -> (w2024:enum16{"waiting", "sound", "ITI"})
                n2093 = local read "state 3.1"() -> (w2021:enum16{"waiting", "sound", "ITI"})
                n2094 = local read "state 3.2"() -> (w2020:enum16{"waiting", "sound", "ITI"})
                n2095 = Build Array(w2038, w2037, w2025, w2024, w2021, w2020, w2014, w2013) -> (w2036:enum16{"waiting", "sound", "ITI"}[])
                n2096 = local write "free water 1.1"("free water 1.1") -> ()
                n2097 = local write "free water 1.2"("free water 1.2") -> ()
                n2098 = local write "free water 2.1"("free water 2.1") -> ()
                n2099 = local write "free water 3.1"("free water 3.1") -> ()
                n2100 = local write "free water 2.2"("free water 2.2") -> ()
                n2101 = local write "free water 3.2"("free water 3.2") -> ()
                n2102 = local write "free water 4.2"("free water 4.2") -> ()
                n2103 = local write "free water 4.1"("free water 4.1") -> ()
                n2104 = Build Array("free water 1.1", "free water 1.2", "free water 2.1", "free water 2.2", "free water 3.1", "free water 3.2", "free water 4.1", "free water 4.2") -> (w2040:bool[])
                n2105 = Equal?(x=w2036, y=enum16{"waiting", "water", "ITI"}."waiting") -> (x = y?=w2041:bool[])
                n2106 = And(x=w2041, y=w2040) -> (x .and. y?=w2039:bool[])
                n2107 = Index Array(array=w2039) -> (element #1=w2034:bool, element #2=w2031:bool, element #3=w2027:bool, element #4=w2026:bool, element #5=w2018:bool, element #6=w2017:bool, element #7=w2011:bool, element #8=w2010:bool)  [unwired: 8 in]
                n2108 = local read "current sound"() -> (w2035:dbl)
                n2109 = local read "current sound"() -> (w2028:dbl)
                n2110 = local read "current sound"() -> (w2012:dbl)
                n2111 = local read "current sound"() -> (w2019:dbl)
                n2112 = case shown="4" w2028 {
                  tunnel: w2027 -> [_ w2187 _ w2223 _]
                  tunnel: w2026 -> [_ _ w2205 _ w2241]
                  frame 0, Default {
                  }
                  frame 1 {
                    n2113 = case shown="True" w2187 {
                      frame False {
                      }
                      frame True {
                        w2194 = 0.0 ("element")
                        n2114 = local read "water # 2.1L"() -> (w2196:dbl)
                        n2115 = local read "water dur (ms) 2.1"() -> (w2203:dbl)
                        n2116 = local read "water # 2.2R"() -> (w2195:dbl)
                        n2117 = local read "water port 2.1"() -> (w2204:tag)
                        n2118 = local read "lick  #  2.2R"() -> (w2197:dbl)
                        n2119 = local read "lick  #  2.1L"() -> (w2198:dbl)
                        n2120 = local read "time (s)"() -> (w2199:dbl)
                        n2121 = local read "mistake # 2.2R"() -> (w2188:dbl)
                        n2122 = local read "current sound"() -> (w2192:dbl)
                        n2123 = local read "mistake # 2.1L"() -> (w2189:dbl)
                        n2124 = local read "ITI (s)"() -> (w2191:dbl)
                        n2125 = local read "trial #"() -> (w2193:dbl)
                        n2126 = local read "Mouse path 2"() -> (w2200:path)
                        n2127 = call "_digital_on_duration_off.vi"("duration (ms)"=w2203, "digital port"=w2204) -> ()  [unwired: 10 in]
                        n2128 = Build Array(w2199, w2198, w2197, w2196, w2195, w2194, w2194, w2193, w2192, w2191, 1.0 ("element"), w2189, w2188) -> (w2202:dbl[])
                        n2129 = call-poly <vilib>:"Write To Spreadsheet File.vi"("append to file? (new file:F)"=TRUE, "1D data"=w2202, "file path (dialog if empty)"=w2200) -> ()  [unwired: 5 in, 1 out]
                      }
                    }
                  }
                  frame 2 {
                    n2130 = case shown="True" w2205 {
                      frame False {
                      }
                      frame True {
                        w2212 = 0.0 ("element")
                        n2131 = local read "water # 2.2R"() -> (w2213:dbl)
                        n2132 = local read "water # 2.1L"() -> (w2214:dbl)
                        n2133 = local read "lick  #  2.2R"() -> (w2215:dbl)
                        n2134 = local read "lick  #  2.1L"() -> (w2216:dbl)
                        n2135 = local read "current sound"() -> (w2210:dbl)
                        n2136 = local read "ITI (s)"() -> (w2209:dbl)
                        n2137 = local read "trial #"() -> (w2211:dbl)
                        n2138 = local read "time (s)"() -> (w2217:dbl)
                        n2139 = local read "water dur (ms) 2.2"() -> (w2221:dbl)
                        n2140 = local read "mistake # 2.2R"() -> (w2206:dbl)
                        n2141 = local read "water port 2.2"() -> (w2222:tag)
                        n2142 = local read "mistake # 2.1L"() -> (w2207:dbl)
                        n2143 = local read "Mouse path 2"() -> (w2218:path)
                        n2144 = Build Array(w2217, w2216, w2215, w2214, w2213, w2212, w2212, w2211, w2210, w2209, 1.0 ("element"), w2207, w2206) -> (w2219:dbl[])
                        n2145 = call "_digital_on_duration_off.vi"("duration (ms)"=w2221, "digital port"=w2222) -> ()  [unwired: 10 in]
                        n2146 = call-poly <vilib>:"Write To Spreadsheet File.vi"("append to file? (new file:F)"=TRUE, "1D data"=w2219, "file path (dialog if empty)"=w2218) -> ()  [unwired: 5 in, 1 out]
                      }
                    }
                  }
                  frame 3 {
                    n2147 = case shown="True" w2223 {
                      frame False {
                      }
                      frame True {
                        w2230 = 0.0 ("element")
                        n2148 = local read "water # 2.2R"() -> (w2231:dbl)
                        n2149 = local read "water # 2.1L"() -> (w2232:dbl)
                        n2150 = local read "lick  #  2.1L"() -> (w2234:dbl)
                        n2151 = local read "lick  #  2.2R"() -> (w2233:dbl)
                        n2152 = local read "current sound"() -> (w2228:dbl)
                        n2153 = local read "time (s)"() -> (w2235:dbl)
                        n2154 = local read "ITI (s)"() -> (w2227:dbl)
                        n2155 = local read "trial #"() -> (w2229:dbl)
                        n2156 = local read "water dur (ms) 2.1"() -> (w2239:dbl)
                        n2157 = local read "mistake # 2.2R"() -> (w2224:dbl)
                        n2158 = local read "mistake # 2.1L"() -> (w2225:dbl)
                        n2159 = local read "water port 2.1"() -> (w2240:tag)
                        n2160 = local read "Mouse path 2"() -> (w2236:path)
                        n2161 = call "_digital_on_duration_off.vi"("duration (ms)"=w2239, "digital port"=w2240) -> ()  [unwired: 10 in]
                        n2162 = Build Array(w2235, w2234, w2233, w2232, w2231, w2230, w2230, w2229, w2228, w2227, 1.0 ("element"), w2225, w2224) -> (w2237:dbl[])
                        n2163 = call-poly <vilib>:"Write To Spreadsheet File.vi"("append to file? (new file:F)"=TRUE, "1D data"=w2237, "file path (dialog if empty)"=w2236) -> ()  [unwired: 5 in, 1 out]
                      }
                    }
                  }
                  frame 4 {
                    n2164 = case shown="True" w2241 {
                      frame False {
                      }
                      frame True {
                        w2248 = 0.0 ("element")
                        n2165 = local read "water # 2.2R"() -> (w2249:dbl)
                        n2166 = local read "water # 2.1L"() -> (w2250:dbl)
                        n2167 = local read "lick  #  2.2R"() -> (w2251:dbl)
                        n2168 = local read "current sound"() -> (w2246:dbl)
                        n2169 = local read "lick  #  2.1L"() -> (w2252:dbl)
                        n2170 = local read "ITI (s)"() -> (w2245:dbl)
                        n2171 = local read "trial #"() -> (w2247:dbl)
                        n2172 = local read "mistake # 2.2R"() -> (w2242:dbl)
                        n2173 = local read "mistake # 2.1L"() -> (w2243:dbl)
                        n2174 = local read "time (s)"() -> (w2253:dbl)
                        n2175 = local read "water dur (ms) 2.2"() -> (w2257:dbl)
                        n2176 = local read "water port 2.2"() -> (w2258:tag)
                        n2177 = local read "Mouse path 2"() -> (w2255:path)
                        n2178 = Build Array(w2253, w2252, w2251, w2250, w2249, w2248, w2248, w2247, w2246, w2245, 1.0 ("element"), w2243, w2242) -> (w2254:dbl[])
                        n2179 = call "_digital_on_duration_off.vi"("duration (ms)"=w2257, "digital port"=w2258) -> ()  [unwired: 10 in]
                        n2180 = call-poly <vilib>:"Write To Spreadsheet File.vi"("append to file? (new file:F)"=TRUE, "1D data"=w2254, "file path (dialog if empty)"=w2255) -> ()  [unwired: 5 in, 1 out]
                      }
                    }
                  }
                }
                n2181 = case shown="4" w2035 {
                  tunnel: w2034 -> [_ w2259 _ w2295 _]
                  tunnel: w2031 -> [_ _ w2277 _ w2313]
                  frame 0, Default {
                  }
                  frame 1 {
                    n2182 = case shown="True" w2259 {
                      frame False {
                      }
                      frame True {
                        w2266 = 0
                        n2183 = local read "water # 1.1L"() -> (w2263:dbl)
                        n2184 = local read "water # 1.2R"() -> (w2262:dbl)
                        n2185 = local read "water port 1.1"() -> (w2268:tag)
                        n2186 = local read "water dur (ms) 1.1"() -> (w2267:dbl)
                        n2187 = local read "lick # 1.2R"() -> (w2264:dbl)
                        n2188 = local read "lick # 1.1L"() -> (w2265:dbl)
                        n2189 = local read "current sound"() -> (w2272:dbl)
                        n2190 = local read "mistake # 1.2R"() -> (w2260:dbl)
                        n2191 = local read "trial #"() -> (w2273:dbl)
                        n2192 = local read "time (s)"() -> (w2274:dbl)
                        n2193 = local read "mistake # 1.1L"() -> (w2261:dbl)
                        n2194 = local read "ITI (s)"() -> (w2271:dbl)
                        n2195 = call "_digital_on_duration_off.vi"("duration (ms)"=w2267, "digital port"=w2268) -> ()  [unwired: 10 in]
                        n2196 = local read "Mouse path 1"() -> (w2275:path)
                        n2197 = Build Array(w2274, w2265, w2264, w2263, w2262, w2266, w2266, w2273, w2272, w2271, 1, w2261, w2260) -> (w2269:dbl[])
                        n2198 = call-poly <vilib>:"Write To Spreadsheet File.vi"("append to file? (new file:F)"=TRUE, "1D data"=w2269, "file path (dialog if empty)"=w2275) -> ()  [unwired: 5 in, 1 out]
                      }
                    }
                  }
                  frame 2 {
                    n2199 = case shown="True" w2277 {
                      frame False {
                      }
                      frame True {
                        w2286 = 0 ("element")
                        n2200 = local read "water # 1.1L"() -> (w2281:dbl)
                        n2201 = local read "lick # 1.2R"() -> (w2282:dbl)
                        n2202 = local read "water # 1.2R"() -> (w2280:dbl)
                        n2203 = local read "mistake # 1.2R"() -> (w2278:dbl)
                        n2204 = local read "lick # 1.1L"() -> (w2283:dbl)
                        n2205 = local read "current sound"() -> (w2289:dbl)
                        n2206 = local read "mistake # 1.1L"() -> (w2279:dbl)
                        n2207 = local read "trial #"() -> (w2290:dbl)
                        n2208 = local read "ITI (s)"() -> (w2288:dbl)
                        n2209 = local read "time (s)"() -> (w2291:dbl)
                        n2210 = local read "water dur (ms) 1.2"() -> (w2284:dbl)
                        n2211 = Build Array(w2291, w2283, w2282, w2281, w2280, w2286, w2286, w2290, w2289, w2288, 1 ("element"), w2279, w2278) -> (w2292:dbl[])
                        n2212 = local read "Mouse path 1"() -> (w2293:path)
                        n2213 = local read "water port 1.2"() -> (w2285:tag)
                        n2214 = call-poly <vilib>:"Write To Spreadsheet File.vi"("append to file? (new file:F)"=TRUE, "1D data"=w2292, "file path (dialog if empty)"=w2293) -> ()  [unwired: 5 in, 1 out]
                        n2215 = call "_digital_on_duration_off.vi"("duration (ms)"=w2284, "digital port"=w2285) -> ()  [unwired: 10 in]
                      }
                    }
                  }
                  frame 3 {
                    n2216 = case shown="True" w2295 {
                      frame False {
                      }
                      frame True {
                        w2302 = 0.0 ("element")
                        n2217 = local read "lick # 1.2R"() -> (w2305:dbl)
                        n2218 = local read "water # 1.2R"() -> (w2303:dbl)
                        n2219 = local read "water # 1.1L"() -> (w2304:dbl)
                        n2220 = local read "lick # 1.1L"() -> (w2306:dbl)
                        n2221 = local read "time (s)"() -> (w2307:dbl)
                        n2222 = local read "current sound"() -> (w2300:dbl)
                        n2223 = local read "mistake # 1.1L"() -> (w2297:dbl)
                        n2224 = local read "mistake # 1.2R"() -> (w2296:dbl)
                        n2225 = local read "trial #"() -> (w2301:dbl)
                        n2226 = local read "ITI (s)"() -> (w2299:dbl)
                        n2227 = local read "water dur (ms) 1.1"() -> (w2311:dbl)
                        n2228 = local read "water port 1.1"() -> (w2312:tag)
                        n2229 = local read "Mouse path 1"() -> (w2308:path)
                        n2230 = Build Array(w2307, w2306, w2305, w2304, w2303, w2302, w2302, w2301, w2300, w2299, 1.0 ("element"), w2297, w2296) -> (w2309:dbl[])
                        n2231 = call "_digital_on_duration_off.vi"("duration (ms)"=w2311, "digital port"=w2312) -> ()  [unwired: 10 in]
                        n2232 = call-poly <vilib>:"Write To Spreadsheet File.vi"("append to file? (new file:F)"=TRUE, "1D data"=w2309, "file path (dialog if empty)"=w2308) -> ()  [unwired: 5 in, 1 out]
                      }
                    }
                  }
                  frame 4 {
                    n2233 = case shown="True" w2313 {
                      frame False {
                      }
                      frame True {
                        w2320 = 0.0 ("element")
                        n2234 = local read "water # 1.1L"() -> (w2322:dbl)
                        n2235 = local read "water # 1.2R"() -> (w2321:dbl)
                        n2236 = local read "lick # 1.2R"() -> (w2323:dbl)
                        n2237 = local read "lick # 1.1L"() -> (w2324:dbl)
                        n2238 = local read "water dur (ms) 1.2"() -> (w2329:dbl)
                        n2239 = local read "current sound"() -> (w2318:dbl)
                        n2240 = local read "time (s)"() -> (w2325:dbl)
                        n2241 = local read "water port 1.2"() -> (w2330:tag)
                        n2242 = local read "trial #"() -> (w2319:dbl)
                        n2243 = local read "ITI (s)"() -> (w2317:dbl)
                        n2244 = local read "mistake # 1.2R"() -> (w2314:dbl)
                        n2245 = local read "mistake # 1.1L"() -> (w2315:dbl)
                        n2246 = local read "Mouse path 1"() -> (w2326:path)
                        n2247 = call "_digital_on_duration_off.vi"("duration (ms)"=w2329, "digital port"=w2330) -> ()  [unwired: 10 in]
                        n2248 = Build Array(w2325, w2324, w2323, w2322, w2321, w2320, w2320, w2319, w2318, w2317, 1.0 ("element"), w2315, w2314) -> (w2327:dbl[])
                        n2249 = call-poly <vilib>:"Write To Spreadsheet File.vi"("append to file? (new file:F)"=TRUE, "1D data"=w2327, "file path (dialog if empty)"=w2326) -> ()  [unwired: 5 in, 1 out]
                      }
                    }
                  }
                }
                n2250 = case shown="4" w2019 {
                  tunnel: w2018 -> [_ w2115 _ w2151 _]
                  tunnel: w2017 -> [_ _ w2133 _ w2169]
                  frame 0, Default {
                  }
                  frame 1 {
                    n2251 = case shown="True" w2115 {
                      frame False {
                      }
                      frame True {
                        w2122 = 0.0 ("element")
                        n2252 = local read "water # 3.2R"() -> (w2123:dbl)
                        n2253 = local read "water # 3.1L"() -> (w2124:dbl)
                        n2254 = local read "current sound"() -> (w2120:dbl)
                        n2255 = local read "lick # 3.2R"() -> (w2125:dbl)
                        n2256 = local read "lick # 3.1L"() -> (w2126:dbl)
                        n2257 = local read "mistake # 3.2R"() -> (w2116:dbl)
                        n2258 = local read "trial #"() -> (w2121:dbl)
                        n2259 = local read "mistake # 3.1L"() -> (w2117:dbl)
                        n2260 = local read "ITI (s)"() -> (w2119:dbl)
                        n2261 = local read "time (s)"() -> (w2127:dbl)
                        n2262 = local read "water dur (ms) 3.1"() -> (w2131:dbl)
                        n2263 = local read "water port 3.1"() -> (w2132:tag)
                        n2264 = local read "Mouse path 3"() -> (w2129:path)
                        n2265 = Build Array(w2127, w2126, w2125, w2124, w2123, w2122, w2122, w2121, w2120, w2119, 1.0 ("element"), w2117, w2116) -> (w2128:dbl[])
                        n2266 = call "_digital_on_duration_off.vi"("duration (ms)"=w2131, "digital port"=w2132) -> ()  [unwired: 10 in]
                        n2267 = call-poly <vilib>:"Write To Spreadsheet File.vi"("append to file? (new file:F)"=TRUE, "1D data"=w2128, "file path (dialog if empty)"=w2129) -> ()  [unwired: 5 in, 1 out]
                      }
                    }
                  }
                  frame 2 {
                    n2268 = case shown="True" w2133 {
                      frame False {
                      }
                      frame True {
                        w2140 = 0.0 ("element")
                        n2269 = local read "water # 3.2R"() -> (w2141:dbl)
                        n2270 = local read "water # 3.1L"() -> (w2142:dbl)
                        n2271 = local read "current sound"() -> (w2138:dbl)
                        n2272 = local read "mistake # 3.2R"() -> (w2134:dbl)
                        n2273 = local read "lick # 3.2R"() -> (w2143:dbl)
                        n2274 = local read "mistake # 3.1L"() -> (w2135:dbl)
                        n2275 = local read "lick # 3.1L"() -> (w2144:dbl)
                        n2276 = local read "trial #"() -> (w2139:dbl)
                        n2277 = local read "ITI (s)"() -> (w2137:dbl)
                        n2278 = local read "time (s)"() -> (w2145:dbl)
                        n2279 = local read "water dur (ms) 3. 2"() -> (w2149:dbl)
                        n2280 = local read "Mouse path 3"() -> (w2147:path)
                        n2281 = local read "water port 3.2"() -> (w2150:tag)
                        n2282 = Build Array(w2145, w2144, w2143, w2142, w2141, w2140, w2140, w2139, w2138, w2137, 1.0 ("element"), w2135, w2134) -> (w2146:dbl[])
                        n2283 = call-poly <vilib>:"Write To Spreadsheet File.vi"("append to file? (new file:F)"=TRUE, "1D data"=w2146, "file path (dialog if empty)"=w2147) -> ()  [unwired: 5 in, 1 out]
                        n2284 = call "_digital_on_duration_off.vi"("duration (ms)"=w2149, "digital port"=w2150) -> ()  [unwired: 10 in]
                      }
                    }
                  }
                  frame 3 {
                    n2285 = case shown="True" w2151 {
                      frame False {
                      }
                      frame True {
                        w2158 = 0.0 ("element")
                        n2286 = local read "water # 3.1L"() -> (w2160:dbl)
                        n2287 = local read "water # 3.2R"() -> (w2159:dbl)
                        n2288 = local read "lick # 3.1L"() -> (w2162:dbl)
                        n2289 = local read "lick # 3.2R"() -> (w2161:dbl)
                        n2290 = local read "current sound"() -> (w2156:dbl)
                        n2291 = local read "ITI (s)"() -> (w2155:dbl)
                        n2292 = local read "trial #"() -> (w2157:dbl)
                        n2293 = local read "mistake # 3.2R"() -> (w2152:dbl)
                        n2294 = local read "time (s)"() -> (w2163:dbl)
                        n2295 = local read "mistake # 3.1L"() -> (w2153:dbl)
                        n2296 = local read "water dur (ms) 3.1"() -> (w2167:dbl)
                        n2297 = local read "water port 3.1"() -> (w2168:tag)
                        n2298 = local read "Mouse path 3"() -> (w2165:path)
                        n2299 = Build Array(w2163, w2162, w2161, w2160, w2159, w2158, w2158, w2157, w2156, w2155, 1.0 ("element"), w2153, w2152) -> (w2164:dbl[])
                        n2300 = call "_digital_on_duration_off.vi"("duration (ms)"=w2167, "digital port"=w2168) -> ()  [unwired: 10 in]
                        n2301 = call-poly <vilib>:"Write To Spreadsheet File.vi"("append to file? (new file:F)"=TRUE, "1D data"=w2164, "file path (dialog if empty)"=w2165) -> ()  [unwired: 5 in, 1 out]
                      }
                    }
                  }
                  frame 4 {
                    n2302 = case shown="True" w2169 {
                      frame False {
                      }
                      frame True {
                        w2176 = 0.0 ("element")
                        n2303 = local read "water # 3.1L"() -> (w2178:dbl)
                        n2304 = local read "water # 3.2R"() -> (w2177:dbl)
                        n2305 = local read "current sound"() -> (w2174:dbl)
                        n2306 = local read "lick # 3.2R"() -> (w2179:dbl)
                        n2307 = local read "lick # 3.1L"() -> (w2180:dbl)
                        n2308 = local read "trial #"() -> (w2175:dbl)
                        n2309 = local read "ITI (s)"() -> (w2173:dbl)
                        n2310 = local read "time (s)"() -> (w2181:dbl)
                        n2311 = local read "mistake # 3.1L"() -> (w2171:dbl)
                        n2312 = local read "mistake # 3.2R"() -> (w2170:dbl)
                        n2313 = local read "water dur (ms) 3. 2"() -> (w2185:dbl)
                        n2314 = local read "water port 3.2"() -> (w2186:tag)
                        n2315 = local read "Mouse path 3"() -> (w2183:path)
                        n2316 = Build Array(w2181, w2180, w2179, w2178, w2177, w2176, w2176, w2175, w2174, w2173, 1.0 ("element"), w2171, w2170) -> (w2182:dbl[])
                        n2317 = call "_digital_on_duration_off.vi"("duration (ms)"=w2185, "digital port"=w2186) -> ()  [unwired: 10 in]
                        n2318 = call-poly <vilib>:"Write To Spreadsheet File.vi"("append to file? (new file:F)"=TRUE, "1D data"=w2182, "file path (dialog if empty)"=w2183) -> ()  [unwired: 5 in, 1 out]
                      }
                    }
                  }
                }
                n2319 = case shown="4" w2012 {
                  tunnel: w2011 -> [_ w2043 _ w2079 _]
                  tunnel: w2010 -> [_ _ w2061 _ w2097]
                  frame 0, Default {
                  }
                  frame 1 {
                    n2320 = case shown="True" w2043 {
                      frame False {
                      }
                      frame True {
                        w2050 = 0.0 ("element")
                        n2321 = local read "water # 4.1L"() -> (w2052:dbl)
                        n2322 = local read "water # 4.2R"() -> (w2051:dbl)
                        n2323 = local read "lick # 4.2R"() -> (w2053:dbl)
                        n2324 = local read "lick # 4.1L"() -> (w2054:dbl)
                        n2325 = local read "current sound"() -> (w2048:dbl)
                        n2326 = local read "mistake # 4.2R"() -> (w2044:dbl)
                        n2327 = local read "mistake # 4.1L"() -> (w2045:dbl)
                        n2328 = local read "ITI (s)"() -> (w2047:dbl)
                        n2329 = local read "trial #"() -> (w2049:dbl)
                        n2330 = local read "time (s)"() -> (w2055:dbl)
                        n2331 = local read "water dur (ms) 4.1"() -> (w2059:dbl)
                        n2332 = local read "water port 4.1"() -> (w2060:tag)
                        n2333 = local read "Mouse path 4"() -> (w2056:path)
                        n2334 = Build Array(w2055, w2054, w2053, w2052, w2051, w2050, w2050, w2049, w2048, w2047, 1.0 ("element"), w2045, w2044) -> (w2057:dbl[])
                        n2335 = call "_digital_on_duration_off.vi"("duration (ms)"=w2059, "digital port"=w2060) -> ()  [unwired: 10 in]
                        n2336 = call-poly <vilib>:"Write To Spreadsheet File.vi"("append to file? (new file:F)"=TRUE, "1D data"=w2057, "file path (dialog if empty)"=w2056) -> ()  [unwired: 5 in, 1 out]
                      }
                    }
                  }
                  frame 2 {
                    n2337 = case shown="True" w2061 {
                      frame False {
                      }
                      frame True {
                        w2068 = 0.0 ("element")
                        n2338 = local read "lick # 4.2R"() -> (w2071:dbl)
                        n2339 = local read "current sound"() -> (w2066:dbl)
                        n2340 = local read "water # 4.2R"() -> (w2069:dbl)
                        n2341 = local read "water # 4.1L"() -> (w2070:dbl)
                        n2342 = local read "lick # 4.1L"() -> (w2072:dbl)
                        n2343 = local read "trial #"() -> (w2067:dbl)
                        n2344 = local read "time (s)"() -> (w2073:dbl)
                        n2345 = local read "ITI (s)"() -> (w2065:dbl)
                        n2346 = local read "mistake # 4.1L"() -> (w2063:dbl)
                        n2347 = local read "mistake # 4.2R"() -> (w2062:dbl)
                        n2348 = local read "water dur (ms) 4.2"() -> (w2077:dbl)
                        n2349 = local read "water port 4.2"() -> (w2078:tag)
                        n2350 = local read "Mouse path 4"() -> (w2074:path)
                        n2351 = Build Array(w2073, w2072, w2071, w2070, w2069, w2068, w2068, w2067, w2066, w2065, 1.0 ("element"), w2063, w2062) -> (w2075:dbl[])
                        n2352 = call "_digital_on_duration_off.vi"("duration (ms)"=w2077, "digital port"=w2078) -> ()  [unwired: 10 in]
                        n2353 = call-poly <vilib>:"Write To Spreadsheet File.vi"("append to file? (new file:F)"=TRUE, "1D data"=w2075, "file path (dialog if empty)"=w2074) -> ()  [unwired: 5 in, 1 out]
                      }
                    }
                  }
                  frame 3 {
                    n2354 = case shown="True" w2079 {
                      frame False {
                      }
                      frame True {
                        w2086 = 0.0 ("element")
                        n2355 = local read "water # 4.2R"() -> (w2087:dbl)
                        n2356 = local read "current sound"() -> (w2084:dbl)
                        n2357 = local read "water # 4.1L"() -> (w2088:dbl)
                        n2358 = local read "lick # 4.2R"() -> (w2089:dbl)
                        n2359 = local read "ITI (s)"() -> (w2083:dbl)
                        n2360 = local read "lick # 4.1L"() -> (w2090:dbl)
                        n2361 = local read "trial #"() -> (w2085:dbl)
                        n2362 = local read "mistake # 4.2R"() -> (w2080:dbl)
                        n2363 = local read "mistake # 4.1L"() -> (w2081:dbl)
                        n2364 = local read "time (s)"() -> (w2091:dbl)
                        n2365 = local read "water dur (ms) 4.1"() -> (w2095:dbl)
                        n2366 = local read "water port 4.1"() -> (w2096:tag)
                        n2367 = local read "Mouse path 4"() -> (w2093:path)
                        n2368 = Build Array(w2091, w2090, w2089, w2088, w2087, w2086, w2086, w2085, w2084, w2083, 1.0 ("element"), w2081, w2080) -> (w2092:dbl[])
                        n2369 = call-poly <vilib>:"Write To Spreadsheet File.vi"("append to file? (new file:F)"=TRUE, "1D data"=w2092, "file path (dialog if empty)"=w2093) -> ()  [unwired: 5 in, 1 out]
                        n2370 = call "_digital_on_duration_off.vi"("duration (ms)"=w2095, "digital port"=w2096) -> ()  [unwired: 10 in]
                      }
                    }
                  }
                  frame 4 {
                    n2371 = case shown="True" w2097 {
                      frame False {
                      }
                      frame True {
                        w2104 = 0.0 ("element")
                        n2372 = local read "water # 4.2R"() -> (w2105:dbl)
                        n2373 = local read "water # 4.1L"() -> (w2106:dbl)
                        n2374 = local read "current sound"() -> (w2102:dbl)
                        n2375 = local read "lick # 4.2R"() -> (w2107:dbl)
                        n2376 = local read "lick # 4.1L"() -> (w2108:dbl)
                        n2377 = local read "ITI (s)"() -> (w2101:dbl)
                        n2378 = local read "trial #"() -> (w2103:dbl)
                        n2379 = local read "time (s)"() -> (w2109:dbl)
                        n2380 = local read "mistake # 4.2R"() -> (w2098:dbl)
                        n2381 = local read "mistake # 4.1L"() -> (w2099:dbl)
                        n2382 = local read "water dur (ms) 4.2"() -> (w2113:dbl)
                        n2383 = local read "water port 4.2"() -> (w2114:tag)
                        n2384 = local read "Mouse path 4"() -> (w2111:path)
                        n2385 = Build Array(w2109, w2108, w2107, w2106, w2105, w2104, w2104, w2103, w2102, w2101, 1.0 ("element"), w2099, w2098) -> (w2110:dbl[])
                        n2386 = call-poly <vilib>:"Write To Spreadsheet File.vi"("append to file? (new file:F)"=TRUE, "1D data"=w2110, "file path (dialog if empty)"=w2111) -> ()  [unwired: 5 in, 1 out]
                        n2387 = call "_digital_on_duration_off.vi"("duration (ms)"=w2113, "digital port"=w2114) -> ()  [unwired: 10 in]
                      }
                    }
                  }
                }
              }
              frame #1 {
              }
            }
          }
          frame "graph" {
            n2388 = local read "mistake # 2.2R"() -> (w2366:dbl)
            n2389 = local read "mistake # 3.1L"() -> (w2358:dbl)
            n2390 = local read "mistake # 4.2R"() -> (w2334:dbl)
            n2391 = local read "mistake # 4.1L"() -> (w2342:dbl)
            n2392 = local read "water # 4.2R"() -> (w2335:dbl)
            n2393 = local read "water # 2.2R"() -> (w2367:dbl)
            n2394 = local read "water # 4.2R"() -> (w2336:dbl)
            n2395 = local read "mistake # 2.1L"() -> (w2374:dbl)
            n2396 = local read "water # 3.1L"() -> (w2359:dbl)
            n2397 = local read "water # 2.2R"() -> (w2368:dbl)
            n2398 = local read "water # 4.1L"() -> (w2343:dbl)
            n2399 = local read "water # 2.1L"() -> (w2375:dbl)
            n2400 = local read "water # 3.1L"() -> (w2361:dbl)
            n2401 = local read "mistake # 3.2R"() -> (w2350:dbl)
            n2402 = local read "mistake # 1.2R"() -> (w2383:dbl)
            n2403 = local read "water # 3.2R"() -> (w2351:dbl)
            n2404 = local read "water # 2.1L"() -> (w2376:dbl)
            n2405 = local read "water # 4.1L"() -> (w2345:dbl)
            n2406 = local read "mistake # 1.1L"() -> (w2390:dbl)
            n2407 = local read "water # 3.2R"() -> (w2353:dbl)
            n2408 = local read "water # 1.1L"() -> (w2391:dbl)
            n2409 = local read "water # 1.2R"() -> (w2384:dbl)
            n2410 = local read "water # 1.2R"() -> (w2385:dbl)
            n2411 = local read "water # 1.1L"() -> (w2393:dbl)
            n2412 = Add(x=w2335, y=w2334) -> (x+y=w2333:dbl)
            n2413 = Add(x=w2367, y=w2366) -> (x+y=w2365:dbl)
            n2414 = Add(x=w2375, y=w2374) -> (x+y=w2373:dbl)
            n2415 = Add(x=w2359, y=w2358) -> (x+y=w2357:dbl)
            n2416 = Add(x=w2391, y=w2390) -> (x+y=w2389:dbl)
            n2417 = Add(x=w2351, y=w2350) -> (x+y=w2349:dbl)
            n2418 = Add(x=w2384, y=w2383) -> (x+y=w2382:dbl)
            n2419 = Add(x=w2343, y=w2342) -> (x+y=w2341:dbl)
            n2420 = Divide(x=w2376, y=w2373) -> (x/y=w2377:dbl)
            n2421 = Divide(x=w2353, y=w2349) -> (x/y=w2352:dbl)
            n2422 = Divide(x=w2361, y=w2357) -> (x/y=w2360:dbl)
            n2423 = Divide(x=w2368, y=w2365) -> (x/y=w2369:dbl)
            n2424 = Divide(x=w2385, y=w2382) -> (x/y=w2381:dbl)
            n2425 = Divide(x=w2393, y=w2389) -> (x/y=w2392:dbl)
            n2426 = Divide(x=w2336, y=w2333) -> (x/y=w2337:dbl)
            n2427 = Divide(x=w2345, y=w2341) -> (x/y=w2344:dbl)
            n2428 = local read "time (s)"() -> (w2397:dbl)
            n2429 = call <vilib>:"Mean PtByPt.vi"("x"=w2360) -> ("mean"=w2362:dbl)  [unwired: 3 in, 1 out]
            n2430 = call <vilib>:"Mean PtByPt.vi"("x"=w2352) -> ("mean"=w2354:dbl)  [unwired: 3 in, 1 out]
            n2431 = call <vilib>:"Mean PtByPt.vi"("x"=w2381) -> ("mean"=w2386:dbl)  [unwired: 3 in, 1 out]
            n2432 = call <vilib>:"Mean PtByPt.vi"("x"=w2344) -> ("mean"=w2346:dbl)  [unwired: 3 in, 1 out]
            n2433 = call <vilib>:"Mean PtByPt.vi"("x"=w2337) -> ("mean"=w2332:dbl)  [unwired: 3 in, 1 out]
            n2434 = call <vilib>:"Mean PtByPt.vi"("x"=w2377) -> ("mean"=w2378:dbl)  [unwired: 3 in, 1 out]
            n2435 = call <vilib>:"Mean PtByPt.vi"("x"=w2369) -> ("mean"=w2370:dbl)  [unwired: 3 in, 1 out]
            n2436 = call <vilib>:"Mean PtByPt.vi"("x"=w2392) -> ("mean"=w2394:dbl)  [unwired: 3 in, 1 out]
            n2437 = local write "ratio 1.2R"(w2386) -> ()
            n2438 = local write "ratio 1.1L"(w2394) -> ()
            n2439 = local write "ratio 2.1L"(w2378) -> ()
            n2440 = local write "ratio 3.1L"(w2362) -> ()
            n2441 = local write "ratio 2.2R"(w2370) -> ()
            n2442 = local write "ratio 3.2R"(w2354) -> ()
            n2443 = call "ratio"("Signals"=w2397) -> ("Collected Signals"=w2338:dynamicdata)  [unwired: 9 in, 1 out]
            n2444 = call "ratio1"("Signals"=w2394) -> ("Collected Signals"=w2396:dynamicdata)  [unwired: 9 in, 1 out]
            n2445 = local write "ratio 4.2R"(w2332) -> ()
            n2446 = call "ratio2"("Signals"=w2386) -> ("Collected Signals"=w2388:dynamicdata)  [unwired: 9 in, 1 out]
            n2447 = local write "ratio 4.1L"(w2346) -> ()
            n2448 = call "ratio3"("Signals"=w2378) -> ("Collected Signals"=w2380:dynamicdata)  [unwired: 9 in, 1 out]
            n2449 = call "ratio5"("Signals"=w2362) -> ("Collected Signals"=w2364:dynamicdata)  [unwired: 9 in, 1 out]
            n2450 = call "ratio4"("Signals"=w2370) -> ("Collected Signals"=w2372:dynamicdata)  [unwired: 9 in, 1 out]
            n2451 = call "ratio6"("Signals"=w2354) -> ("Collected Signals"=w2356:dynamicdata)  [unwired: 9 in, 1 out]
            n2452 = call "ratio7"("Signals"=w2346) -> ("Collected Signals"=w2348:dynamicdata)  [unwired: 9 in, 1 out]
            n2453 = call "ratio8"("Signals"=w2332) -> ("Collected Signals"=w2340:dynamicdata)  [unwired: 9 in, 1 out]
            n2454 = call "Build ratio1"("Y Input"=w2396, "X Input"=w2338) -> ("XY Graph"=→"ratio 1.1L":cluster{"Y":dbl[], "Y":dbl[]}[])  [unwired: 3 in, 6 out]
            n2455 = call "Build ratio"("Y Input"=w2388, "X Input"=w2338) -> ("XY Graph"=→"ratio 1.2R":cluster{"Y":dbl[], "Y":dbl[]}[])  [unwired: 3 in, 6 out]
            n2456 = call "Build ratio2"("Y Input"=w2380, "X Input"=w2338) -> ("XY Graph"=→"ratio 2.1L":cluster{"Y":dbl[], "Y":dbl[]}[])  [unwired: 3 in, 6 out]
            n2457 = call "Build ratio4"("Y Input"=w2364, "X Input"=w2338) -> ("XY Graph"=→"ratio 3.1L":cluster{"Y":dbl[], "Y":dbl[]}[])  [unwired: 3 in, 6 out]
            n2458 = call "Build ratio3"("Y Input"=w2372, "X Input"=w2338) -> ("XY Graph"=→"ratio 2.2R":cluster{"Y":dbl[], "Y":dbl[]}[])  [unwired: 3 in, 6 out]
            n2459 = call "Build ratio5"("Y Input"=w2356, "X Input"=w2338) -> ("XY Graph"=→"ratio 3.2R":cluster{"Y":dbl[], "Y":dbl[]}[])  [unwired: 3 in, 6 out]
            n2460 = call "Build ratio6"("Y Input"=w2348, "X Input"=w2338) -> ("XY Graph"=→"ratio 4.1L":cluster{"Y":dbl[], "Y":dbl[]}[])  [unwired: 3 in, 6 out]
            n2461 = call "Build ratio7"("Y Input"=w2340, "X Input"=w2338) -> ("XY Graph"=→"ratio 4.2R":cluster{"Y":dbl[], "Y":dbl[]}[])  [unwired: 3 in, 6 out]
          }
          frame "data collection" {
          }
        }
        n2462 = Wait (ms)(milliseconds to wait=u32 0) -> ()  [unwired: 1 out]
      }
    }
  }
